vi "HandleObservationAsync_old.vi"(8 "error in (no error)":errorcluster, 10 "Acquisition.lvclass In":refnum<class "Acquisition.lvclass">, 11 "S4ACS_GUI in":refnum<class "S4GUI.lvclass">) -> (0 "error out":errorcluster, 2 "Acquisition.lvclass Out":refnum<class "Acquisition.lvclass">, 3 "S4ACS_GUI out":refnum<class "S4GUI.lvclass">)   [LabVIEW 2018, in "S4GUI.lvclass"]
uses:
  S4GUI.lvclass
  Acquisition/Acquisition.lvclass
  C:/Users/devstaff/sparc4/s4gui/Versao ZeroMQ REQ-REP/SPARC4_GUI -20241016_20241016/Server/Server.lvclass
  S4GUI.lvclass/S4GUI.ctl
  Instrument/Instrument.lvclass/Instrument.ctl
  Device/Optics/Optics.lvclass/Optics.ctl
  Interface/Interface.lvclass/Interface.ctl
  Server/Server.lvclass/Server.ctl
  Device/Optics/Opt_Selector/Opt_Selector.lvclass
  C:/Users/devstaff/sparc4/s4gui/Versao ZeroMQ REQ-REP/SPARC4_GUI -20241016_20241016/Device/Optics/Optics.lvclass
  Instrument/Instrument.lvclass
  StateMachine/State Machine.lvclass
  SyncBox/Sync Box.lvclass
  Trigger/Trigger.lvclass
  Channel/Channel.lvclass
  Interface/Interface.lvclass
  TelFocus/TelFocus.lvclass
  SecMirror/SecMirror.lvclass
  Device/Optics/Optics.lvclass
  Server/Server.lvclass
panel:
  out "time308":u32
  out "time307":u32
  out "time9":u32
  out "delay 89":u32
  out "time 10":u32
  out "time elapsed 2":u32
  out "time 8":u32
  out "delay 78":u32
  out "time7":u32
  out "time6":u32
  out "time5":u32
  out "delay 3-4":u32
  out "time4":u32
  out "time3":u32
  out "time 2":u32
  out "time1":u32
  # "ACS DELAY"
  # "WAVEPLATE DURATION"
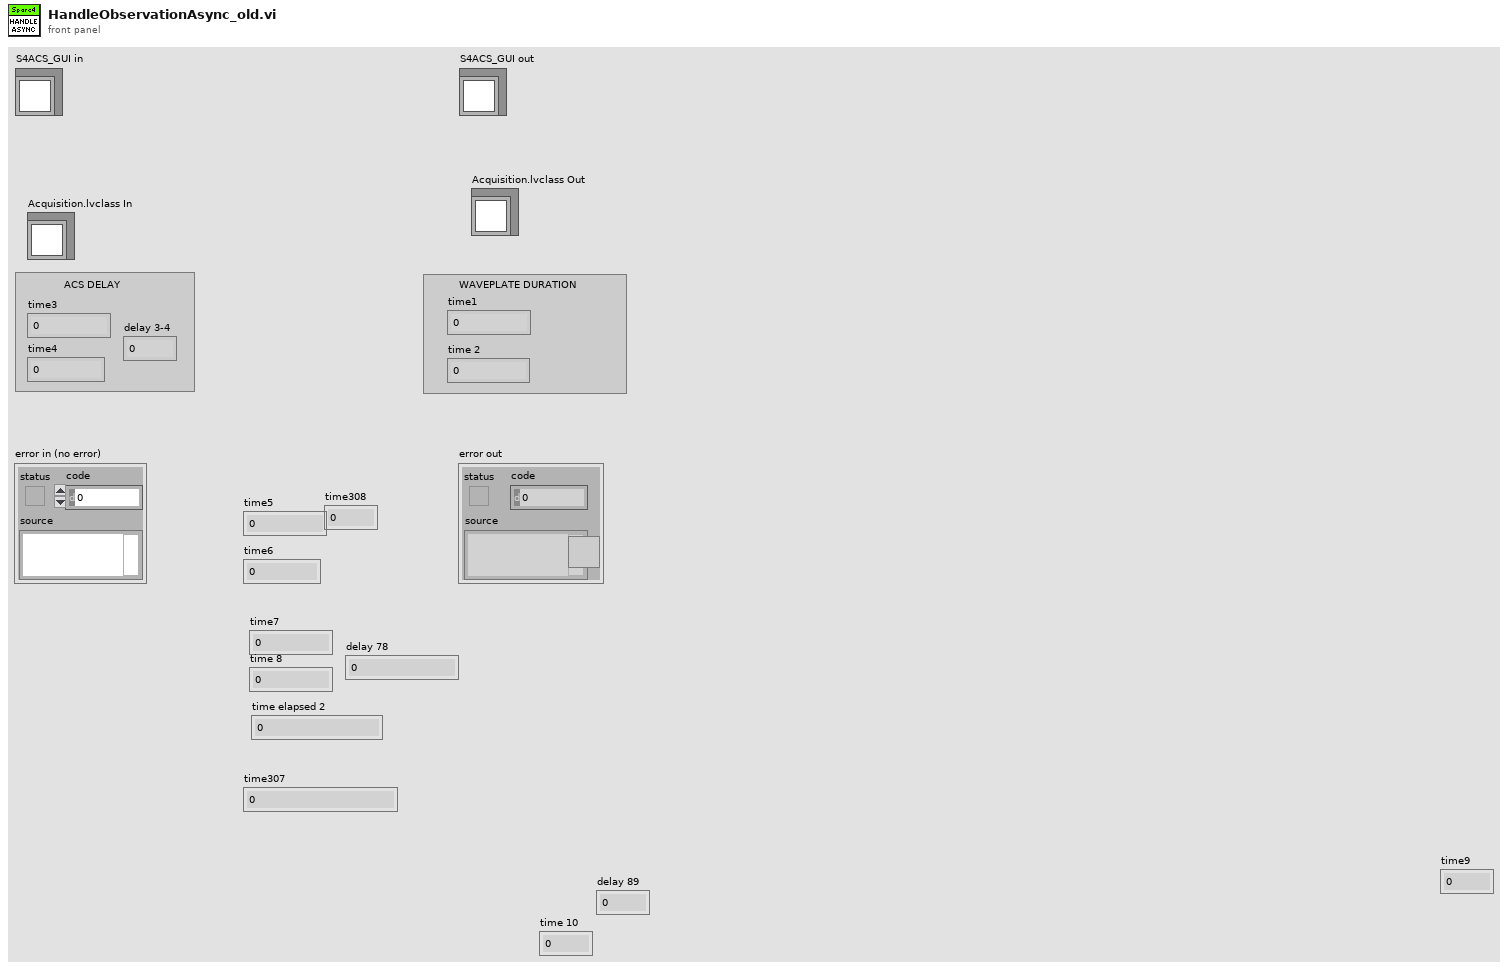
[diagram p1: front panel]
types:
  T1 = cluster{"ACQUISITION_MODE":u8, "TRIGGER_MODE":u8, "READ_MODE":u8, "PREAMP":u8, "READOUT_RATE":u8, "VERTICAL_SHIFT_SPEED":u8, "EM_MODE":u8, "EM_GAIN":u16, "SHUTTER_MODE":u8, "SHUTTER_TTL":u8, "SHUTTER_OPENING_TIME":u16, "SHUTTER_CLOSING_TIME":u16, "VBIN":u16, "HBIN":u16, "INITIAL_LINE":u16, "INITIAL_COLUMN":u16, "FINAL_LINE":u16, "FINAL_COLUMN":u16, "FRAME_TRANSFER":bool, "VERTICAL_CLOCK_VOLTAGE":u8, "AD_CHANNEL":u32}
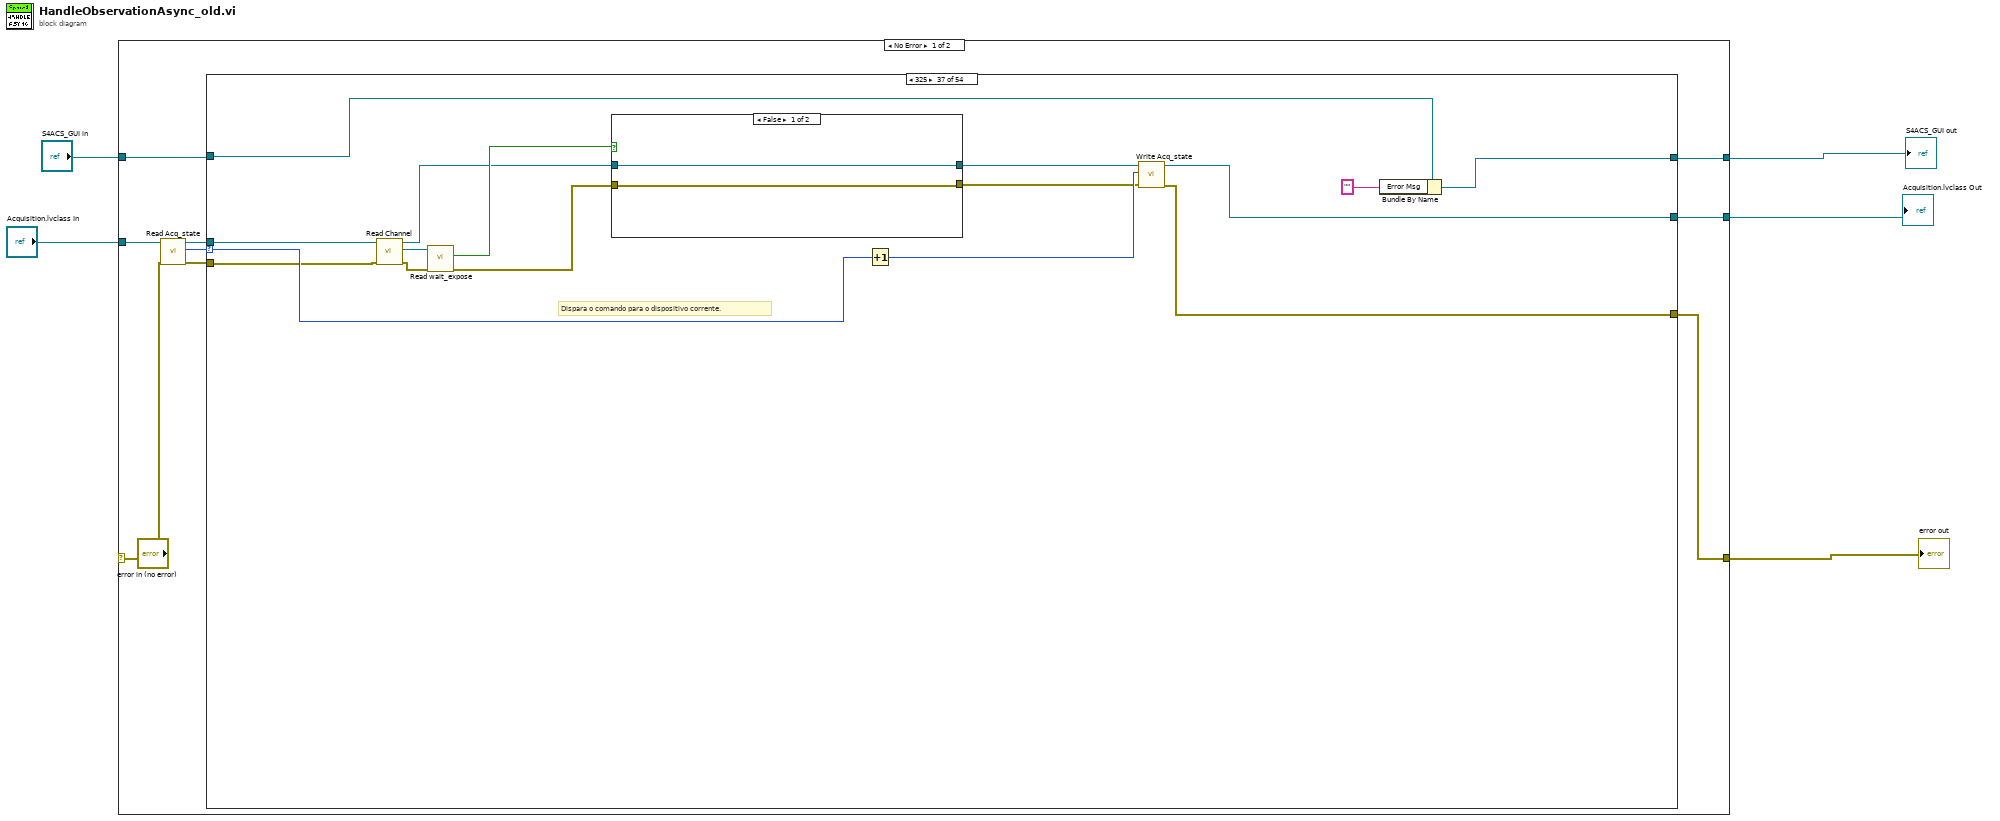
[diagram p0: block diagram]
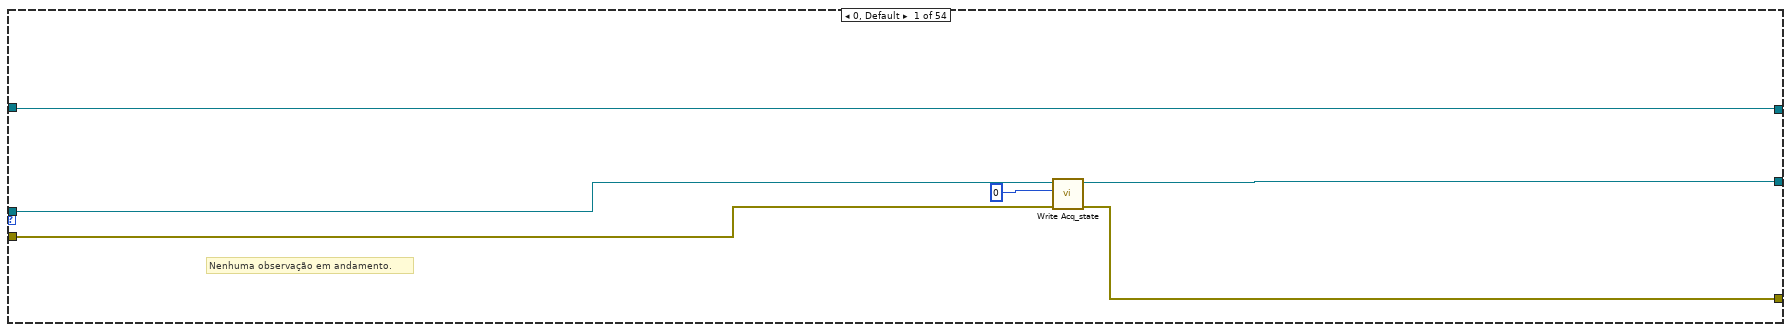
[diagram p2: hidden frame]
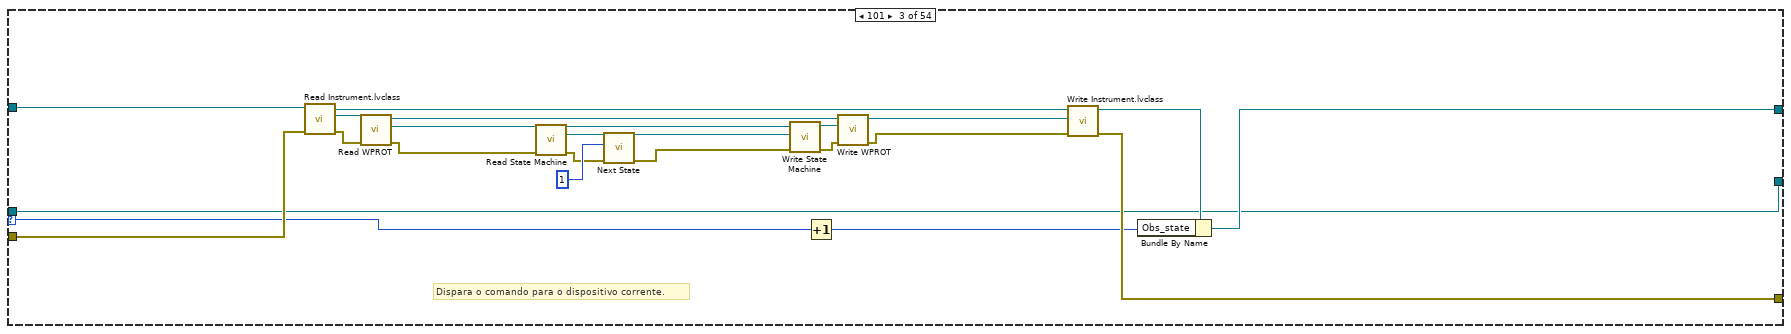
[diagram p4: hidden frame]
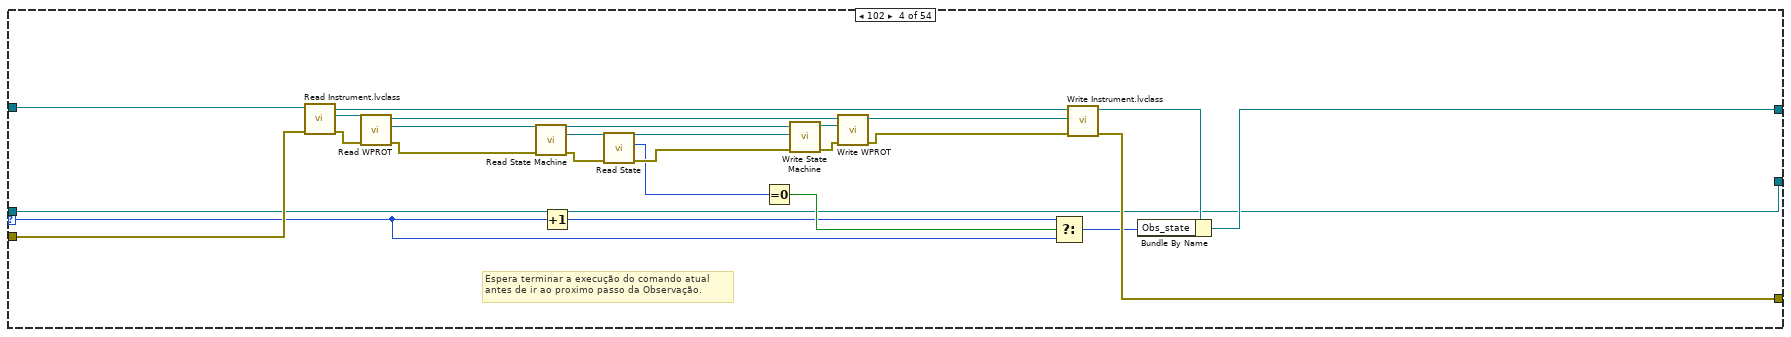
[diagram p5: hidden frame]
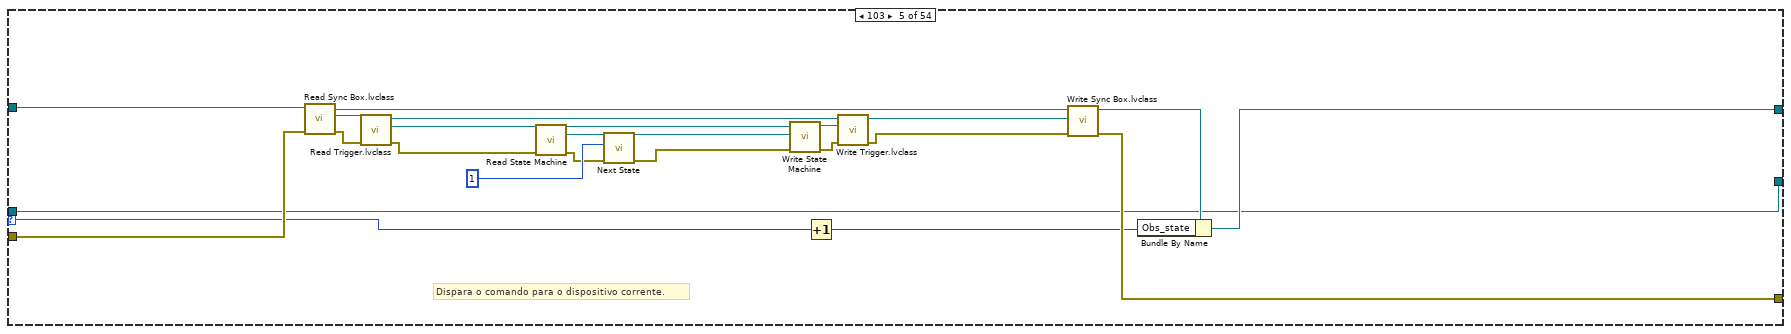
[diagram p6: hidden frame]
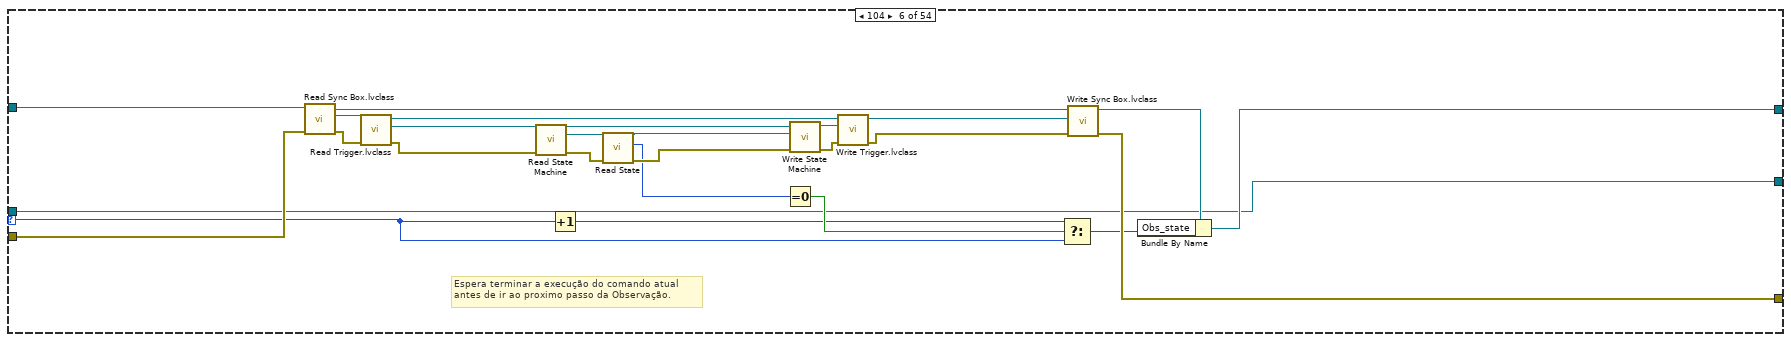
[diagram p7: hidden frame]
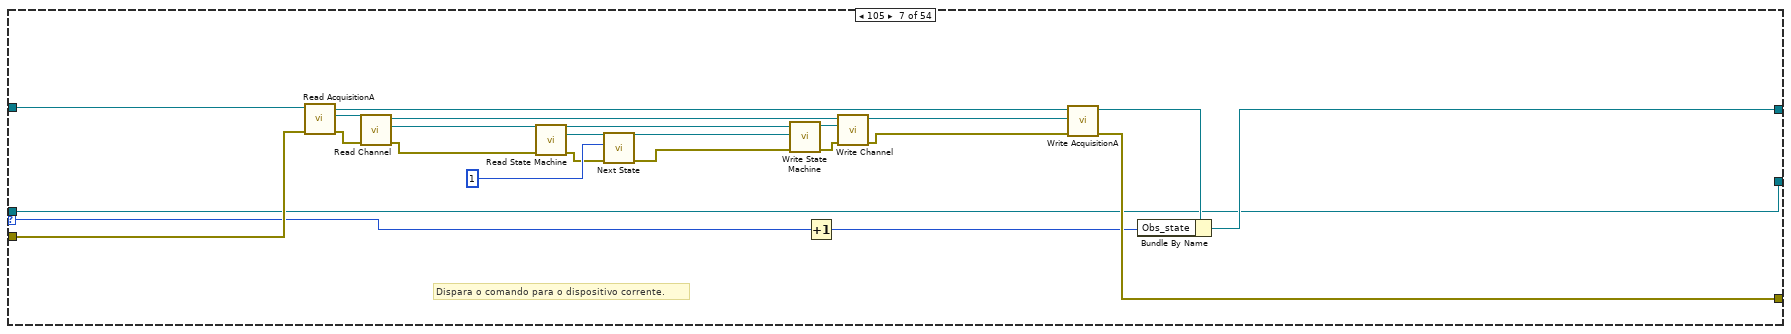
[diagram p8: hidden frame]
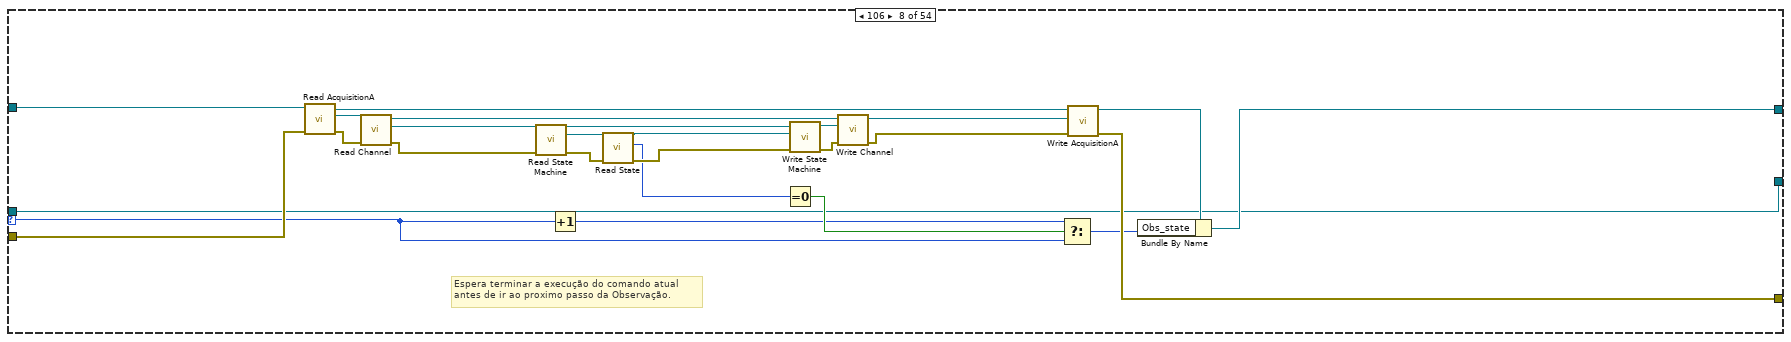
[diagram p9: hidden frame]
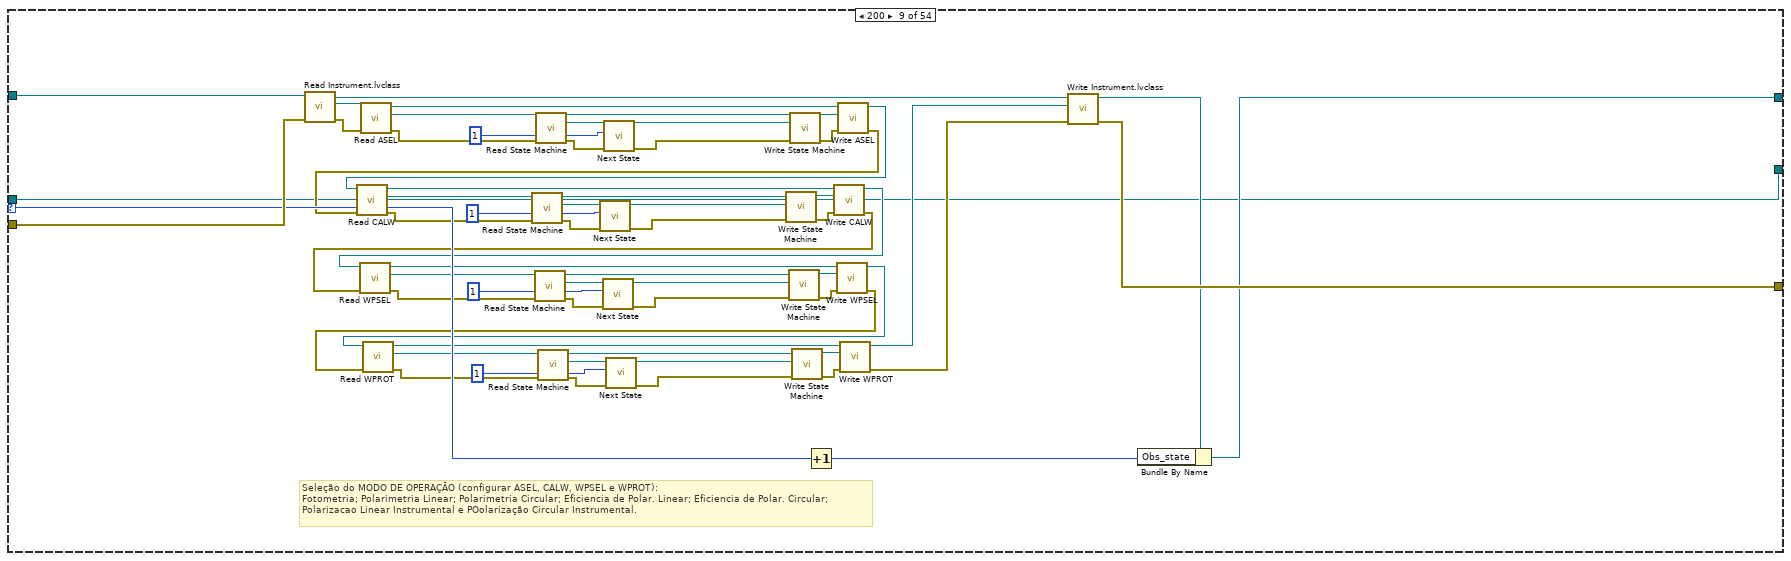
[diagram p10: hidden frame]
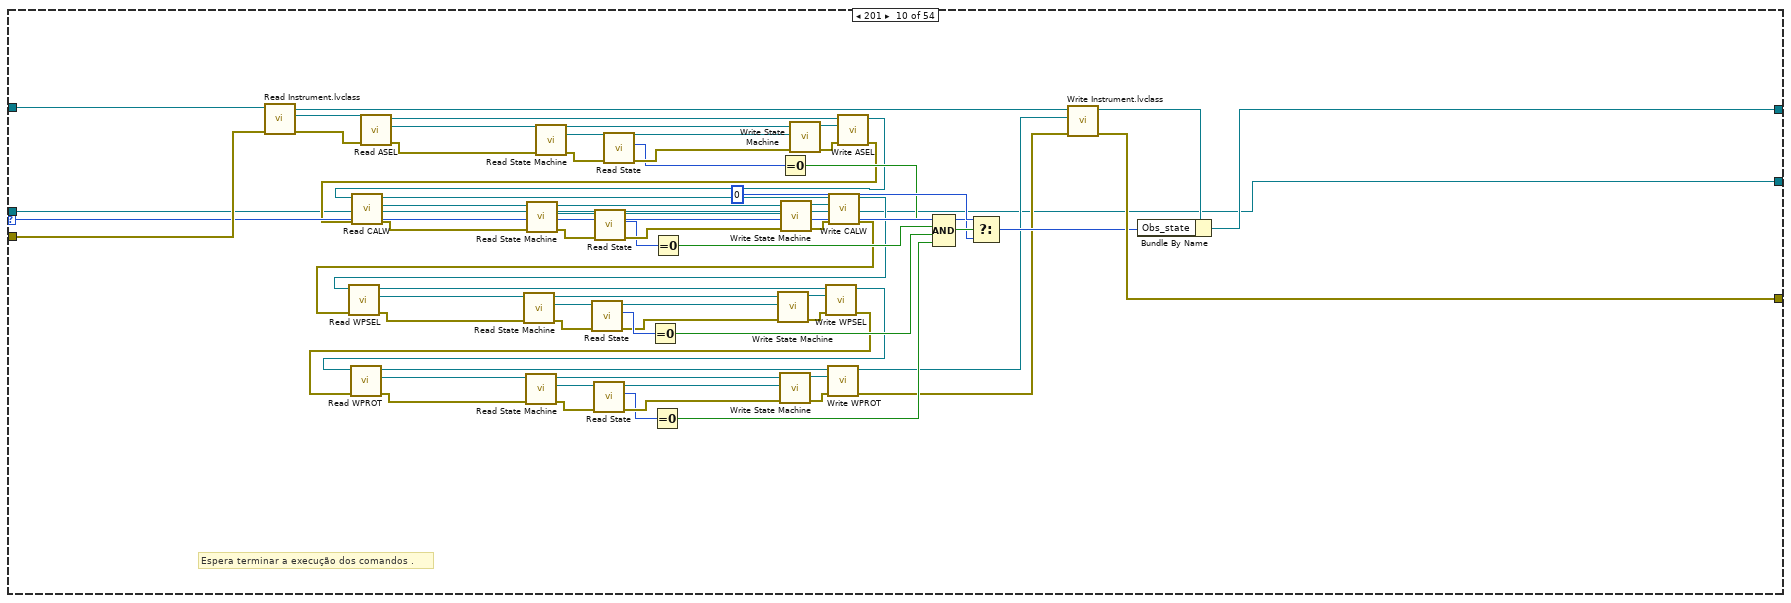
[diagram p11: hidden frame]
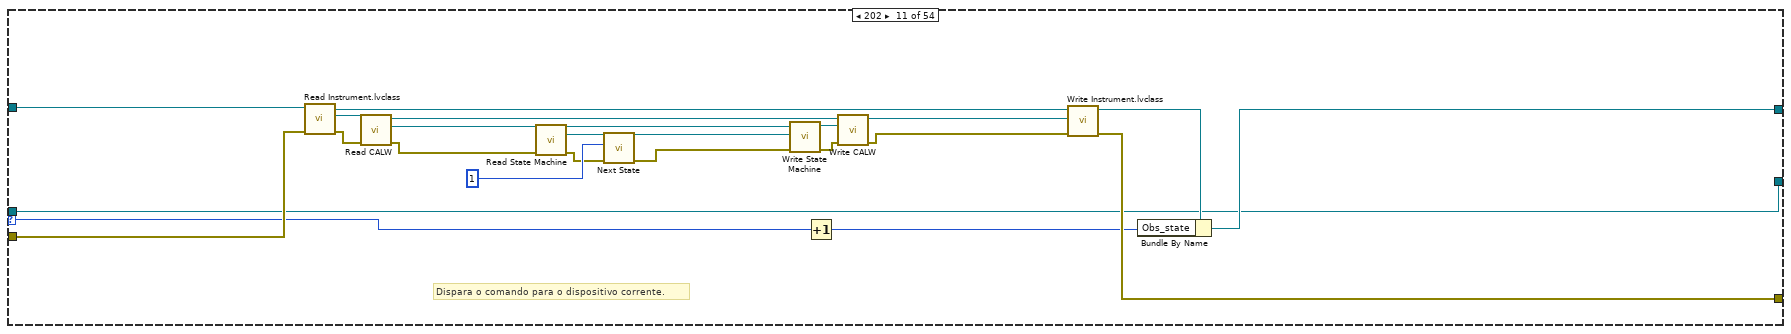
[diagram p12: hidden frame]
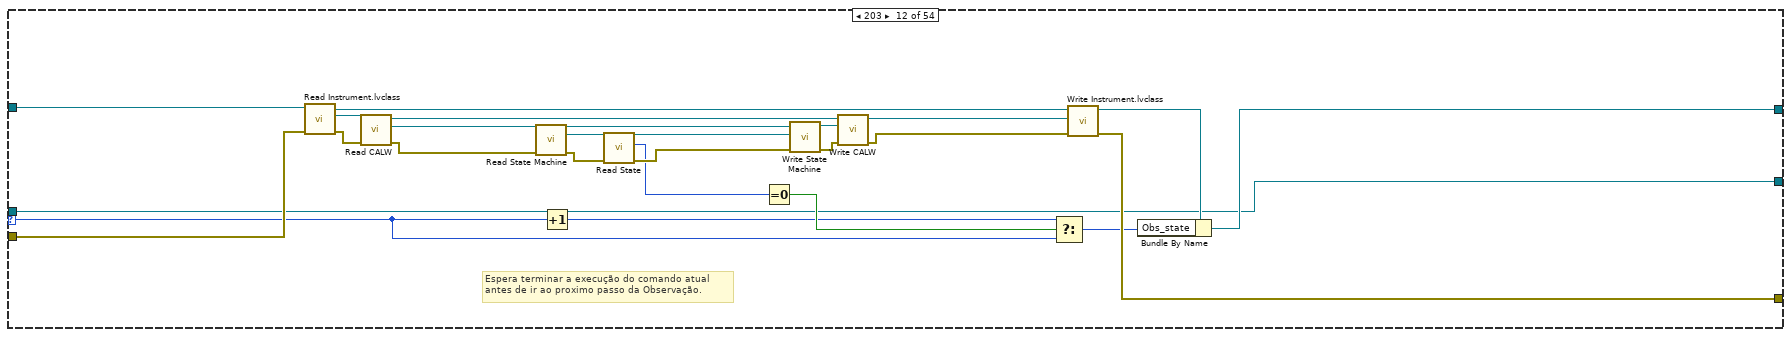
[diagram p13: hidden frame]
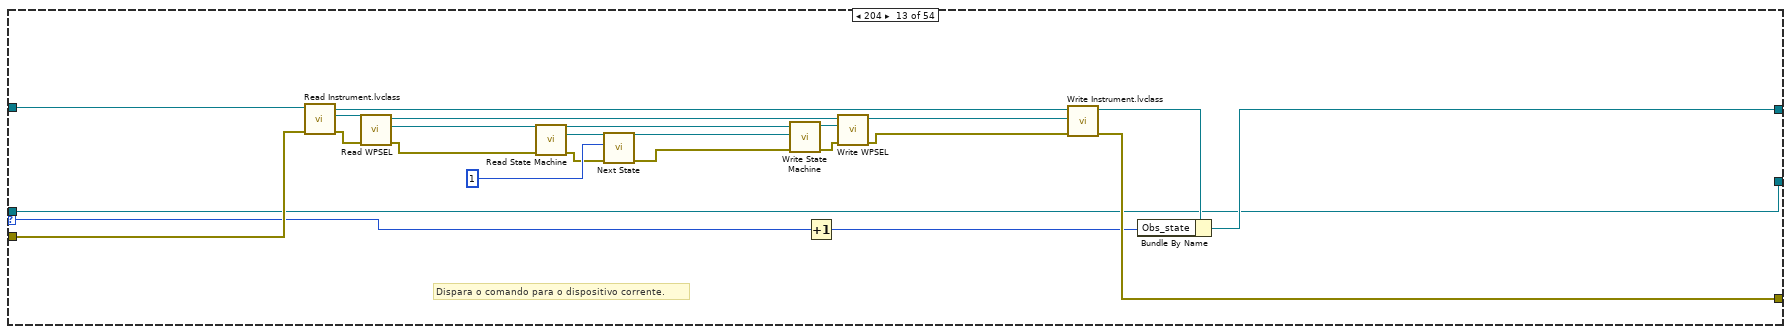
[diagram p14: hidden frame]
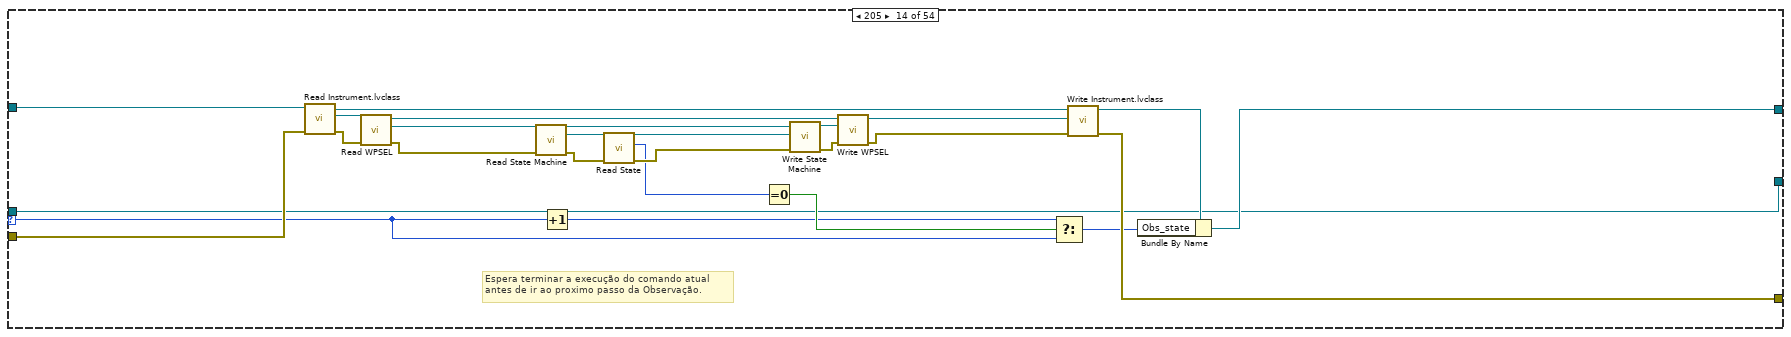
[diagram p15: hidden frame]
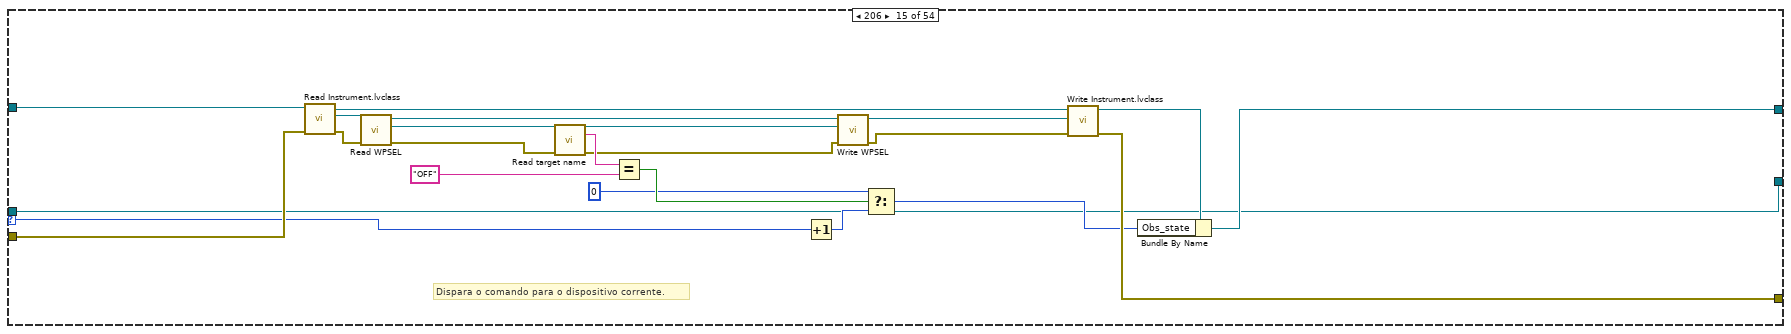
[diagram p16: hidden frame]
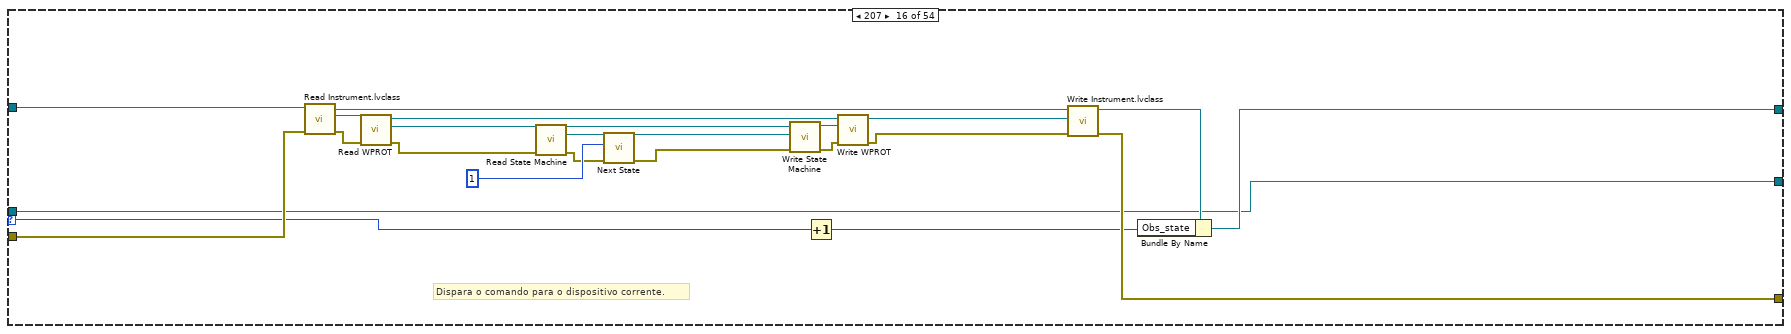
[diagram p17: hidden frame]
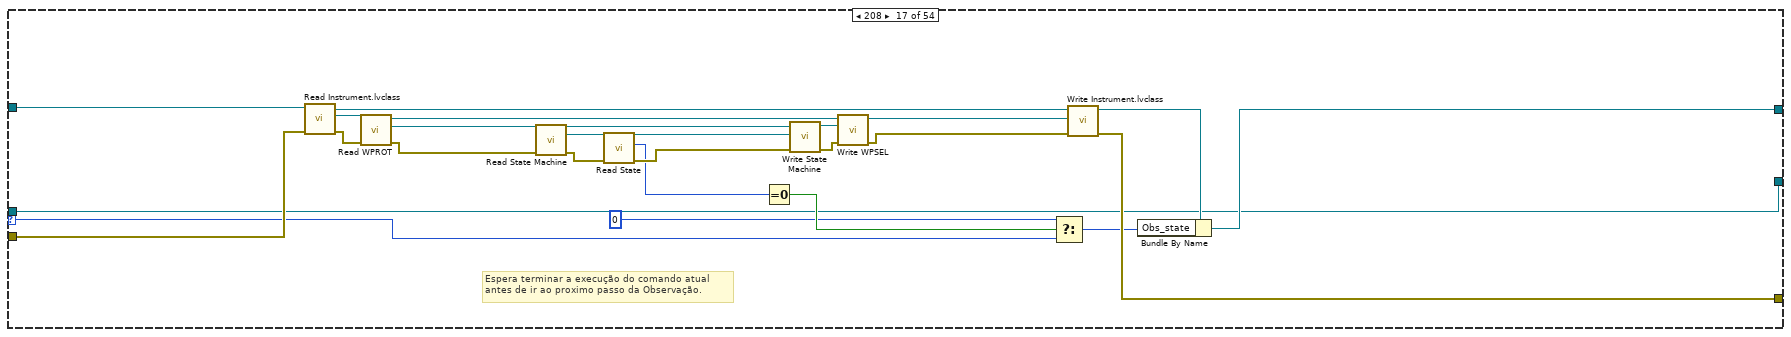
[diagram p18: hidden frame]
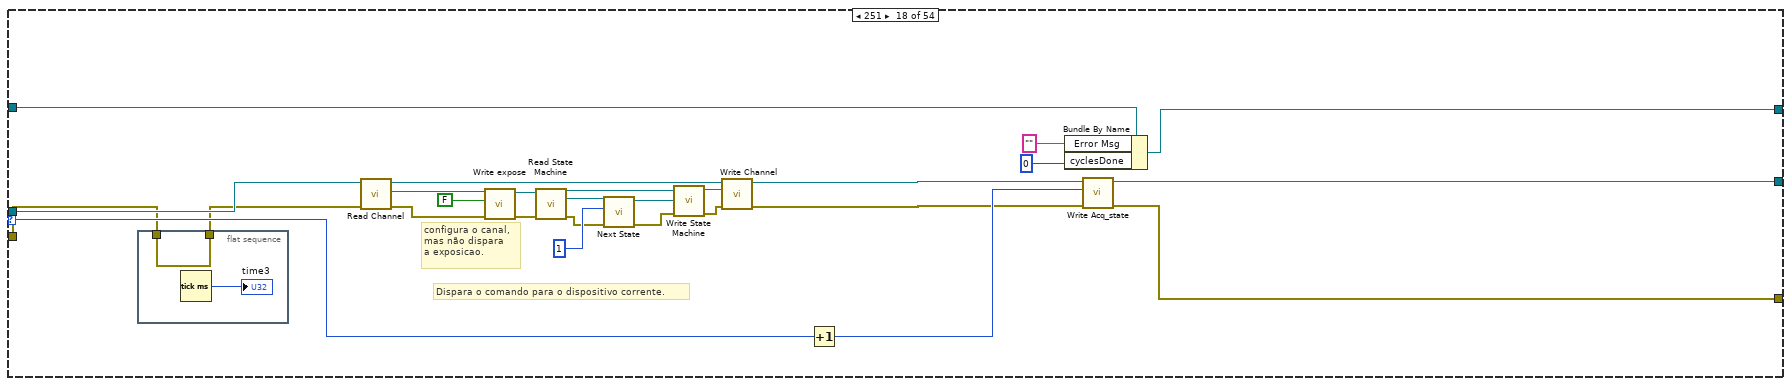
[diagram p19: hidden frame]
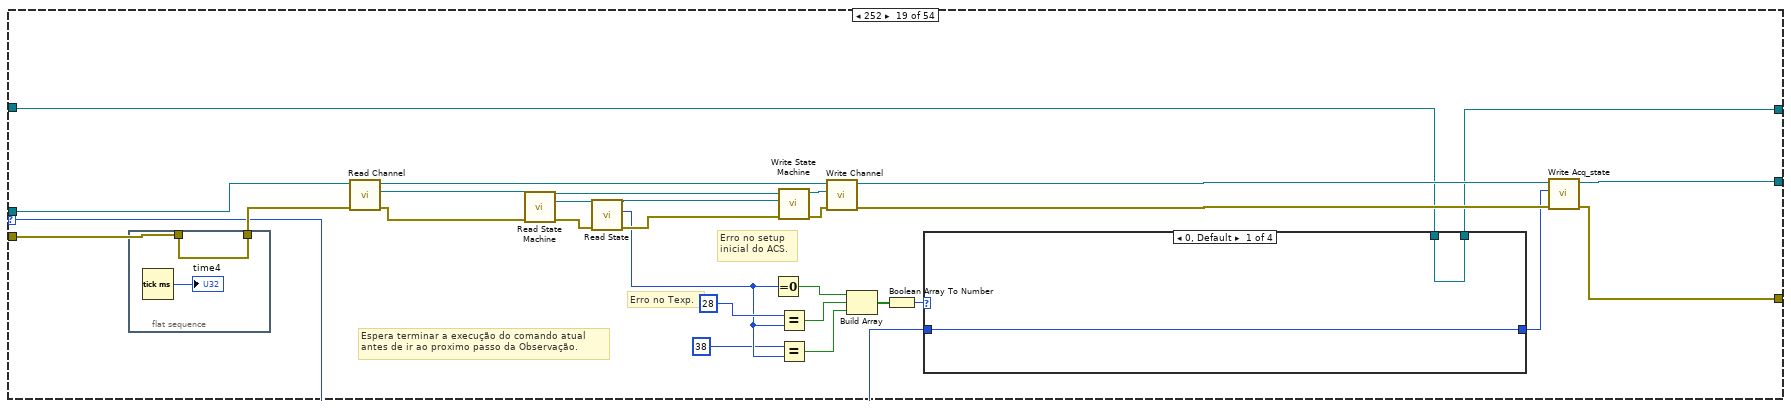
[diagram p20: hidden frame]
diagram:
  n1 = case shown="No Error" "error in (no error)" {
    selector: "error in (no error)" -> [w9 w1768]
    tunnel: [w15 w1768] -> w5
    tunnel: [w14 w1767] -> w3
    tunnel: "S4ACS_GUI in" -> [w13 w1767]
    tunnel: "Acquisition.lvclass In" -> [w12 w1766]
    tunnel: [w7 w1766] -> w1
    frame No Error {
      n2 = call-dynamic "Read Acq_state.vi"("error in (no error)"=w9, "Acquisition in"=w12) -> ("error out"=w8:errorcluster, "Acq_state"=w10:u32, "Acquisition out"=w11:refnum<class "Acquisition.lvclass">)  [unwired: 7 in]
      n3 = case shown="325" w10 {
        selector: w10 -> [_ _ w28 w51 w78 w101 w128 w151 w220 w284 w310 w333 w360 w383 w419 w433 w456 w499 w512 w585 w592 w635 w648 _ w740 w750 w806 w871 w922 w954 w992 _ w1091 w1101 w1129 w1161 w1187 w1207 w1257 w1338 _ w1418 _ w1505 w1554 w1603 w1626 w1642 w1667 w1686 w1711 _ _ _]
        tunnel: w13 -> [w20 w24 w42 w68 w92 w118 w142 w168 w234 w302 w324 w350 w374 w400 w423 w447 w473 w483 w510 w555 w599 w616 w646 w715 w725 w749 w807 w890 w912 w939 w995 w1028 w1081 w1100 w1120 w1144 w1179 w1208 w1252 w1333 w1404 w1417 w1491 w1507 w1556 w1599 w1617 w1648 w1663 w1677 w1704 w1737 w1745 w1748]
        tunnel: [w20 w24 w26 w55 w76 w109 w126 w159 w218 w289 w308 w337 w358 w387 w418 w431 w460 w481 w509 w555 w599 w619 w645 w701 w730 w749 w773 w860 w910 w946 w994 w1027 w1079 w1100 w1119 w1145 w1181 w1211 w1253 w1334 w1404 w1417 w1491 w1504 w1540 w1599 w1621 w1648 w1663 w1681 w1704 w1732 w1745 w1750] -> w14
        tunnel: w8 -> [w19 w23 w41 w67 w91 w117 w141 w167 w233 w301 w323 w349 w373 w399 w422 w446 w472 w485 w522 w556 w593 w622 w658 w706 w724 w763 w770 w877 w920 w934 w1001 w1032 w1089 w1114 w1117 w1155 w1172 w1215 w1237 w1318 w1410 w1421 w1485 w1506 w1555 w1601 w1631 w1645 w1665 w1694 w1724 w1736 w1744 w1747]
        tunnel: [w16 w23 w40 w66 w90 w116 w140 w166 w232 w300 w322 w348 w372 w398 w421 w445 w471 w486 w523 w589 w594 w623 w659 w708 w734 w761 w772 w881 w915 w957 w999 w1029 w1084 w1112 w1123 w1158 w1182 w1218 w1240 w1321 w1415 w1419 w1492 w1498 w1536 w1592 w1627 w1646 w1659 w1690 w1720 w1730 w1744 w1749] -> w15
        tunnel: w11 -> [w18 w22 w25 w49 w75 w99 w125 w149 w175 w238 w307 w331 w357 w381 w407 w430 w454 w491 w527 w588 w600 w627 w663 w700 w739 w764 w775 w859 w921 w961 w1002 w1031 w1090 w1115 w1128 w1154 w1177 w1214 w1238 w1319 w1411 w1422 w1486 w1502 w1539 w1602 w1632 w1643 w1666 w1695 w1725 w1735 w1743 w1746]
        tunnel: [w17 w22 w25 w49 w75 w99 w125 w149 w175 w238 w307 w331 w357 w381 w407 w430 w454 w488 w524 w590 w595 w624 w660 w707 w735 w762 w771 w880 w916 w958 w1000 w1030 w1085 w1113 w1127 w1160 w1186 w1220 w1256 w1337 w1416 w1420 w1493 w1501 w1537 w1596 w1628 w1647 w1660 w1691 w1721 w1731 w1743 w1746] -> w7
        frame 0, Default {
          # "Nenhuma observação em andamento."
          n4 = call-dynamic "Write Acq_state.vi"("error in (no error)"=w19, "Acq_state"=u32 0 ("Obs_state"), "Acquisition in"=w18) -> ("error out"=w16:errorcluster, "Acquisition out"=w17:refnum<class "Acquisition.lvclass">)  [unwired: 7 in]
        }
        frame 1 {
          # "Estado de erro!\nFica aqui até acionar STOP ou ABORT."
          # "Nenhuma observação em andamento."
        }
        frame 101 {
          # "Dispara o comando para o dispositivo corrente."
          n5 = call "Read Instrument.lvclass.vi"("error in (no error)"=w41, "S4ACS_GUI in"=w42) -> ("error out"=w47:errorcluster, "Instrument.lvclass"=w48:refnum<class "Instrument.lvclass">, "S4ACS_GUI out"=w44:refnum<class "S4GUI.lvclass">)  [unwired: 7 in]
          n6 = call "Read WPROT.vi"("error in (no error)"=w47, "Instrument in"=w48) -> ("error out"=w34:errorcluster, "Opt_Selector.lvclass"=w33:refnum<class "Opt_Selector.lvclass">, "Instrument out"=w46:refnum<class "Instrument.lvclass">)  [unwired: 7 in]
          n7 = call-dynamic "Read State Machine.vi"("error in (no error)"=w34, "Device in"=w33) -> ("error out"=w37:errorcluster, "State Machine.lvclass"=w39:refnum<class "State Machine.lvclass">, "Device out"=w31:refnum<class "Opt_Selector.lvclass">)  [unwired: 7 in]
          n8 = call "Next State.vi"("error in (no error)"=w37, "New_State"=1, "State Machine in"=w39) -> ("error out"=w36:errorcluster, "State Machine out"=w35:refnum<class "State Machine.lvclass">)  [unwired: 7 in]
          n9 = call-dynamic "Write State Machine.vi"("error in (no error)"=w36, "State Machine.lvclass"=w35, "Device in"=w31) -> ("error out"=w30:errorcluster, "Device out"=w32:refnum<class "Opt_Selector.lvclass">)  [unwired: 7 in]
          n10 = Increment(x=w28) -> (x+1=w27:u32)
          n11 = call "Write WPROT.vi"("error in (no error)"=w30, "Opt_Selector.lvclass"=w32, "Instrument in"=w46) -> ("error out"=w43:errorcluster, "Instrument out"=w45:refnum<class "Instrument.lvclass">)  [unwired: 7 in]
          n12 = call "Write Instrument.lvclass.vi"("error in (no error)"=w43, "Instrument.lvclass"=w45, "S4ACS_GUI in"=w44) -> ("error out"=w40:errorcluster, "S4ACS_GUI out"=w29:refnum<class "S4GUI.lvclass">)  [unwired: 7 in]
          n13 = Bundle By Name(cluster=w29, "Obs_state"=w27) -> (w26:refnum<class "S4GUI.lvclass">)
        }
        frame 102 {
          # "Espera terminar a execução do comando atual \nantes de ir ao proximo passo da Observação."
          n14 = call "Read Instrument.lvclass.vi"("error in (no error)"=w67, "S4ACS_GUI in"=w68) -> ("error out"=w73:errorcluster, "Instrument.lvclass"=w74:refnum<class "Instrument.lvclass">, "S4ACS_GUI out"=w70:refnum<class "S4GUI.lvclass">)  [unwired: 7 in]
          n15 = call "Read WPROT.vi"("error in (no error)"=w73, "Instrument in"=w74) -> ("error out"=w61:errorcluster, "Opt_Selector.lvclass"=w60:refnum<class "Opt_Selector.lvclass">, "Instrument out"=w72:refnum<class "Instrument.lvclass">)  [unwired: 7 in]
          n16 = call-dynamic "Read State Machine.vi"("error in (no error)"=w61, "Device in"=w60) -> ("error out"=w64:errorcluster, "State Machine.lvclass"=w65:refnum<class "State Machine.lvclass">, "Device out"=w58:refnum<class "Opt_Selector.lvclass">)  [unwired: 7 in]
          n17 = Increment(x=w51) -> (x+1=w50:u32)
          n18 = call-dynamic "Read State.vi"("error in (no error)"=w64, "State Machine in"=w65) -> ("error out"=w63:errorcluster, "State"=w53:i32, "State Machine out"=w62:refnum<class "State Machine.lvclass">)  [unwired: 7 in]
          n19 = Equal To 0?(x=w53) -> (x = 0?=w54:bool)
          n20 = call-dynamic "Write State Machine.vi"("error in (no error)"=w63, "State Machine.lvclass"=w62, "Device in"=w58) -> ("error out"=w57:errorcluster, "Device out"=w59:refnum<class "Opt_Selector.lvclass">)  [unwired: 7 in]
          n21 = call "Write WPROT.vi"("error in (no error)"=w57, "Opt_Selector.lvclass"=w59, "Instrument in"=w72) -> ("error out"=w69:errorcluster, "Instrument out"=w71:refnum<class "Instrument.lvclass">)  [unwired: 7 in]
          n22 = Select(t=w50, s=w54, f=w51) -> (s? t:f=w52:u32)
          n23 = call "Write Instrument.lvclass.vi"("error in (no error)"=w69, "Instrument.lvclass"=w71, "S4ACS_GUI in"=w70) -> ("error out"=w66:errorcluster, "S4ACS_GUI out"=w56:refnum<class "S4GUI.lvclass">)  [unwired: 7 in]
          n24 = Bundle By Name(cluster=w56, "Obs_state"=w52) -> (w55:refnum<class "S4GUI.lvclass">)
        }
        frame 103 {
          # "Dispara o comando para o dispositivo corrente."
          n25 = call-dynamic "Read Sync Box.lvclass.vi"("error in (no error)"=w91, "SPARC4_AC in"=w92) -> ("error out"=w97:errorcluster, "Sync Box.lvclass"=w98:refnum<class "Sync Box.lvclass">, "SPARC4_AC out"=w94:refnum<class "S4GUI.lvclass">)  [unwired: 7 in]
          n26 = call-dynamic "Read Trigger.lvclass.vi"("error in (no error)"=w97, "Sync Box in"=w98) -> ("error out"=w84:errorcluster, "Trigger.lvclass"=w83:refnum<class "Trigger.lvclass">, "Sync Box out"=w96:refnum<class "Sync Box.lvclass">)  [unwired: 7 in]
          n27 = call-dynamic "Read State Machine.vi"("error in (no error)"=w84, "Device in"=w83) -> ("error out"=w87:errorcluster, "State Machine.lvclass"=w89:refnum<class "State Machine.lvclass">, "Device out"=w81:refnum<class "Trigger.lvclass">)  [unwired: 7 in]
          n28 = call "Next State.vi"("error in (no error)"=w87, "New_State"=1, "State Machine in"=w89) -> ("error out"=w86:errorcluster, "State Machine out"=w85:refnum<class "State Machine.lvclass">)  [unwired: 7 in]
          n29 = call-dynamic "Write State Machine.vi"("error in (no error)"=w86, "State Machine.lvclass"=w85, "Device in"=w81) -> ("error out"=w80:errorcluster, "Device out"=w82:refnum<class "Trigger.lvclass">)  [unwired: 7 in]
          n30 = Increment(x=w78) -> (x+1=w77:u32)
          n31 = call-dynamic "Write Trigger.lvclass.vi"("error in (no error)"=w80, "Trigger.lvclass"=w82, "Sync Box in"=w96) -> ("error out"=w93:errorcluster, "Sync Box out"=w95:refnum<class "Sync Box.lvclass">)  [unwired: 7 in]
          n32 = call-dynamic "Write Sync Box.lvclass.vi"("error in (no error)"=w93, "Sync Box.lvclass"=w95, "SPARC4_AC in"=w94) -> ("error out"=w90:errorcluster, "SPARC4_AC out"=w79:refnum<class "S4GUI.lvclass">)  [unwired: 7 in]
          n33 = Bundle By Name(cluster=w79, "Obs_state"=w77) -> (w76:refnum<class "S4GUI.lvclass">)
        }
        frame 104 {
          # "Espera terminar a execução do comando atual \nantes de ir ao proximo passo da Observação."
          n34 = call-dynamic "Read Sync Box.lvclass.vi"("error in (no error)"=w117, "SPARC4_AC in"=w118) -> ("error out"=w123:errorcluster, "Sync Box.lvclass"=w124:refnum<class "Sync Box.lvclass">, "SPARC4_AC out"=w120:refnum<class "S4GUI.lvclass">)  [unwired: 7 in]
          n35 = call-dynamic "Read Trigger.lvclass.vi"("error in (no error)"=w123, "Sync Box in"=w124) -> ("error out"=w115:errorcluster, "Trigger.lvclass"=w114:refnum<class "Trigger.lvclass">, "Sync Box out"=w122:refnum<class "Sync Box.lvclass">)  [unwired: 7 in]
          n36 = call-dynamic "Read State Machine.vi"("error in (no error)"=w115, "Device in"=w114) -> ("error out"=w106:errorcluster, "State Machine.lvclass"=w108:refnum<class "State Machine.lvclass">, "Device out"=w112:refnum<class "Trigger.lvclass">)  [unwired: 7 in]
          n37 = Increment(x=w101) -> (x+1=w103:u32)
          n38 = call-dynamic "Read State.vi"("error in (no error)"=w106, "State Machine in"=w108) -> ("error out"=w105:errorcluster, "State"=w100:i32, "State Machine out"=w107:refnum<class "State Machine.lvclass">)  [unwired: 7 in]
          n39 = Equal To 0?(x=w100) -> (x = 0?=w104:bool)
          n40 = call-dynamic "Write State Machine.vi"("error in (no error)"=w105, "State Machine.lvclass"=w107, "Device in"=w112) -> ("error out"=w111:errorcluster, "Device out"=w113:refnum<class "Trigger.lvclass">)  [unwired: 7 in]
          n41 = call-dynamic "Write Trigger.lvclass.vi"("error in (no error)"=w111, "Trigger.lvclass"=w113, "Sync Box in"=w122) -> ("error out"=w119:errorcluster, "Sync Box out"=w121:refnum<class "Sync Box.lvclass">)  [unwired: 7 in]
          n42 = Select(t=w103, s=w104, f=w101) -> (s? t:f=w102:u32)
          n43 = call-dynamic "Write Sync Box.lvclass.vi"("error in (no error)"=w119, "Sync Box.lvclass"=w121, "SPARC4_AC in"=w120) -> ("error out"=w116:errorcluster, "SPARC4_AC out"=w110:refnum<class "S4GUI.lvclass">)  [unwired: 7 in]
          n44 = Bundle By Name(cluster=w110, "Obs_state"=w102) -> (w109:refnum<class "S4GUI.lvclass">)
        }
        frame 105 {
          # "Dispara o comando para o dispositivo corrente."
          n45 = call-dynamic "Read AcquisitionA.vi"("error in (no error)"=w141, "S4ACS_GUI in"=w142) -> ("error out"=w147:errorcluster, "Acquisition.lvclass"=w148:refnum<class "Acquisition.lvclass">, "S4ACS_GUI out"=w144:refnum<class "S4GUI.lvclass">)  [unwired: 7 in]
          n46 = call-dynamic "Read Channel.vi"("error in (no error)"=w147, "Acquisition in"=w148) -> ("error out"=w134:errorcluster, "Channel.lvclass"=w133:refnum<class "Channel.lvclass">, "Acquisition out"=w146:refnum<class "Acquisition.lvclass">)  [unwired: 7 in]
          n47 = call-dynamic "Read State Machine.vi"("error in (no error)"=w134, "Device in"=w133) -> ("error out"=w137:errorcluster, "State Machine.lvclass"=w139:refnum<class "State Machine.lvclass">, "Device out"=w131:refnum<class "Channel.lvclass">)  [unwired: 7 in]
          n48 = call "Next State.vi"("error in (no error)"=w137, "New_State"=1, "State Machine in"=w139) -> ("error out"=w136:errorcluster, "State Machine out"=w135:refnum<class "State Machine.lvclass">)  [unwired: 7 in]
          n49 = call-dynamic "Write State Machine.vi"("error in (no error)"=w136, "State Machine.lvclass"=w135, "Device in"=w131) -> ("error out"=w130:errorcluster, "Device out"=w132:refnum<class "Channel.lvclass">)  [unwired: 7 in]
          n50 = Increment(x=w128) -> (x+1=w127:u32)
          n51 = call-dynamic "Write Channel.vi"("error in (no error)"=w130, "Channel.lvclass"=w132, "Acquisition in"=w146) -> ("error out"=w143:errorcluster, "Acquisition out"=w145:refnum<class "Acquisition.lvclass">)  [unwired: 7 in]
          n52 = call-dynamic "Write AcquisitionA.vi"("error in (no error)"=w143, "Acquisition.lvclass"=w145, "S4ACS_GUI in"=w144) -> ("error out"=w140:errorcluster, "S4ACS_GUI out"=w129:refnum<class "S4GUI.lvclass">)  [unwired: 7 in]
          n53 = Bundle By Name(cluster=w129, "Obs_state"=w127) -> (w126:refnum<class "S4GUI.lvclass">)
        }
        frame 106 {
          # "Espera terminar a execução do comando atual \nantes de ir ao proximo passo da Observação."
          n54 = call-dynamic "Read AcquisitionA.vi"("error in (no error)"=w167, "S4ACS_GUI in"=w168) -> ("error out"=w173:errorcluster, "Acquisition.lvclass"=w174:refnum<class "Acquisition.lvclass">, "S4ACS_GUI out"=w170:refnum<class "S4GUI.lvclass">)  [unwired: 7 in]
          n55 = call-dynamic "Read Channel.vi"("error in (no error)"=w173, "Acquisition in"=w174) -> ("error out"=w165:errorcluster, "Channel.lvclass"=w164:refnum<class "Channel.lvclass">, "Acquisition out"=w172:refnum<class "Acquisition.lvclass">)  [unwired: 7 in]
          n56 = call-dynamic "Read State Machine.vi"("error in (no error)"=w165, "Device in"=w164) -> ("error out"=w156:errorcluster, "State Machine.lvclass"=w158:refnum<class "State Machine.lvclass">, "Device out"=w162:refnum<class "Channel.lvclass">)  [unwired: 7 in]
          n57 = Increment(x=w151) -> (x+1=w153:u32)
          n58 = call-dynamic "Read State.vi"("error in (no error)"=w156, "State Machine in"=w158) -> ("error out"=w155:errorcluster, "State"=w150:i32, "State Machine out"=w157:refnum<class "State Machine.lvclass">)  [unwired: 7 in]
          n59 = Equal To 0?(x=w150) -> (x = 0?=w154:bool)
          n60 = call-dynamic "Write State Machine.vi"("error in (no error)"=w155, "State Machine.lvclass"=w157, "Device in"=w162) -> ("error out"=w161:errorcluster, "Device out"=w163:refnum<class "Channel.lvclass">)  [unwired: 7 in]
          n61 = call-dynamic "Write Channel.vi"("error in (no error)"=w161, "Channel.lvclass"=w163, "Acquisition in"=w172) -> ("error out"=w169:errorcluster, "Acquisition out"=w171:refnum<class "Acquisition.lvclass">)  [unwired: 7 in]
          n62 = Select(t=w153, s=w154, f=w151) -> (s? t:f=w152:u32)
          n63 = call-dynamic "Write AcquisitionA.vi"("error in (no error)"=w169, "Acquisition.lvclass"=w171, "S4ACS_GUI in"=w170) -> ("error out"=w166:errorcluster, "S4ACS_GUI out"=w160:refnum<class "S4GUI.lvclass">)  [unwired: 7 in]
          n64 = Bundle By Name(cluster=w160, "Obs_state"=w152) -> (w159:refnum<class "S4GUI.lvclass">)
        }
        frame 200 {
          # "Seleção do MODO DE OPERAÇÃO (configurar ASEL, CALW, WPSEL e WPROT): \nFotometria; Polarimetria Linear; Polarimetria Circular; Eficiencia de Polar. Linear; Eficiencia de Polar. Circular;\nPolarizacao Linear Instrumental e POolarização Circular Instrumental."
          n65 = call "Read Instrument.lvclass.vi"("error in (no error)"=w233, "S4ACS_GUI in"=w234) -> ("error out"=w237:errorcluster, "Instrument.lvclass"=w197:refnum<class "Instrument.lvclass">, "S4ACS_GUI out"=w235:refnum<class "S4GUI.lvclass">)  [unwired: 7 in]
          n66 = call "Read ASEL.vi"("error in (no error)"=w237, "Instrument in"=w197) -> ("error out"=w226:errorcluster, "Opt_Selector.lvclass"=w225:refnum<class "Opt_Selector.lvclass">, "Instrument out"=w236:refnum<class "Instrument.lvclass">)  [unwired: 7 in]
          n67 = call-dynamic "Read State Machine.vi"("error in (no error)"=w226, "Device in"=w225) -> ("error out"=w229:errorcluster, "State Machine.lvclass"=w231:refnum<class "State Machine.lvclass">, "Device out"=w223:refnum<class "Opt_Selector.lvclass">)  [unwired: 7 in]
          n68 = call "Next State.vi"("error in (no error)"=w229, "New_State"=1, "State Machine in"=w231) -> ("error out"=w228:errorcluster, "State Machine out"=w227:refnum<class "State Machine.lvclass">)  [unwired: 7 in]
          n69 = call-dynamic "Write State Machine.vi"("error in (no error)"=w228, "State Machine.lvclass"=w227, "Device in"=w223) -> ("error out"=w222:errorcluster, "Device out"=w224:refnum<class "Opt_Selector.lvclass">)  [unwired: 7 in]
          n70 = Increment(x=w220) -> (x+1=w219:u32)
          n71 = call "Write ASEL.vi"("error in (no error)"=w222, "Opt_Selector.lvclass"=w224, "Instrument in"=w236) -> ("error out"=w178:errorcluster, "Instrument out"=w196:refnum<class "Instrument.lvclass">)  [unwired: 7 in]
          n72 = call "Read CALW.vi"("error in (no error)"=w178, "Instrument in"=w196) -> ("error out"=w213:errorcluster, "Opt_Selector.lvclass"=w214:refnum<class "Opt_Selector.lvclass">, "Instrument out"=w195:refnum<class "Instrument.lvclass">)  [unwired: 7 in]
          n73 = call-dynamic "Read State Machine.vi"("error in (no error)"=w213, "Device in"=w214) -> ("error out"=w210:errorcluster, "State Machine.lvclass"=w208:refnum<class "State Machine.lvclass">, "Device out"=w216:refnum<class "Opt_Selector.lvclass">)  [unwired: 7 in]
          n74 = call "Next State.vi"("error in (no error)"=w210, "New_State"=1, "State Machine in"=w208) -> ("error out"=w211:errorcluster, "State Machine out"=w212:refnum<class "State Machine.lvclass">)  [unwired: 7 in]
          n75 = call-dynamic "Write State Machine.vi"("error in (no error)"=w211, "State Machine.lvclass"=w212, "Device in"=w216) -> ("error out"=w217:errorcluster, "Device out"=w215:refnum<class "Opt_Selector.lvclass">)  [unwired: 7 in]
          n76 = call "Write CALW.vi"("error in (no error)"=w217, "Opt_Selector.lvclass"=w215, "Instrument in"=w195) -> ("error out"=w177:errorcluster, "Instrument out"=w194:refnum<class "Instrument.lvclass">)  [unwired: 7 in]
          n77 = call "Read WPSEL.vi"("error in (no error)"=w177, "Instrument in"=w194) -> ("error out"=w202:errorcluster, "Opt_Selector.lvclass"=w201:refnum<class "Opt_Selector.lvclass">, "Instrument out"=w193:refnum<class "Instrument.lvclass">)  [unwired: 7 in]
          n78 = call-dynamic "Read State Machine.vi"("error in (no error)"=w202, "Device in"=w201) -> ("error out"=w205:errorcluster, "State Machine.lvclass"=w207:refnum<class "State Machine.lvclass">, "Device out"=w199:refnum<class "Opt_Selector.lvclass">)  [unwired: 7 in]
          n79 = call "Next State.vi"("error in (no error)"=w205, "New_State"=1, "State Machine in"=w207) -> ("error out"=w204:errorcluster, "State Machine out"=w203:refnum<class "State Machine.lvclass">)  [unwired: 7 in]
          n80 = call-dynamic "Write State Machine.vi"("error in (no error)"=w204, "State Machine.lvclass"=w203, "Device in"=w199) -> ("error out"=w198:errorcluster, "Device out"=w200:refnum<class "Opt_Selector.lvclass">)  [unwired: 7 in]
          n81 = call "Write WPSEL.vi"("error in (no error)"=w198, "Opt_Selector.lvclass"=w200, "Instrument in"=w193) -> ("error out"=w176:errorcluster, "Instrument out"=w182:refnum<class "Instrument.lvclass">)  [unwired: 7 in]
          n82 = call "Read WPROT.vi"("error in (no error)"=w176, "Instrument in"=w182) -> ("error out"=w188:errorcluster, "Opt_Selector.lvclass"=w189:refnum<class "Opt_Selector.lvclass">, "Instrument out"=w181:refnum<class "Instrument.lvclass">)  [unwired: 7 in]
          n83 = call-dynamic "Read State Machine.vi"("error in (no error)"=w188, "Device in"=w189) -> ("error out"=w185:errorcluster, "State Machine.lvclass"=w183:refnum<class "State Machine.lvclass">, "Device out"=w191:refnum<class "Opt_Selector.lvclass">)  [unwired: 7 in]
          n84 = call "Next State.vi"("error in (no error)"=w185, "New_State"=1, "State Machine in"=w183) -> ("error out"=w186:errorcluster, "State Machine out"=w187:refnum<class "State Machine.lvclass">)  [unwired: 7 in]
          n85 = call-dynamic "Write State Machine.vi"("error in (no error)"=w186, "State Machine.lvclass"=w187, "Device in"=w191) -> ("error out"=w192:errorcluster, "Device out"=w190:refnum<class "Opt_Selector.lvclass">)  [unwired: 7 in]
          n86 = call "Write WPROT.vi"("error in (no error)"=w192, "Opt_Selector.lvclass"=w190, "Instrument in"=w181) -> ("error out"=w179:errorcluster, "Instrument out"=w180:refnum<class "Instrument.lvclass">)  [unwired: 7 in]
          n87 = call "Write Instrument.lvclass.vi"("error in (no error)"=w179, "Instrument.lvclass"=w180, "S4ACS_GUI in"=w235) -> ("error out"=w232:errorcluster, "S4ACS_GUI out"=w221:refnum<class "S4GUI.lvclass">)  [unwired: 7 in]
          n88 = Bundle By Name(cluster=w221, "Obs_state"=w219) -> (w218:refnum<class "S4GUI.lvclass">)
        }
        frame 201 {
          # "Espera terminar a execução dos comandos ."
          n89 = call "Read Instrument.lvclass.vi"("error in (no error)"=w301, "S4ACS_GUI in"=w302) -> ("error out"=w305:errorcluster, "Instrument.lvclass"=w306:refnum<class "Instrument.lvclass">, "S4ACS_GUI out"=w303:refnum<class "S4GUI.lvclass">)  [unwired: 7 in]
          n90 = call "Read ASEL.vi"("error in (no error)"=w305, "Instrument in"=w306) -> ("error out"=w295:errorcluster, "Opt_Selector.lvclass"=w294:refnum<class "Opt_Selector.lvclass">, "Instrument out"=w304:refnum<class "Instrument.lvclass">)  [unwired: 7 in]
          n91 = call-dynamic "Read State Machine.vi"("error in (no error)"=w295, "Device in"=w294) -> ("error out"=w298:errorcluster, "State Machine.lvclass"=w299:refnum<class "State Machine.lvclass">, "Device out"=w292:refnum<class "Opt_Selector.lvclass">)  [unwired: 7 in]
          n92 = call-dynamic "Read State.vi"("error in (no error)"=w298, "State Machine in"=w299) -> ("error out"=w297:errorcluster, "State"=w288:i32, "State Machine out"=w296:refnum<class "State Machine.lvclass">)  [unwired: 7 in]
          n93 = Equal To 0?(x=w288) -> (x = 0?=w283:bool)
          n94 = call-dynamic "Write State Machine.vi"("error in (no error)"=w297, "State Machine.lvclass"=w296, "Device in"=w292) -> ("error out"=w291:errorcluster, "Device out"=w293:refnum<class "Opt_Selector.lvclass">)  [unwired: 7 in]
          n95 = call "Write ASEL.vi"("error in (no error)"=w291, "Opt_Selector.lvclass"=w293, "Instrument in"=w304) -> ("error out"=w245:errorcluster, "Instrument out"=w246:refnum<class "Instrument.lvclass">)  [unwired: 7 in]
          n96 = call "Read CALW.vi"("error in (no error)"=w245, "Instrument in"=w246) -> ("error out"=w278:errorcluster, "Opt_Selector.lvclass"=w279:refnum<class "Opt_Selector.lvclass">, "Instrument out"=w249:refnum<class "Instrument.lvclass">)  [unwired: 7 in]
          n97 = call-dynamic "Read State Machine.vi"("error in (no error)"=w278, "Device in"=w279) -> ("error out"=w275:errorcluster, "State Machine.lvclass"=w274:refnum<class "State Machine.lvclass">, "Device out"=w281:refnum<class "Opt_Selector.lvclass">)  [unwired: 7 in]
          n98 = call-dynamic "Read State.vi"("error in (no error)"=w275, "State Machine in"=w274) -> ("error out"=w276:errorcluster, "State"=w273:i32, "State Machine out"=w277:refnum<class "State Machine.lvclass">)  [unwired: 7 in]
          n99 = Equal To 0?(x=w273) -> (x = 0?=w272:bool)
          n100 = call-dynamic "Write State Machine.vi"("error in (no error)"=w276, "State Machine.lvclass"=w277, "Device in"=w281) -> ("error out"=w282:errorcluster, "Device out"=w280:refnum<class "Opt_Selector.lvclass">)  [unwired: 7 in]
          n101 = call "Write CALW.vi"("error in (no error)"=w282, "Opt_Selector.lvclass"=w280, "Instrument in"=w249) -> ("error out"=w243:errorcluster, "Instrument out"=w244:refnum<class "Instrument.lvclass">)  [unwired: 7 in]
          n102 = call "Read WPSEL.vi"("error in (no error)"=w243, "Instrument in"=w244) -> ("error out"=w266:errorcluster, "Opt_Selector.lvclass"=w265:refnum<class "Opt_Selector.lvclass">, "Instrument out"=w248:refnum<class "Instrument.lvclass">)  [unwired: 7 in]
          n103 = call-dynamic "Read State Machine.vi"("error in (no error)"=w266, "Device in"=w265) -> ("error out"=w269:errorcluster, "State Machine.lvclass"=w270:refnum<class "State Machine.lvclass">, "Device out"=w263:refnum<class "Opt_Selector.lvclass">)  [unwired: 7 in]
          n104 = call-dynamic "Read State.vi"("error in (no error)"=w269, "State Machine in"=w270) -> ("error out"=w268:errorcluster, "State"=w271:i32, "State Machine out"=w267:refnum<class "State Machine.lvclass">)  [unwired: 7 in]
          n105 = Equal To 0?(x=w271) -> (x = 0?=w251:bool)
          n106 = call-dynamic "Write State Machine.vi"("error in (no error)"=w268, "State Machine.lvclass"=w267, "Device in"=w263) -> ("error out"=w262:errorcluster, "Device out"=w264:refnum<class "Opt_Selector.lvclass">)  [unwired: 7 in]
          n107 = call "Write WPSEL.vi"("error in (no error)"=w262, "Opt_Selector.lvclass"=w264, "Instrument in"=w248) -> ("error out"=w241:errorcluster, "Instrument out"=w242:refnum<class "Instrument.lvclass">)  [unwired: 7 in]
          n108 = call "Read WPROT.vi"("error in (no error)"=w241, "Instrument in"=w242) -> ("error out"=w257:errorcluster, "Opt_Selector.lvclass"=w258:refnum<class "Opt_Selector.lvclass">, "Instrument out"=w247:refnum<class "Instrument.lvclass">)  [unwired: 7 in]
          n109 = call-dynamic "Read State Machine.vi"("error in (no error)"=w257, "Device in"=w258) -> ("error out"=w254:errorcluster, "State Machine.lvclass"=w253:refnum<class "State Machine.lvclass">, "Device out"=w260:refnum<class "Opt_Selector.lvclass">)  [unwired: 7 in]
          n110 = call-dynamic "Read State.vi"("error in (no error)"=w254, "State Machine in"=w253) -> ("error out"=w255:errorcluster, "State"=w252:i32, "State Machine out"=w256:refnum<class "State Machine.lvclass">)  [unwired: 7 in]
          n111 = Equal To 0?(x=w252) -> (x = 0?=w250:bool)
          n112 = call-dynamic "Write State Machine.vi"("error in (no error)"=w255, "State Machine.lvclass"=w256, "Device in"=w260) -> ("error out"=w261:errorcluster, "Device out"=w259:refnum<class "Opt_Selector.lvclass">)  [unwired: 7 in]
          n113 = call "Write WPROT.vi"("error in (no error)"=w261, "Opt_Selector.lvclass"=w259, "Instrument in"=w247) -> ("error out"=w239:errorcluster, "Instrument out"=w240:refnum<class "Instrument.lvclass">)  [unwired: 7 in]
          n114 = Compound Arithmetic op=AND(w283, w272, w251, w250) -> (w285:bool)
          n115 = Select(t=u32 0, s=w285, f=w284) -> (s? t:f=w287:u32)
          n116 = call "Write Instrument.lvclass.vi"("error in (no error)"=w239, "Instrument.lvclass"=w240, "S4ACS_GUI in"=w303) -> ("error out"=w300:errorcluster, "S4ACS_GUI out"=w290:refnum<class "S4GUI.lvclass">)  [unwired: 7 in]
          n117 = Bundle By Name(cluster=w290, "Obs_state"=w287) -> (w289:refnum<class "S4GUI.lvclass">)
        }
        frame 202 {
          # "Dispara o comando para o dispositivo corrente."
          n118 = call "Read Instrument.lvclass.vi"("error in (no error)"=w323, "S4ACS_GUI in"=w324) -> ("error out"=w329:errorcluster, "Instrument.lvclass"=w330:refnum<class "Instrument.lvclass">, "S4ACS_GUI out"=w326:refnum<class "S4GUI.lvclass">)  [unwired: 7 in]
          n119 = call "Read CALW.vi"("error in (no error)"=w329, "Instrument in"=w330) -> ("error out"=w316:errorcluster, "Opt_Selector.lvclass"=w315:refnum<class "Opt_Selector.lvclass">, "Instrument out"=w328:refnum<class "Instrument.lvclass">)  [unwired: 7 in]
          n120 = call-dynamic "Read State Machine.vi"("error in (no error)"=w316, "Device in"=w315) -> ("error out"=w319:errorcluster, "State Machine.lvclass"=w321:refnum<class "State Machine.lvclass">, "Device out"=w313:refnum<class "Opt_Selector.lvclass">)  [unwired: 7 in]
          n121 = call "Next State.vi"("error in (no error)"=w319, "New_State"=1, "State Machine in"=w321) -> ("error out"=w318:errorcluster, "State Machine out"=w317:refnum<class "State Machine.lvclass">)  [unwired: 7 in]
          n122 = call-dynamic "Write State Machine.vi"("error in (no error)"=w318, "State Machine.lvclass"=w317, "Device in"=w313) -> ("error out"=w312:errorcluster, "Device out"=w314:refnum<class "Opt_Selector.lvclass">)  [unwired: 7 in]
          n123 = Increment(x=w310) -> (x+1=w309:u32)
          n124 = call "Write CALW.vi"("error in (no error)"=w312, "Opt_Selector.lvclass"=w314, "Instrument in"=w328) -> ("error out"=w325:errorcluster, "Instrument out"=w327:refnum<class "Instrument.lvclass">)  [unwired: 7 in]
          n125 = call "Write Instrument.lvclass.vi"("error in (no error)"=w325, "Instrument.lvclass"=w327, "S4ACS_GUI in"=w326) -> ("error out"=w322:errorcluster, "S4ACS_GUI out"=w311:refnum<class "S4GUI.lvclass">)  [unwired: 7 in]
          n126 = Bundle By Name(cluster=w311, "Obs_state"=w309) -> (w308:refnum<class "S4GUI.lvclass">)
        }
        frame 203 {
          # "Espera terminar a execução do comando atual \nantes de ir ao proximo passo da Observação."
          n127 = call "Read Instrument.lvclass.vi"("error in (no error)"=w349, "S4ACS_GUI in"=w350) -> ("error out"=w355:errorcluster, "Instrument.lvclass"=w356:refnum<class "Instrument.lvclass">, "S4ACS_GUI out"=w352:refnum<class "S4GUI.lvclass">)  [unwired: 7 in]
          n128 = call "Read CALW.vi"("error in (no error)"=w355, "Instrument in"=w356) -> ("error out"=w343:errorcluster, "Opt_Selector.lvclass"=w342:refnum<class "Opt_Selector.lvclass">, "Instrument out"=w354:refnum<class "Instrument.lvclass">)  [unwired: 7 in]
          n129 = call-dynamic "Read State Machine.vi"("error in (no error)"=w343, "Device in"=w342) -> ("error out"=w346:errorcluster, "State Machine.lvclass"=w347:refnum<class "State Machine.lvclass">, "Device out"=w340:refnum<class "Opt_Selector.lvclass">)  [unwired: 7 in]
          n130 = Increment(x=w333) -> (x+1=w332:u32)
          n131 = call-dynamic "Read State.vi"("error in (no error)"=w346, "State Machine in"=w347) -> ("error out"=w345:errorcluster, "State"=w335:i32, "State Machine out"=w344:refnum<class "State Machine.lvclass">)  [unwired: 7 in]
          n132 = Equal To 0?(x=w335) -> (x = 0?=w336:bool)
          n133 = call-dynamic "Write State Machine.vi"("error in (no error)"=w345, "State Machine.lvclass"=w344, "Device in"=w340) -> ("error out"=w339:errorcluster, "Device out"=w341:refnum<class "Opt_Selector.lvclass">)  [unwired: 7 in]
          n134 = call "Write CALW.vi"("error in (no error)"=w339, "Opt_Selector.lvclass"=w341, "Instrument in"=w354) -> ("error out"=w351:errorcluster, "Instrument out"=w353:refnum<class "Instrument.lvclass">)  [unwired: 7 in]
          n135 = Select(t=w332, s=w336, f=w333) -> (s? t:f=w334:u32)
          n136 = call "Write Instrument.lvclass.vi"("error in (no error)"=w351, "Instrument.lvclass"=w353, "S4ACS_GUI in"=w352) -> ("error out"=w348:errorcluster, "S4ACS_GUI out"=w338:refnum<class "S4GUI.lvclass">)  [unwired: 7 in]
          n137 = Bundle By Name(cluster=w338, "Obs_state"=w334) -> (w337:refnum<class "S4GUI.lvclass">)
        }
        frame 204 {
          # "Dispara o comando para o dispositivo corrente."
          n138 = call "Read Instrument.lvclass.vi"("error in (no error)"=w373, "S4ACS_GUI in"=w374) -> ("error out"=w379:errorcluster, "Instrument.lvclass"=w380:refnum<class "Instrument.lvclass">, "S4ACS_GUI out"=w376:refnum<class "S4GUI.lvclass">)  [unwired: 7 in]
          n139 = call "Read WPSEL.vi"("error in (no error)"=w379, "Instrument in"=w380) -> ("error out"=w366:errorcluster, "Opt_Selector.lvclass"=w365:refnum<class "Opt_Selector.lvclass">, "Instrument out"=w378:refnum<class "Instrument.lvclass">)  [unwired: 7 in]
          n140 = call-dynamic "Read State Machine.vi"("error in (no error)"=w366, "Device in"=w365) -> ("error out"=w369:errorcluster, "State Machine.lvclass"=w371:refnum<class "State Machine.lvclass">, "Device out"=w363:refnum<class "Opt_Selector.lvclass">)  [unwired: 7 in]
          n141 = call "Next State.vi"("error in (no error)"=w369, "New_State"=1, "State Machine in"=w371) -> ("error out"=w368:errorcluster, "State Machine out"=w367:refnum<class "State Machine.lvclass">)  [unwired: 7 in]
          n142 = call-dynamic "Write State Machine.vi"("error in (no error)"=w368, "State Machine.lvclass"=w367, "Device in"=w363) -> ("error out"=w362:errorcluster, "Device out"=w364:refnum<class "Opt_Selector.lvclass">)  [unwired: 7 in]
          n143 = Increment(x=w360) -> (x+1=w359:u32)
          n144 = call "Write WPSEL.vi"("error in (no error)"=w362, "Opt_Selector.lvclass"=w364, "Instrument in"=w378) -> ("error out"=w375:errorcluster, "Instrument out"=w377:refnum<class "Instrument.lvclass">)  [unwired: 7 in]
          n145 = call "Write Instrument.lvclass.vi"("error in (no error)"=w375, "Instrument.lvclass"=w377, "S4ACS_GUI in"=w376) -> ("error out"=w372:errorcluster, "S4ACS_GUI out"=w361:refnum<class "S4GUI.lvclass">)  [unwired: 7 in]
          n146 = Bundle By Name(cluster=w361, "Obs_state"=w359) -> (w358:refnum<class "S4GUI.lvclass">)
        }
        frame 205 {
          # "Espera terminar a execução do comando atual \nantes de ir ao proximo passo da Observação."
          n147 = call "Read Instrument.lvclass.vi"("error in (no error)"=w399, "S4ACS_GUI in"=w400) -> ("error out"=w405:errorcluster, "Instrument.lvclass"=w406:refnum<class "Instrument.lvclass">, "S4ACS_GUI out"=w402:refnum<class "S4GUI.lvclass">)  [unwired: 7 in]
          n148 = call "Read WPSEL.vi"("error in (no error)"=w405, "Instrument in"=w406) -> ("error out"=w393:errorcluster, "Opt_Selector.lvclass"=w392:refnum<class "Opt_Selector.lvclass">, "Instrument out"=w404:refnum<class "Instrument.lvclass">)  [unwired: 7 in]
          n149 = call-dynamic "Read State Machine.vi"("error in (no error)"=w393, "Device in"=w392) -> ("error out"=w396:errorcluster, "State Machine.lvclass"=w397:refnum<class "State Machine.lvclass">, "Device out"=w390:refnum<class "Opt_Selector.lvclass">)  [unwired: 7 in]
          n150 = Increment(x=w383) -> (x+1=w382:u32)
          n151 = call-dynamic "Read State.vi"("error in (no error)"=w396, "State Machine in"=w397) -> ("error out"=w395:errorcluster, "State"=w385:i32, "State Machine out"=w394:refnum<class "State Machine.lvclass">)  [unwired: 7 in]
          n152 = Equal To 0?(x=w385) -> (x = 0?=w386:bool)
          n153 = call-dynamic "Write State Machine.vi"("error in (no error)"=w395, "State Machine.lvclass"=w394, "Device in"=w390) -> ("error out"=w389:errorcluster, "Device out"=w391:refnum<class "Opt_Selector.lvclass">)  [unwired: 7 in]
          n154 = call "Write WPSEL.vi"("error in (no error)"=w389, "Opt_Selector.lvclass"=w391, "Instrument in"=w404) -> ("error out"=w401:errorcluster, "Instrument out"=w403:refnum<class "Instrument.lvclass">)  [unwired: 7 in]
          n155 = Select(t=w382, s=w386, f=w383) -> (s? t:f=w384:u32)
          n156 = call "Write Instrument.lvclass.vi"("error in (no error)"=w401, "Instrument.lvclass"=w403, "S4ACS_GUI in"=w402) -> ("error out"=w398:errorcluster, "S4ACS_GUI out"=w388:refnum<class "S4GUI.lvclass">)  [unwired: 7 in]
          n157 = Bundle By Name(cluster=w388, "Obs_state"=w384) -> (w387:refnum<class "S4GUI.lvclass">)
        }
        frame 206 {
          # "Dispara o comando para o dispositivo corrente."
          n158 = call "Read Instrument.lvclass.vi"("error in (no error)"=w422, "S4ACS_GUI in"=w423) -> ("error out"=w428:errorcluster, "Instrument.lvclass"=w429:refnum<class "Instrument.lvclass">, "S4ACS_GUI out"=w425:refnum<class "S4GUI.lvclass">)  [unwired: 7 in]
          n159 = call "Read WPSEL.vi"("error in (no error)"=w428, "Instrument in"=w429) -> ("error out"=w416:errorcluster, "Opt_Selector.lvclass"=w417:refnum<class "Opt_Selector.lvclass">, "Instrument out"=w427:refnum<class "Instrument.lvclass">)  [unwired: 7 in]
          n160 = call "Read target name.vi"("error in (no error)"=w416, "Optics in"=w417) -> ("error out"=w410:errorcluster, "target name"=w415:string, "Optics out"=w409:refnum<class "Opt_Selector.lvclass">)  [unwired: 7 in]
          n161 = Equal?(x=w415, y="OFF") -> (x = y?=w413:bool)
          n162 = Increment(x=w419) -> (x+1=w411:u32)
          n163 = call "Write WPSEL.vi"("error in (no error)"=w410, "Opt_Selector.lvclass"=w409, "Instrument in"=w427) -> ("error out"=w424:errorcluster, "Instrument out"=w426:refnum<class "Instrument.lvclass">)  [unwired: 7 in]
          n164 = Select(t=u32 0, s=w413, f=w411) -> (s? t:f=w408:u32)
          n165 = call "Write Instrument.lvclass.vi"("error in (no error)"=w424, "Instrument.lvclass"=w426, "S4ACS_GUI in"=w425) -> ("error out"=w421:errorcluster, "S4ACS_GUI out"=w420:refnum<class "S4GUI.lvclass">)  [unwired: 7 in]
          n166 = Bundle By Name(cluster=w420, "Obs_state"=w408) -> (w418:refnum<class "S4GUI.lvclass">)
        }
        frame 207 {
          # "Dispara o comando para o dispositivo corrente."
          n167 = call "Read Instrument.lvclass.vi"("error in (no error)"=w446, "S4ACS_GUI in"=w447) -> ("error out"=w452:errorcluster, "Instrument.lvclass"=w453:refnum<class "Instrument.lvclass">, "S4ACS_GUI out"=w449:refnum<class "S4GUI.lvclass">)  [unwired: 7 in]
          n168 = call "Read WPROT.vi"("error in (no error)"=w452, "Instrument in"=w453) -> ("error out"=w439:errorcluster, "Opt_Selector.lvclass"=w438:refnum<class "Opt_Selector.lvclass">, "Instrument out"=w451:refnum<class "Instrument.lvclass">)  [unwired: 7 in]
          n169 = call-dynamic "Read State Machine.vi"("error in (no error)"=w439, "Device in"=w438) -> ("error out"=w442:errorcluster, "State Machine.lvclass"=w444:refnum<class "State Machine.lvclass">, "Device out"=w436:refnum<class "Opt_Selector.lvclass">)  [unwired: 7 in]
          n170 = call "Next State.vi"("error in (no error)"=w442, "New_State"=1, "State Machine in"=w444) -> ("error out"=w441:errorcluster, "State Machine out"=w440:refnum<class "State Machine.lvclass">)  [unwired: 7 in]
          n171 = call-dynamic "Write State Machine.vi"("error in (no error)"=w441, "State Machine.lvclass"=w440, "Device in"=w436) -> ("error out"=w435:errorcluster, "Device out"=w437:refnum<class "Opt_Selector.lvclass">)  [unwired: 7 in]
          n172 = Increment(x=w433) -> (x+1=w432:u32)
          n173 = call "Write WPROT.vi"("error in (no error)"=w435, "Opt_Selector.lvclass"=w437, "Instrument in"=w451) -> ("error out"=w448:errorcluster, "Instrument out"=w450:refnum<class "Instrument.lvclass">)  [unwired: 7 in]
          n174 = call "Write Instrument.lvclass.vi"("error in (no error)"=w448, "Instrument.lvclass"=w450, "S4ACS_GUI in"=w449) -> ("error out"=w445:errorcluster, "S4ACS_GUI out"=w434:refnum<class "S4GUI.lvclass">)  [unwired: 7 in]
          n175 = Bundle By Name(cluster=w434, "Obs_state"=w432) -> (w431:refnum<class "S4GUI.lvclass">)
        }
        frame 208 {
          # "Espera terminar a execução do comando atual \nantes de ir ao proximo passo da Observação."
          n176 = call "Read Instrument.lvclass.vi"("error in (no error)"=w472, "S4ACS_GUI in"=w473) -> ("error out"=w478:errorcluster, "Instrument.lvclass"=w479:refnum<class "Instrument.lvclass">, "S4ACS_GUI out"=w475:refnum<class "S4GUI.lvclass">)  [unwired: 7 in]
          n177 = call "Read WPROT.vi"("error in (no error)"=w478, "Instrument in"=w479) -> ("error out"=w466:errorcluster, "Opt_Selector.lvclass"=w465:refnum<class "Opt_Selector.lvclass">, "Instrument out"=w477:refnum<class "Instrument.lvclass">)  [unwired: 7 in]
          n178 = call-dynamic "Read State Machine.vi"("error in (no error)"=w466, "Device in"=w465) -> ("error out"=w469:errorcluster, "State Machine.lvclass"=w470:refnum<class "State Machine.lvclass">, "Device out"=w463:refnum<class "Opt_Selector.lvclass">)  [unwired: 7 in]
          n179 = call-dynamic "Read State.vi"("error in (no error)"=w469, "State Machine in"=w470) -> ("error out"=w468:errorcluster, "State"=w458:i32, "State Machine out"=w467:refnum<class "State Machine.lvclass">)  [unwired: 7 in]
          n180 = Equal To 0?(x=w458) -> (x = 0?=w459:bool)
          n181 = call-dynamic "Write State Machine.vi"("error in (no error)"=w468, "State Machine.lvclass"=w467, "Device in"=w463) -> ("error out"=w462:errorcluster, "Device out"=w464:refnum<class "Opt_Selector.lvclass">)  [unwired: 7 in]
          n182 = call "Write WPSEL.vi"("error in (no error)"=w462, "Opt_Selector.lvclass"=w464, "Instrument in"=w477) -> ("error out"=w474:errorcluster, "Instrument out"=w476:refnum<class "Instrument.lvclass">)  [unwired: 7 in]
          n183 = Select(t=u32 0, s=w459, f=w456) -> (s? t:f=w457:u32)
          n184 = call "Write Instrument.lvclass.vi"("error in (no error)"=w474, "Instrument.lvclass"=w476, "S4ACS_GUI in"=w475) -> ("error out"=w471:errorcluster, "S4ACS_GUI out"=w461:refnum<class "S4GUI.lvclass">)  [unwired: 7 in]
          n185 = Bundle By Name(cluster=w461, "Obs_state"=w457) -> (w460:refnum<class "S4GUI.lvclass">)
        }
        frame 251 {
          # "configura o canal,\nmas não dispara\na exposicao."
          # "Dispara o comando para o dispositivo corrente."
          n186 = flat-sequence {
            tunnel: [w508] -> w484
            tunnel: w485 -> [w508]
            frame #0 {
              n187 = Tick Count (ms)() -> (millisecond timer value=→"time3":u32)
            }
          }
          n188 = call-dynamic "Read Channel.vi"("error in (no error)"=w484, "Acquisition in"=w491) -> ("error out"=w496:errorcluster, "Channel.lvclass"=w498:refnum<class "Channel.lvclass">, "Acquisition out"=w506:refnum<class "Acquisition.lvclass">)  [unwired: 7 in]
          n189 = call-dynamic "Write expose.vi"("error in (no error)"=w496, "expose"=FALSE, "Channel in"=w498) -> ("error out"=w495:errorcluster, "Channel out"=w497:refnum<class "Channel.lvclass">)  [unwired: 7 in]
          n190 = call-dynamic "Read State Machine.vi"("error in (no error)"=w495, "Device in"=w497) -> ("error out"=w503:errorcluster, "State Machine.lvclass"=w505:refnum<class "State Machine.lvclass">, "Device out"=w501:refnum<class "Channel.lvclass">)  [unwired: 7 in]
          n191 = call "Next State.vi"("error in (no error)"=w503, "New_State"=1, "State Machine in"=w505) -> ("error out"=w492:errorcluster, "State Machine out"=w493:refnum<class "State Machine.lvclass">)  [unwired: 7 in]
          n192 = call-dynamic "Write State Machine.vi"("error in (no error)"=w492, "State Machine.lvclass"=w493, "Device in"=w501) -> ("error out"=w500:errorcluster, "Device out"=w502:refnum<class "Channel.lvclass">)  [unwired: 7 in]
          n193 = call-dynamic "Write Channel.vi"("error in (no error)"=w500, "Channel.lvclass"=w502, "Acquisition in"=w506) -> ("error out"=w487:errorcluster, "Acquisition out"=w489:refnum<class "Acquisition.lvclass">)  [unwired: 7 in]
          n194 = Increment(x=w499) -> (x+1=w490:u32)
          n195 = Bundle By Name(cluster=w483, "Error Msg"="", "cyclesDone"=u32 0) -> (w481:refnum<class "S4GUI.lvclass">)
          n196 = call-dynamic "Write Acq_state.vi"("error in (no error)"=w487, "Acq_state"=w490, "Acquisition in"=w489) -> ("error out"=w486:errorcluster, "Acquisition out"=w488:refnum<class "Acquisition.lvclass">)  [unwired: 7 in]
        }
        frame 252 {
          # "Erro no Texp."
          # "Erro no setup\ninicial do ACS."
          # "Espera terminar a execução do comando atual \nantes de ir ao proximo passo da Observação."
          n197 = flat-sequence {
            tunnel: [w553] -> w521
            tunnel: w522 -> [w553]
            frame #0 {
              n198 = Tick Count (ms)() -> (millisecond timer value=→"time4":u32)
            }
          }
          n199 = call-dynamic "Read Channel.vi"("error in (no error)"=w521, "Acquisition in"=w527) -> ("error out"=w536:errorcluster, "Channel.lvclass"=w535:refnum<class "Channel.lvclass">, "Acquisition out"=w537:refnum<class "Acquisition.lvclass">)  [unwired: 7 in]
          n200 = call-dynamic "Read State Machine.vi"("error in (no error)"=w536, "Device in"=w535) -> ("error out"=w529:errorcluster, "State Machine.lvclass"=w531:refnum<class "State Machine.lvclass">, "Device out"=w533:refnum<class "Channel.lvclass">)  [unwired: 7 in]
          n201 = call-dynamic "Read State.vi"("error in (no error)"=w529, "State Machine in"=w531) -> ("error out"=w528:errorcluster, "State"=w519:i32, "State Machine out"=w530:refnum<class "State Machine.lvclass">)  [unwired: 7 in]
          n202 = Equal To 0?(x=w519) -> (x = 0?=w517:bool)
          n203 = call-dynamic "Write State Machine.vi"("error in (no error)"=w528, "State Machine.lvclass"=w530, "Device in"=w533) -> ("error out"=w532:errorcluster, "Device out"=w534:refnum<class "Channel.lvclass">)  [unwired: 7 in]
          n204 = Equal?(x=28, y=w519) -> (x = y?=w516:bool)
          n205 = Equal?(x=38, y=w519) -> (x = y?=w515:bool)
          n206 = call-dynamic "Write Channel.vi"("error in (no error)"=w532, "Channel.lvclass"=w534, "Acquisition in"=w537) -> ("error out"=w526:errorcluster, "Acquisition out"=w525:refnum<class "Acquisition.lvclass">)  [unwired: 7 in]
          n207 = Build Array(w517, w516, w515) -> (w514:bool[])
          n208 = Boolean Array To Number(Boolean array=w514) -> (number=w513:u32)
          n209 = case shown="0, Default" w513 {
            tunnel: w512 -> [w539 _ _ _]
            tunnel: [w539 u32 300 ("t") u32 1 ("t") u32 1 ("t")] -> w511
            tunnel: w510 -> [w538 w542 w547 w551]
            tunnel: [w538 w541 w546 w550] -> w509
            frame 0, Default {
            }
            frame 1 {
              n210 = Tick Count (ms)() -> (millisecond timer value=→"time307":u32)
              n211 = Bundle By Name(cluster=w542, "Error Msg"="") -> (w541:refnum<class "S4GUI.lvclass">)
            }
            frame 2 {
              n212 = Bundle By Name(cluster=w547, "Error Msg"="ERROR: Some channel initialization failed. S4GUI:HandleObservationAsync.vi state 252.") -> (w546:refnum<class "S4GUI.lvclass">)
            }
            frame 4 {
              n213 = Bundle By Name(cluster=w551, "Error Msg"="ERROR: Some channel with invalid Exposition Time. S4GUI:HandleObservationAsync.vi state 252.") -> (w550:refnum<class "S4GUI.lvclass">)
            }
          }
          n214 = call-dynamic "Write Acq_state.vi"("error in (no error)"=w526, "Acq_state"=w511, "Acquisition in"=w525) -> ("error out"=w523:errorcluster, "Acquisition out"=w524:refnum<class "Acquisition.lvclass">)  [unwired: 7 in]
        }
        frame 253 {
          # "Sem syncbox, \ntrigger mode = 0 (internal)"
          n215 = call-dynamic "Read Channel.vi"("error in (no error)"=w556, "Acquisition in"=w588) -> ("error out"=w561:errorcluster, "Channel.lvclass"=w560:refnum<class "Channel.lvclass">, "Acquisition out"=w583:refnum<class "Acquisition.lvclass">)  [unwired: 7 in]
          n216 = call-dynamic "Read Interface.vi"("error in (no error)"=w561, "Channel in"=w560) -> ("error out"=w559:errorcluster, "Interface.lvclass"=w565:refnum<class "Interface.lvclass">, "Channel out"=w564:refnum<class "Channel.lvclass">)  [unwired: 7 in]
          n217 = call-dynamic "Get CCD_Config.vi"("error in (no error)"=w559, "Interface in"=w565) -> ("error out"=w572:errorcluster, "output cluster"=w574:T1, "Interface out"=w571:refnum<class "Interface.lvclass">)  [unwired: 7 in]
          n218 = Bundle By Name(cluster=w574, "TRIGGER_MODE"=u8 0) -> (w570:T1)
          n219 = call-dynamic "Set CCD_Config.vi"("error in (no error)"=w572, "input cluster"=w570, "Interface in"=w571) -> ("error out"=w568:errorcluster, "Interface out"=w566:refnum<class "Interface.lvclass">)  [unwired: 7 in]
          n220 = Flatten To String(anything=w570, error in (no error)=w568) -> (data string=w569:string, error out=w567:errorcluster)  [unwired: 2 in, 1 out]
          n221 = call "Write flatted cluster.vi"("error in (no error)"=w567, "flatted cluster"=w569, "Interface in"=w566) -> ("error out"=w562:errorcluster, "Interface out"=w563:refnum<class "Interface.lvclass">)  [unwired: 7 in]
          n222 = call-dynamic "Write Interface.vi"("error in (no error)"=w562, "Interface.lvclass"=w563, "Channel in"=w564) -> ("error out"=w558:errorcluster, "Channel out"=w557:refnum<class "Channel.lvclass">)  [unwired: 7 in]
          n223 = call-dynamic "Read State Machine.vi"("error in (no error)"=w558, "Device in"=w557) -> ("error out"=w580:errorcluster, "State Machine.lvclass"=w582:refnum<class "State Machine.lvclass">, "Device out"=w578:refnum<class "Channel.lvclass">)  [unwired: 7 in]
          n224 = Increment(x=w585) -> (x+1=w586:u32)
          n225 = call "Next State.vi"("error in (no error)"=w580, "New_State"=60, "State Machine in"=w582) -> ("error out"=w575:errorcluster, "State Machine out"=w576:refnum<class "State Machine.lvclass">)  [unwired: 7 in]
          n226 = call-dynamic "Write State Machine.vi"("error in (no error)"=w575, "State Machine.lvclass"=w576, "Device in"=w578) -> ("error out"=w577:errorcluster, "Device out"=w579:refnum<class "Channel.lvclass">)  [unwired: 7 in]
          n227 = call-dynamic "Write Channel.vi"("error in (no error)"=w577, "Channel.lvclass"=w579, "Acquisition in"=w583) -> ("error out"=w584:errorcluster, "Acquisition out"=w587:refnum<class "Acquisition.lvclass">)  [unwired: 7 in]
          n228 = call-dynamic "Write Acq_state.vi"("error in (no error)"=w584, "Acq_state"=w586, "Acquisition in"=w587) -> ("error out"=w589:errorcluster, "Acquisition out"=w590:refnum<class "Acquisition.lvclass">)  [unwired: 7 in]
        }
        frame 254 {
          # "Espera terminar a execução do comando atual \nantes de ir ao proximo passo da Observação."
          n229 = call-dynamic "Read Channel.vi"("error in (no error)"=w593, "Acquisition in"=w600) -> ("error out"=w611:errorcluster, "Channel.lvclass"=w610:refnum<class "Channel.lvclass">, "Acquisition out"=w612:refnum<class "Acquisition.lvclass">)  [unwired: 7 in]
          n230 = call-dynamic "Read State Machine.vi"("error in (no error)"=w611, "Device in"=w610) -> ("error out"=w604:errorcluster, "State Machine.lvclass"=w606:refnum<class "State Machine.lvclass">, "Device out"=w608:refnum<class "Channel.lvclass">)  [unwired: 7 in]
          n231 = call-dynamic "Read State.vi"("error in (no error)"=w604, "State Machine in"=w606) -> ("error out"=w603:errorcluster, "State"=w601:i32, "State Machine out"=w605:refnum<class "State Machine.lvclass">)  [unwired: 7 in]
          n232 = Equal To 0?(x=w601) -> (x = 0?=w602:bool)
          n233 = call-dynamic "Write State Machine.vi"("error in (no error)"=w603, "State Machine.lvclass"=w605, "Device in"=w608) -> ("error out"=w607:errorcluster, "Device out"=w609:refnum<class "Channel.lvclass">)  [unwired: 7 in]
          n234 = call-dynamic "Write Channel.vi"("error in (no error)"=w607, "Channel.lvclass"=w609, "Acquisition in"=w612) -> ("error out"=w597:errorcluster, "Acquisition out"=w596:refnum<class "Acquisition.lvclass">)  [unwired: 7 in]
          n235 = Select(t=u32 299, s=w602, f=w592) -> (s? t:f=w598:u32)
          n236 = call-dynamic "Write Acq_state.vi"("error in (no error)"=w597, "Acq_state"=w598, "Acquisition in"=w596) -> ("error out"=w594:errorcluster, "Acquisition out"=w595:refnum<class "Acquisition.lvclass">)  [unwired: 7 in]
        }
        frame 271 {
          # "configura o canal,\nmas não dispara\na exposicao."
          # "Dispara o comando para o dispositivo corrente."
          n237 = flat-sequence {
            tunnel: [w644] -> w621
            tunnel: w622 -> [w644]
            frame #0 {
              n238 = Tick Count (ms)() -> (millisecond timer value=→"time5":u32)
            }
          }
          n239 = call-dynamic "Read Channel.vi"("error in (no error)"=w621, "Acquisition in"=w627) -> ("error out"=w632:errorcluster, "Channel.lvclass"=w634:refnum<class "Channel.lvclass">, "Acquisition out"=w642:refnum<class "Acquisition.lvclass">)  [unwired: 7 in]
          n240 = call-dynamic "Write expose.vi"("error in (no error)"=w632, "expose"=FALSE, "Channel in"=w634) -> ("error out"=w631:errorcluster, "Channel out"=w633:refnum<class "Channel.lvclass">)  [unwired: 7 in]
          n241 = call-dynamic "Read State Machine.vi"("error in (no error)"=w631, "Device in"=w633) -> ("error out"=w639:errorcluster, "State Machine.lvclass"=w641:refnum<class "State Machine.lvclass">, "Device out"=w637:refnum<class "Channel.lvclass">)  [unwired: 7 in]
          n242 = call "Next State.vi"("error in (no error)"=w639, "New_State"=1, "State Machine in"=w641) -> ("error out"=w628:errorcluster, "State Machine out"=w629:refnum<class "State Machine.lvclass">)  [unwired: 7 in]
          n243 = call-dynamic "Write State Machine.vi"("error in (no error)"=w628, "State Machine.lvclass"=w629, "Device in"=w637) -> ("error out"=w636:errorcluster, "Device out"=w638:refnum<class "Channel.lvclass">)  [unwired: 7 in]
          n244 = call-dynamic "Write Channel.vi"("error in (no error)"=w636, "Channel.lvclass"=w638, "Acquisition in"=w642) -> ("error out"=w614:errorcluster, "Acquisition out"=w625:refnum<class "Acquisition.lvclass">)  [unwired: 7 in]
          n245 = Increment(x=w635) -> (x+1=w626:u32)
          n246 = Unbundle By Name(w616) -> ("TelFocus.lvclass"=w618:refnum<class "TelFocus.lvclass">)
          n247 = call-dynamic "Write focus #stepsdone.vi"("error in (no error)"=w614, "focus #stepsdone"=u32 0, "TelFocus in"=w618) -> ("error out"=w613:errorcluster, "TelFocus out"=w615:refnum<class "TelFocus.lvclass">)  [unwired: 7 in]
          n248 = Bundle By Name(cluster=w616, "TelFocus.lvclass"=w615, "Error Msg"="") -> (w619:refnum<class "S4GUI.lvclass">)
          n249 = call-dynamic "Write Acq_state.vi"("error in (no error)"=w613, "Acq_state"=w626, "Acquisition in"=w625) -> ("error out"=w623:errorcluster, "Acquisition out"=w624:refnum<class "Acquisition.lvclass">)  [unwired: 7 in]
        }
        frame 272 {
          # "Erro no Texp."
          # "Erro no setup\ninicial do ACS."
          # "Espera terminar a execução do comando atual \nantes de ir ao proximo passo da Observação."
          n250 = flat-sequence {
            tunnel: [w688] -> w657
            tunnel: w658 -> [w688]
            frame #0 {
              n251 = Tick Count (ms)() -> (millisecond timer value=→"time6":u32)
            }
          }
          n252 = call-dynamic "Read Channel.vi"("error in (no error)"=w657, "Acquisition in"=w663) -> ("error out"=w672:errorcluster, "Channel.lvclass"=w671:refnum<class "Channel.lvclass">, "Acquisition out"=w673:refnum<class "Acquisition.lvclass">)  [unwired: 7 in]
          n253 = call-dynamic "Read State Machine.vi"("error in (no error)"=w672, "Device in"=w671) -> ("error out"=w665:errorcluster, "State Machine.lvclass"=w667:refnum<class "State Machine.lvclass">, "Device out"=w669:refnum<class "Channel.lvclass">)  [unwired: 7 in]
          n254 = call-dynamic "Read State.vi"("error in (no error)"=w665, "State Machine in"=w667) -> ("error out"=w664:errorcluster, "State"=w655:i32, "State Machine out"=w666:refnum<class "State Machine.lvclass">)  [unwired: 7 in]
          n255 = Equal To 0?(x=w655) -> (x = 0?=w653:bool)
          n256 = call-dynamic "Write State Machine.vi"("error in (no error)"=w664, "State Machine.lvclass"=w666, "Device in"=w669) -> ("error out"=w668:errorcluster, "Device out"=w670:refnum<class "Channel.lvclass">)  [unwired: 7 in]
          n257 = Equal?(x=28, y=w655) -> (x = y?=w652:bool)
          n258 = Equal?(x=38, y=w655) -> (x = y?=w651:bool)
          n259 = call-dynamic "Write Channel.vi"("error in (no error)"=w668, "Channel.lvclass"=w670, "Acquisition in"=w673) -> ("error out"=w662:errorcluster, "Acquisition out"=w661:refnum<class "Acquisition.lvclass">)  [unwired: 7 in]
          n260 = Build Array(w653, w652, w651) -> (w650:bool[])
          n261 = Boolean Array To Number(Boolean array=w650) -> (number=w649:u32)
          n262 = case shown="1" w649 {
            tunnel: w648 -> [w674 _ _ _]
            tunnel: [w674 u32 360 ("t") u32 0 ("t") u32 0 ("t")] -> w647
            tunnel: w646 -> [w675 w677 w682 w686]
            tunnel: [w675 w676 w681 w685] -> w645
            frame 0, Default {
            }
            frame 1 {
              n263 = Bundle By Name(cluster=w677, "Error Msg"="") -> (w676:refnum<class "S4GUI.lvclass">)
            }
            frame 2 {
              n264 = Bundle By Name(cluster=w682, "Error Msg"="ERROR: Some channel initialization failed. S4GUI:HandleObservationAsync.vi state 272.") -> (w681:refnum<class "S4GUI.lvclass">)
            }
            frame 4 {
              n265 = Bundle By Name(cluster=w686, "Error Msg"="ERROR: Some channel with invalid Exposition Time. S4GUI:HandleObservationAsync.vi state 272.") -> (w685:refnum<class "S4GUI.lvclass">)
            }
          }
          n266 = call-dynamic "Write Acq_state.vi"("error in (no error)"=w662, "Acq_state"=w647, "Acquisition in"=w661) -> ("error out"=w659:errorcluster, "Acquisition out"=w660:refnum<class "Acquisition.lvclass">)  [unwired: 7 in]
        }
        frame 300 {
          # "Verifica se é modo fotometria ou polarimetria:\nTrue = polarimetria (estado 301)\nFalse = fotometria (estado 321)"
          n267 = flat-sequence {
            tunnel: [w716] -> w705
            tunnel: w706 -> [w716]
            frame #0 {
              n268 = local read "time4"() -> (w718:u32)
              n269 = local read "time3"() -> (w717:u32)
              n270 = Subtract(x=w718, y=w717) -> (x-y=→"delay 3-4":u32)
            }
          }
          n271 = call "Read Instrument.lvclass.vi"("error in (no error)"=w705, "S4ACS_GUI in"=w715) -> ("error out"=w712:errorcluster, "Instrument.lvclass"=w713:refnum<class "Instrument.lvclass">, "S4ACS_GUI out"=w702:refnum<class "S4GUI.lvclass">)  [unwired: 7 in]
          n272 = call-dynamic "Read mode.vi"("error in (no error)"=w712, "Instrument in"=w713) -> ("error out"=w692:errorcluster, "mode"=w711:bool)  [unwired: 7 in, 1 out]
          n273 = call-dynamic "Read Channel.vi"("error in (no error)"=w692, "Acquisition in"=w700) -> ("error out"=w694:errorcluster, "Channel.lvclass"=w696:refnum<class "Channel.lvclass">, "Acquisition out"=w699:refnum<class "Acquisition.lvclass">)  [unwired: 7 in]
          n274 = call-dynamic "Write PrevCyclesDone.vi"("error in (no error)"=w694, "PrevCyclesDone"=u32 0, "Channel in"=w696) -> ("error out"=w693:errorcluster, "Channel out"=w695:refnum<class "Channel.lvclass">)  [unwired: 7 in]
          n275 = call-dynamic "Write Channel.vi"("error in (no error)"=w693, "Channel.lvclass"=w695, "Acquisition in"=w699) -> ("error out"=w691:errorcluster, "Acquisition out"=w698:refnum<class "Acquisition.lvclass">)  [unwired: 7 in]
          n276 = Select(t=u32 301, s=w711, f=u32 321 ("t")) -> (s? t:f=w709:u32)
          n277 = call-dynamic "Write Acq_state.vi"("error in (no error)"=w691, "Acq_state"=w709, "Acquisition in"=w698) -> ("error out"=w708:errorcluster, "Acquisition out"=w707:refnum<class "Acquisition.lvclass">)  [unwired: 7 in]
          n278 = Bundle By Name(cluster=w702, "cyclesDone"=u32 0, "sequesDone"=u32 0, "seqAtual"=u32 0) -> (w701:refnum<class "S4GUI.lvclass">)
        }
        frame 301 {
          # "Se for polarimetria com 1 pos,\ndesabilita WAIT EXPOSE no ACS."
          # "Envia WAIT_EXPOSE_COMMAND ...\nON (se forem varias posicoes) ou\nOFF (se for uma única posição da lâmina.)"
          n279 = call-dynamic "VerifWavePlate.vi"("error in (no error)"=w724, "S4GUI in"=w725) -> ("error out"=w723:errorcluster, "One Position"=w721:bool, "S4GUI out"=w722:refnum<class "S4GUI.lvclass">)  [unwired: 7 in]
          n280 = Not(x=w721) -> (.not. x?=w720:bool)
          n281 = call-dynamic "Read Channel.vi"("error in (no error)"=w723, "Acquisition in"=w739) -> ("error out"=w727:errorcluster, "Channel.lvclass"=w729:refnum<class "Channel.lvclass">, "Acquisition out"=w747:refnum<class "Acquisition.lvclass">)  [unwired: 7 in]
          n282 = call-dynamic "Write wait_expose.vi"("error in (no error)"=w727, "wait_expose"=w720, "Channel in"=w729) -> ("error out"=w726:errorcluster, "Channel out"=w728:refnum<class "Channel.lvclass">)  [unwired: 7 in]
          n283 = call-dynamic "Read State Machine.vi"("error in (no error)"=w726, "Device in"=w728) -> ("error out"=w744:errorcluster, "State Machine.lvclass"=w746:refnum<class "State Machine.lvclass">, "Device out"=w742:refnum<class "Channel.lvclass">)  [unwired: 7 in]
          n284 = call "Next State.vi"("error in (no error)"=w744, "New_State"=40, "State Machine in"=w746) -> ("error out"=w732:errorcluster, "State Machine out"=w733:refnum<class "State Machine.lvclass">)  [unwired: 7 in]
          n285 = call-dynamic "Write State Machine.vi"("error in (no error)"=w732, "State Machine.lvclass"=w733, "Device in"=w742) -> ("error out"=w741:errorcluster, "Device out"=w743:refnum<class "Channel.lvclass">)  [unwired: 7 in]
          n286 = Increment(x=w740) -> (x+1=w738:u32)
          n287 = call-dynamic "Write Channel.vi"("error in (no error)"=w741, "Channel.lvclass"=w743, "Acquisition in"=w747) -> ("error out"=w737:errorcluster, "Acquisition out"=w736:refnum<class "Acquisition.lvclass">)  [unwired: 7 in]
          n288 = call-dynamic "Write Acq_state.vi"("error in (no error)"=w737, "Acq_state"=w738, "Acquisition in"=w736) -> ("error out"=w734:errorcluster, "Acquisition out"=w735:refnum<class "Acquisition.lvclass">)  [unwired: 7 in]
          n289 = Bundle By Name(cluster=w722, "Error Msg"="") -> (w730:refnum<class "S4GUI.lvclass">)
        }
        frame 302 {
          # "Espera canal voltar para IDLE"
          n290 = call-dynamic "Read Channel.vi"("error in (no error)"=w763, "Acquisition in"=w764) -> ("error out"=w754:errorcluster, "Channel.lvclass"=w755:refnum<class "Channel.lvclass">, "Acquisition out"=w756:refnum<class "Acquisition.lvclass">)  [unwired: 7 in]
          n291 = call-dynamic "Read State Machine.vi"("error in (no error)"=w754, "Device in"=w755) -> ("error out"=w757:errorcluster, "State Machine.lvclass"=w759:refnum<class "State Machine.lvclass">)  [unwired: 7 in, 1 out]
          n292 = call-dynamic "Read State.vi"("error in (no error)"=w757, "State Machine in"=w759) -> ("error out"=w752:errorcluster, "State"=w758:i32)  [unwired: 7 in, 1 out]
          n293 = Equal?(x=0, y=w758) -> (x = y?=w748:bool)
          n294 = Increment(x=w750) -> (x+1=w751:u32)
          n295 = Select(t=w751, s=w748, f=w750) -> (s? t:f=w753:u32)
          n296 = call-dynamic "Write Acq_state.vi"("error in (no error)"=w752, "Acq_state"=w753, "Acquisition in"=w756) -> ("error out"=w761:errorcluster, "Acquisition out"=w762:refnum<class "Acquisition.lvclass">)  [unwired: 7 in]
        }
        frame 303 {
          # "2024 04 26: ATEN敲O: NO MODO POLARIMETRIA ASYNC, APENAS 1 CANAL POR VEZ PODE FAZER AQUISI敲O!\nO atributo S4GUI:SeqAtual pode se perder se mais de um canal rodar aqui..."
          n297 = flat-sequence {
            tunnel: w770 -> [w811]
            tunnel: [w811] -> w769
            frame #0 {
              n298 = Tick Count (ms)() -> (millisecond timer value=→"time1":u32)
            }
          }
          n299 = call "Read Instrument.lvclass.vi"("error in (no error)"=w769, "S4ACS_GUI in"=w807) -> ("error out"=w809:errorcluster, "Instrument.lvclass"=w810:refnum<class "Instrument.lvclass">, "S4ACS_GUI out"=w767:refnum<class "S4GUI.lvclass">)  [unwired: 7 in]
          n300 = call "Read WPROT.vi"("error in (no error)"=w809, "Instrument in"=w810) -> ("error out"=w804:errorcluster, "Opt_Selector.lvclass"=w805:refnum<class "Opt_Selector.lvclass">, "Instrument out"=w808:refnum<class "Instrument.lvclass">)  [unwired: 7 in]
          n301 = call-dynamic "getTargetPos.vi"("error in (no error)"=w804, "Opt_Selector in"=w805) -> ("error out"=w803:errorcluster, "Target Pos"=w783:u16, "Opt_Selector out"=w802:refnum<class "Opt_Selector.lvclass">)  [unwired: 7 in]
          n302 = Build Array(-1.0 ("element"), 0.0 ("element"), 22.5 ("element"), 45.0 ("element"), 67.5 ("element"), 90.0 ("element"), 112.5 ("element"), 135.0 ("element"), 157.5 ("element"), 180.0 ("element"), 202.5 ("element"), 225.0 ("element"), 247.5 ("element"), 270.0 ("element"), 292.5 ("element"), 315.0 ("element"), 337.5 ("element")) -> (w795:dbl[])
          n303 = Unbundle By Name(w767) -> ("seqAtual"=w768:u32)
          n304 = Index Array(array=w795, index=w783) -> (element=w782:dbl)
          n305 = case shown="1..16" w783 {
            selector: w783 -> [_ w845]
            tunnel: w808 -> [w821 w833]
            tunnel: [w821 w833] -> w778
            tunnel: [w818 w832] -> w777
            tunnel: w806 -> [_ w847]
            tunnel: [u32 314 w846] -> w776
            tunnel: w803 -> [w819 w841]
            tunnel: w802 -> [w820 w840]
            tunnel: w782 -> [_ w835]
            tunnel: [w816 w834] -> w779
            tunnel: [u32 0 ("seqAtual") w823] -> w766
            tunnel: w768 -> [_ w824]
            frame 0, Default {
              # "Verifica os ciclos"
              # "Recupera a sequencia anterior para o caso \nde repetição da sequencia (sem precisar clicar \nnas posicoes desejadas novamente)."
              n306 = call-dynamic "Read sequencia_ant.vi"("error in (no error)"=w819, "Opt_Selector in"=w820) -> ("error out"=w815:errorcluster, "sequencia_ant"=w814:u16, "Opt_Selector out"=w817:refnum<class "Opt_Selector.lvclass">)  [unwired: 7 in]
              n307 = call-dynamic "Write sequencia.vi"("error in (no error)"=w815, "sequencia"=w814, "Opt_Selector in"=w817) -> ("error out"=w818:errorcluster, "Opt_Selector out"=w816:refnum<class "Opt_Selector.lvclass">)  [unwired: 7 in]
            }
            frame 1..16 {
              # "Inicia o Ticks com\nvalor do relogio atual"
              # "Espera até 40 x 0.25s (= 10s) para\nmecanismo entrar em READY"
              n308 = Number To Decimal String(number=w845) -> (decimal integer string=w844:string)  [unwired: 1 in]
              n309 = Concatenate Strings("WP" ("string"), w844) -> (w842:string)
              n310 = call "Write target name.vi"("error in (no error)"=w841, "target name"=w842, "Optics in"=w840) -> ("error out"=w838:errorcluster, "Optics out"=w839:refnum<class "Opt_Selector.lvclass">)  [unwired: 7 in]
              n311 = call "Write target.vi"("error in (no error)"=w838, "target"=w835, "Optics in"=w839) -> ("error out"=w837:errorcluster, "Optics out"=w836:refnum<class "Opt_Selector.lvclass">)  [unwired: 7 in]
              n312 = call-dynamic "Read State Machine.vi"("error in (no error)"=w837, "Device in"=w836) -> ("error out"=w849:errorcluster, "State Machine.lvclass"=w851:refnum<class "State Machine.lvclass">, "Device out"=w848:refnum<class "Opt_Selector.lvclass">)  [unwired: 7 in]
              n313 = Increment(x=w847) -> (x+1=w846:u32)
              n314 = Increment(x=w824) -> (x+1=w823:u32)
              n315 = call "Next State.vi"("error in (no error)"=w849, "New_State"=1, "State Machine in"=w851) -> ("error out"=w830:errorcluster, "State Machine out"=w831:refnum<class "State Machine.lvclass">)  [unwired: 7 in]
              n316 = call-dynamic "Write Timer.vi"("error in (no error)"=w830, "Timer"=u32 40, "State Machine in"=w831) -> ("error out"=w827:errorcluster, "State Machine out"=w828:refnum<class "State Machine.lvclass">)  [unwired: 7 in]
              n317 = call-dynamic "Init Ticks.vi"("error in (no error)"=w827, "State Machine in"=w828) -> ("error out"=w825:errorcluster, "State Machine out"=w826:refnum<class "State Machine.lvclass">)  [unwired: 8 in]
              n318 = call-dynamic "Write State Machine.vi"("error in (no error)"=w825, "State Machine.lvclass"=w826, "Device in"=w848) -> ("error out"=w832:errorcluster, "Device out"=w834:refnum<class "Opt_Selector.lvclass">)  [unwired: 7 in]
            }
          }
          n319 = call "Write WPROT.vi"("error in (no error)"=w777, "Opt_Selector.lvclass"=w779, "Instrument in"=w778) -> ("error out"=w781:errorcluster, "Instrument out"=w780:refnum<class "Instrument.lvclass">)  [unwired: 7 in]
          n320 = Bundle By Name(cluster=w767, "seqAtual"=w766) -> (w765:refnum<class "S4GUI.lvclass">)
          n321 = call "Write Instrument.lvclass.vi"("error in (no error)"=w781, "Instrument.lvclass"=w780, "S4ACS_GUI in"=w765) -> ("error out"=w774:errorcluster, "S4ACS_GUI out"=w773:refnum<class "S4GUI.lvclass">)  [unwired: 7 in]
          n322 = call-dynamic "Write Acq_state.vi"("error in (no error)"=w774, "Acq_state"=w776, "Acquisition in"=w775) -> ("error out"=w772:errorcluster, "Acquisition out"=w771:refnum<class "Acquisition.lvclass">)  [unwired: 7 in]
        }
        frame 304 {
          # "Espera terminar o movimento para a posição \"target\" do waveplate\nantes de ir para o estado que dispara a aquisição de imagens.\n\n20230424: Não precisa mais atualizar o valor de WPPOS com o\ncomando WRITE_HEADER porque o ACS já recebeu a sequência de\nposições da lâmina"
          n323 = flat-sequence {
            tunnel: [w908] -> w876
            tunnel: w877 -> [w908]
            frame #0 {
              n324 = Tick Count (ms)() -> (millisecond timer value=→"time 2":u32)
            }
          }
          n325 = call "Read Instrument.lvclass.vi"("error in (no error)"=w876, "S4ACS_GUI in"=w890) -> ("error out"=w895:errorcluster, "Instrument.lvclass"=w896:refnum<class "Instrument.lvclass">, "S4ACS_GUI out"=w892:refnum<class "S4GUI.lvclass">)  [unwired: 7 in]
          n326 = call "Read WPROT.vi"("error in (no error)"=w895, "Instrument in"=w896) -> ("error out"=w857:errorcluster, "Opt_Selector.lvclass"=w889:refnum<class "Opt_Selector.lvclass">, "Instrument out"=w894:refnum<class "Instrument.lvclass">)  [unwired: 7 in]
          n327 = call-dynamic "Read Channel.vi"("error in (no error)"=w857, "Acquisition in"=w859) -> ("error out"=w853:errorcluster, "Channel.lvclass"=w854:refnum<class "Channel.lvclass">, "Acquisition out"=w858:refnum<class "Acquisition.lvclass">)  [unwired: 7 in]
          n328 = call-dynamic "Read wait_expose.vi"("error in (no error)"=w853, "Channel in"=w854) -> ("error out"=w856:errorcluster, "wait_expose"=w855:bool)  [unwired: 7 in, 1 out]
          n329 = call-dynamic "Read State Machine.vi"("error in (no error)"=w856, "Device in"=w889) -> ("error out"=w863:errorcluster, "State Machine.lvclass"=w866:refnum<class "State Machine.lvclass">, "Device out"=w887:refnum<class "Opt_Selector.lvclass">)  [unwired: 7 in]
          n330 = call-dynamic "Verif Clock.vi"("error in (no error)"=w863, "period (ms)"=u32 20000 ("period"), "State Machine in"=w866) -> ("error out"=w867:errorcluster, "State Machine out"=w865:refnum<class "State Machine.lvclass">)  [unwired: 6 in, 1 out]
          n331 = call-dynamic "Read Timeout.vi"("error in (no error)"=w867, "State Machine in"=w865) -> ("error out"=w862:errorcluster, "Timeout"=w861:bool, "State Machine out"=w864:refnum<class "State Machine.lvclass">)  [unwired: 7 in]
          n332 = call-dynamic "Read State.vi"("error in (no error)"=w862, "State Machine in"=w864) -> ("error out"=w878:errorcluster, "State"=w884:i32, "State Machine out"=w879:refnum<class "State Machine.lvclass">)  [unwired: 7 in]
          n333 = call-dynamic "Write State Machine.vi"("error in (no error)"=w878, "State Machine.lvclass"=w879, "Device in"=w887) -> ("error out"=w886:errorcluster, "Device out"=w888:refnum<class "Opt_Selector.lvclass">)  [unwired: 7 in]
          n334 = Equal To 0?(x=w884) -> (x = 0?=w885:bool)
          n335 = call "Write WPROT.vi"("error in (no error)"=w886, "Opt_Selector.lvclass"=w888, "Instrument in"=w894) -> ("error out"=w891:errorcluster, "Instrument out"=w893:refnum<class "Instrument.lvclass">)  [unwired: 7 in]
          n336 = call "Write Instrument.lvclass.vi"("error in (no error)"=w891, "Instrument.lvclass"=w893, "S4ACS_GUI in"=w892) -> ("error out"=w882:errorcluster, "S4ACS_GUI out"=w869:refnum<class "S4GUI.lvclass">)  [unwired: 7 in]
          n337 = case shown="True" w861 {
            tunnel: w871 -> [w898 _]
            tunnel: [w898 u32 1 ("Obs_state")] -> w870
            tunnel: w869 -> [w897 w902]
            tunnel: [w897 w901] -> w860
            frame False {
            }
            frame True {
              n338 = Bundle By Name(cluster=w902, "Error Msg"="ERROR: moving waveplate (S4GUI:HandleObservationAsync.vi - state 304)") -> (w901:refnum<class "S4GUI.lvclass">)
            }
          }
          n339 = Unbundle By Name(w869) -> ("cyclesDone"=w874:u32, "sequesDone"=w873:u32)
          n340 = Add(x=w874, y=w873) -> (x+y=w875:u32)
          n341 = Equal To 0?(x=w875) -> ()  [unwired: 1 out]
          n342 = case shown="True" TRUE {
            tunnel: [w903 u32 308 ("t")] -> w872
            tunnel: w855 -> [w905 _]
            frame False {
              # "2a seq. em diante: depende\nde Channel.wait_expose"
              n343 = Select(t=u32 308, s=w905, f=u32 326 ("t")) -> (s? t:f=w903:u32)
            }
            frame True {
              # "1a. seq.: Envia EXPOSE"
            }
          }
          n344 = Select(t=w872, s=w885, f=w870) -> (s? t:f=w883:u32)
          n345 = call-dynamic "Write Acq_state.vi"("error in (no error)"=w882, "Acq_state"=w883, "Acquisition in"=w858) -> ("error out"=w881:errorcluster, "Acquisition out"=w880:refnum<class "Acquisition.lvclass">)  [unwired: 7 in]
        }
        frame 308 {
          # "Dispara o comando para o dispositivo corrente."
          n346 = call-dynamic "Read Channel.vi"("error in (no error)"=w920, "Acquisition in"=w921) -> ("error out"=w927:errorcluster, "Channel.lvclass"=w926:refnum<class "Channel.lvclass">, "Acquisition out"=w931:refnum<class "Acquisition.lvclass">)  [unwired: 7 in]
          n347 = call-dynamic "Read State Machine.vi"("error in (no error)"=w927, "Device in"=w926) -> ("error out"=w928:errorcluster, "State Machine.lvclass"=w930:refnum<class "State Machine.lvclass">, "Device out"=w924:refnum<class "Channel.lvclass">)  [unwired: 7 in]
          n348 = call "Next State.vi"("error in (no error)"=w928, "New_State"=50, "State Machine in"=w930) -> ("error out"=w913:errorcluster, "State Machine out"=w914:refnum<class "State Machine.lvclass">)  [unwired: 7 in]
          n349 = call-dynamic "Write State Machine.vi"("error in (no error)"=w913, "State Machine.lvclass"=w914, "Device in"=w924) -> ("error out"=w923:errorcluster, "Device out"=w925:refnum<class "Channel.lvclass">)  [unwired: 7 in]
          n350 = Increment(x=w922) -> (x+1=w919:u32)
          n351 = call-dynamic "Write Channel.vi"("error in (no error)"=w923, "Channel.lvclass"=w925, "Acquisition in"=w931) -> ("error out"=w918:errorcluster, "Acquisition out"=w917:refnum<class "Acquisition.lvclass">)  [unwired: 7 in]
          n352 = call-dynamic "Write Acq_state.vi"("error in (no error)"=w918, "Acq_state"=w919, "Acquisition in"=w917) -> ("error out"=w915:errorcluster, "Acquisition out"=w916:refnum<class "Acquisition.lvclass">)  [unwired: 7 in]
          n353 = Bundle By Name(cluster=w912, "Error Msg"="") -> (w910:refnum<class "S4GUI.lvclass">)
        }
        frame 309 {
          # "Se wait_expose=T, não envia\no EXPOSE do estado 308\n(1o EXPOSE já foi enviado).\n\nNeste caso, vai para:\n* 312 se houver mais \n   de 1 posição da lamina ou para \n* 326 se houver apenas 1 posição\n   da lâmina"
          # "OV 20240821 -Espera ACTIVE ou SeqsDone incrementar."
          n354 = Unbundle By Name(w939) -> ("seqAtual"=w938:u32)
          n355 = flat-sequence {
            tunnel: [w974] -> w933
            tunnel: w934 -> [w974]
            frame #0 {
              n356 = Tick Count (ms)() -> (millisecond timer value=→"time308":u32)
            }
          }
          n357 = call-dynamic "Read Channel.vi"("error in (no error)"=w933, "Acquisition in"=w961) -> ("error out"=w941:errorcluster, "Channel.lvclass"=w944:refnum<class "Channel.lvclass">, "Acquisition out"=w969:refnum<class "Acquisition.lvclass">)  [unwired: 7 in]
          n358 = call-dynamic "Read SequesDone.vi"("error in (no error)"=w941, "Channel in"=w944) -> ("error out"=w940:errorcluster, "SequesDoneRaw"=w942:u32, "Channel out"=w943:refnum<class "Channel.lvclass">)  [unwired: 6 in, 1 out]
          n359 = Equal?(x=w942, y=w938) -> (x = y?=w935:bool)
          n360 = call-dynamic "Read wait_expose.vi"("error in (no error)"=w940, "Channel in"=w943) -> ("error out"=w952:errorcluster, "Channel out"=w953:refnum<class "Channel.lvclass">)  [unwired: 7 in, 1 out]
          n361 = call-dynamic "Read State Machine.vi"("error in (no error)"=w952, "Device in"=w953) -> ("error out"=w963:errorcluster, "State Machine.lvclass"=w965:refnum<class "State Machine.lvclass">, "Device out"=w967:refnum<class "Channel.lvclass">)  [unwired: 7 in]
          n362 = call-dynamic "Read State.vi"("error in (no error)"=w963, "State Machine in"=w965) -> ("error out"=w962:errorcluster, "State"=w955:i32, "State Machine out"=w964:refnum<class "State Machine.lvclass">)  [unwired: 7 in]
          n363 = call-dynamic "Write State Machine.vi"("error in (no error)"=w962, "State Machine.lvclass"=w964, "Device in"=w967) -> ("error out"=w966:errorcluster, "Device out"=w968:refnum<class "Channel.lvclass">)  [unwired: 7 in]
          n364 = Greater?(x=w955, y=53) -> (0:w937:bool)
          n365 = disable-structure shown="Enabled" {
            disable-tunnel: w937 -> [w972 w973]
            disable-tunnel: [w971 w973] -> w936
            disable-tunnel: w935 -> [w970 _]
            frame Disabled {
              n366 = Or(x=w972, y=w970) -> (x .or. y?=w971:bool)
            }
            frame Enabled {
            }
          }
          n367 = call-dynamic "Write Channel.vi"("error in (no error)"=w966, "Channel.lvclass"=w968, "Acquisition in"=w969) -> ("error out"=w951:errorcluster, "Acquisition out"=w960:refnum<class "Acquisition.lvclass">)  [unwired: 7 in]
          n368 = call-dynamic "VerifWavePlate.vi"("error in (no error)"=w951, "S4GUI in"=w939) -> ("error out"=w950:errorcluster, "One Position"=w949:bool, "S4GUI out"=w945:refnum<class "S4GUI.lvclass">)  [unwired: 7 in]
          n369 = Select(t=u32 326, s=w949, f=u32 312 ("t")) -> (s? t:f=w932:u32)
          n370 = Select(t=w932, s=w936, f=w954) -> (s? t:f=w959:u32)
          n371 = call-dynamic "Write Acq_state.vi"("error in (no error)"=w950, "Acq_state"=w959, "Acquisition in"=w960) -> ("error out"=w957:errorcluster, "Acquisition out"=w958:refnum<class "Acquisition.lvclass">)  [unwired: 7 in]
          n372 = flat-sequence {
            tunnel: [w976] -> w946
            tunnel: w945 -> [w976]
            frame #0 {
              n373 = Tick Count (ms)() -> (millisecond timer value=w977:u32)
              n374 = local write "time307"(w977) -> ()
            }
          }
        }
        frame 312 {
          # "Exemplo:\nSET #CYCLES 3\nSET #SEQ 4\ntotal de sequencias: 3 x 4 = 12\n\nseq.        CYCLES_DONE           SEQS_DONE\n1a.                     0                                 0\n2a.                     0                                 1 \n3a.                     0                                 2 \n4a.                     0                                 3 \n\n5a.                     1                                 4->0 \n6a.                     1                                 1 \n7a.                     1                                 2 \n8a.                     1                                 3 \n\n9a.                     2                                 4->0 \n10a.                   2                                 1 \n11a.                   2                                 2 \n12a.                   2                                 3 \n\nfim                    3                                 4"
          # "SEQS_DONE = 0,1,2,...,n,0,1,..."
          n375 = Unbundle By Name(w995) -> ("seqAtual"=w996:u32)
          n376 = call-dynamic "Read Channel.vi"("error in (no error)"=w1001, "Acquisition in"=w1002) -> ("error out"=w988:errorcluster, "Channel.lvclass"=w990:refnum<class "Channel.lvclass">, "Acquisition out"=w1003:refnum<class "Acquisition.lvclass">)  [unwired: 7 in]
          n377 = call-dynamic "Read stopping.vi"("error in (no error)"=w988, "Channel in"=w990) -> ("error out"=w987:errorcluster, "stopping"=w986:bool, "Channel out"=w989:refnum<class "Channel.lvclass">)  [unwired: 7 in]
          n378 = call-dynamic "Read SequesDone.vi"("error in (no error)"=w987, "Channel in"=w989) -> ("error out"=w997:errorcluster, "SequesDoneRaw"=w978:u32, "Channel out"=w998:refnum<class "Channel.lvclass">)  [unwired: 6 in, 1 out]
          n379 = Equal?(x=w978, y=w996) -> (x = y?=w991:bool)
          n380 = call-dynamic "Write Channel.vi"("error in (no error)"=w997, "Channel.lvclass"=w998, "Acquisition in"=w1003) -> ("error out"=w984:errorcluster, "Acquisition out"=w985:refnum<class "Acquisition.lvclass">)  [unwired: 7 in]
          n381 = call-dynamic "GetCubeDuration.vi"("error in (no error)"=w984, "Acquisition in"=w985) -> ("error out"=w983:errorcluster, "Acquisition out"=w982:refnum<class "Acquisition.lvclass">, "CubeDuration"=w981:dbl)  [unwired: 7 in]
          n382 = Multiply(x=w981, y=1000.0) -> (x*y=w980:dbl)
          n383 = case shown="False" w991 {
            tunnel: w995 -> [w1005 w1022]
            tunnel: [w1004 w1022] -> w994
            tunnel: [w1006 w1024] -> w993
            tunnel: w992 -> [w1007 _]
            tunnel: w986 -> [_ w1023]
            tunnel: w980 -> [w1013 _]
            frame False {
              n384 = Add(x=1000.0, y=w1013) -> (x+y=w1011:dbl)
              n385 = local read "time307"() -> (w1014:u32)
              n386 = Tick Count (ms)() -> (millisecond timer value=w1015:u32)
              n387 = Subtract(x=w1015, y=w1014) -> (x-y=w1010:u32)
              n388 = To Double Precision Float(number=w1010) -> (double precision float=w1009:dbl)
              n389 = Less?(x=w1011, y=w1009) -> (x < y?=w1008:bool)
              n390 = case shown="True" w1008 {
                tunnel: w1007 -> [w1017 _]
                tunnel: [w1017 u32 1 ("Acq_state")] -> w1006
                tunnel: [w1016 w1019] -> w1004
                tunnel: w1005 -> [w1016 w1020]
                frame False {
                }
                frame True {
                  n391 = Bundle By Name(cluster=w1020, "Error Msg"="ERROR: Acquisition Timeout - HandleObservationAsync.vi - state 312.") -> (w1019:refnum<class "S4GUI.lvclass">)
                }
              }
            }
            frame True {
              n392 = case shown="False" w1023 {
                tunnel: [u32 303 ("Obs_state") u32 0 ("Obs_state")] -> w1024
                frame False {
                }
                frame True {
                }
              }
            }
          }
          n393 = call-dynamic "Write Acq_state.vi"("error in (no error)"=w983, "Acq_state"=w993, "Acquisition in"=w982) -> ("error out"=w999:errorcluster, "Acquisition out"=w1000:refnum<class "Acquisition.lvclass">)  [unwired: 7 in]
        }
        frame 314 {
          n394 = disable-structure shown="Enabled" {
            disable-tunnel: w1032 -> [w1049 w1065]
            disable-tunnel: w1031 -> [w1048 w1066]
            disable-tunnel: [w1037 w1064] -> w1030
            disable-tunnel: [w1036 w1063] -> w1029
            disable-tunnel: w1028 -> [w1033 w1060]
            disable-tunnel: [w1033 w1059] -> w1027
            frame Disabled {
              n395 = call-dynamic "Read Channel.vi"("error in (no error)"=w1049, "Acquisition in"=w1048) -> ("error out"=w1047:errorcluster, "Channel.lvclass"=w1046:refnum<class "Channel.lvclass">, "Acquisition out"=w1034:refnum<class "Acquisition.lvclass">)  [unwired: 7 in]
              n396 = call-dynamic "Read ciclos.vi"("error in (no error)"=w1047, "Channel in"=w1046) -> ("error out"=w1043:errorcluster, "ciclos"=w1045:u32, "Channel out"=w1035:refnum<class "Channel.lvclass">)  [unwired: 7 in]
              n397 = Decrement(x=w1045) -> (x-1=w1050:u32)
              n398 = Greater Than 0?(x=w1050) -> (x > 0?=w1054:bool)
              n399 = case shown="True" w1054 {
                selector: w1054 -> [w1056 w1058]
                tunnel: w1050 -> [_ w1057]
                tunnel: [w1056 w1058] -> w1053
                tunnel: [u32 0 w1057] -> w1040
                frame False {
                }
                frame True {
                }
              }
              n400 = call-dynamic "Write ciclos.vi"("error in (no error)"=w1043, "ciclos"=w1040, "Channel in"=w1035) -> ("error out"=w1042:errorcluster, "Channel out"=w1041:refnum<class "Channel.lvclass">)  [unwired: 7 in]
              n401 = Select(t=u32 301, s=w1053, f=u32 0) -> (s? t:f=w1044:u32)
              n402 = call-dynamic "Write Channel.vi"("error in (no error)"=w1042, "Channel.lvclass"=w1041, "Acquisition in"=w1034) -> ("error out"=w1038:errorcluster, "Acquisition out"=w1039:refnum<class "Acquisition.lvclass">)  [unwired: 7 in]
              n403 = call-dynamic "Write Acq_state.vi"("error in (no error)"=w1038, "Acq_state"=w1044, "Acquisition in"=w1039) -> ("error out"=w1036:errorcluster, "Acquisition out"=w1037:refnum<class "Acquisition.lvclass">)  [unwired: 7 in]
            }
            frame Enabled {
              n404 = Unbundle By Name(w1060) -> ("cyclesDone"=w1062:u32)
              n405 = Increment(x=w1062) -> (x+1=w1061:u32)
              n406 = Bundle By Name(cluster=w1060, "cyclesDone"=w1061) -> (w1059:refnum<class "S4GUI.lvclass">)
              n407 = Unbundle By Name(w1059) -> ("TotalCiclos"=w1073:u32, "cyclesDone"=w1072:u32)
              n408 = Subtract(x=w1073, y=w1072) -> (x-y=w1071:u32)
              n409 = Greater Than 0?(x=w1071) -> (x > 0?=w1070:bool)
              n410 = Select(t=u32 303, s=w1070, f=u32 0) -> (s? t:f=w1067:u32)
              n411 = call-dynamic "Write Acq_state.vi"("error in (no error)"=w1065, "Acq_state"=w1067, "Acquisition in"=w1066) -> ("error out"=w1063:errorcluster, "Acquisition out"=w1064:refnum<class "Acquisition.lvclass">)  [unwired: 7 in]
            }
          }
        }
        frame 321 {
          # "Envia: WAIT_EXPOSE_COMMAND  OFF"
          # "Para Fotometria Async -> DESABILITA comando EXPOSE para os ACS."
          n412 = call-dynamic "Read Channel.vi"("error in (no error)"=w1089, "Acquisition in"=w1090) -> ("error out"=w1076:errorcluster, "Channel.lvclass"=w1078:refnum<class "Channel.lvclass">, "Acquisition out"=w1098:refnum<class "Acquisition.lvclass">)  [unwired: 7 in]
          n413 = call-dynamic "Write wait_expose.vi"("error in (no error)"=w1076, "wait_expose"=FALSE, "Channel in"=w1078) -> ("error out"=w1075:errorcluster, "Channel out"=w1077:refnum<class "Channel.lvclass">)  [unwired: 7 in]
          n414 = call-dynamic "Read State Machine.vi"("error in (no error)"=w1075, "Device in"=w1077) -> ("error out"=w1095:errorcluster, "State Machine.lvclass"=w1097:refnum<class "State Machine.lvclass">, "Device out"=w1093:refnum<class "Channel.lvclass">)  [unwired: 7 in]
          n415 = call "Next State.vi"("error in (no error)"=w1095, "New_State"=40, "State Machine in"=w1097) -> ("error out"=w1082:errorcluster, "State Machine out"=w1083:refnum<class "State Machine.lvclass">)  [unwired: 7 in]
          n416 = call-dynamic "Write State Machine.vi"("error in (no error)"=w1082, "State Machine.lvclass"=w1083, "Device in"=w1093) -> ("error out"=w1092:errorcluster, "Device out"=w1094:refnum<class "Channel.lvclass">)  [unwired: 7 in]
          n417 = Increment(x=w1091) -> (x+1=w1088:u32)
          n418 = call-dynamic "Write Channel.vi"("error in (no error)"=w1092, "Channel.lvclass"=w1094, "Acquisition in"=w1098) -> ("error out"=w1087:errorcluster, "Acquisition out"=w1086:refnum<class "Acquisition.lvclass">)  [unwired: 7 in]
          n419 = call-dynamic "Write Acq_state.vi"("error in (no error)"=w1087, "Acq_state"=w1088, "Acquisition in"=w1086) -> ("error out"=w1084:errorcluster, "Acquisition out"=w1085:refnum<class "Acquisition.lvclass">)  [unwired: 7 in]
          n420 = Bundle By Name(cluster=w1081, "Error Msg"="") -> (w1079:refnum<class "S4GUI.lvclass">)
        }
        frame 322 {
          # "Espera canal voltar para IDLE"
          n421 = call-dynamic "Read Channel.vi"("error in (no error)"=w1114, "Acquisition in"=w1115) -> ("error out"=w1105:errorcluster, "Channel.lvclass"=w1106:refnum<class "Channel.lvclass">, "Acquisition out"=w1107:refnum<class "Acquisition.lvclass">)  [unwired: 7 in]
          n422 = call-dynamic "Read State Machine.vi"("error in (no error)"=w1105, "Device in"=w1106) -> ("error out"=w1108:errorcluster, "State Machine.lvclass"=w1110:refnum<class "State Machine.lvclass">)  [unwired: 7 in, 1 out]
          n423 = call-dynamic "Read State.vi"("error in (no error)"=w1108, "State Machine in"=w1110) -> ("error out"=w1103:errorcluster, "State"=w1109:i32)  [unwired: 7 in, 1 out]
          n424 = Equal?(x=0, y=w1109) -> (x = y?=w1099:bool)
          n425 = Increment(x=w1101) -> (x+1=w1102:u32)
          n426 = Select(t=w1102, s=w1099, f=w1101) -> (s? t:f=w1104:u32)
          n427 = call-dynamic "Write Acq_state.vi"("error in (no error)"=w1103, "Acq_state"=w1104, "Acquisition in"=w1107) -> ("error out"=w1112:errorcluster, "Acquisition out"=w1113:refnum<class "Acquisition.lvclass">)  [unwired: 7 in]
        }
        frame 323 {
          # "Envia: EXPOSE para o ACS"
          # "Dispara o comando para o dispositivo corrente."
          n428 = flat-sequence {
            tunnel: w1117 -> [w1139]
            tunnel: [w1139] -> w1116
            frame #0 {
              n429 = Tick Count (ms)() -> (millisecond timer value=w1140:u32)
              n430 = local write "time 2"(w1140) -> ()
            }
          }
          n431 = call-dynamic "Read Channel.vi"("error in (no error)"=w1116, "Acquisition in"=w1128) -> ("error out"=w1134:errorcluster, "Channel.lvclass"=w1133:refnum<class "Channel.lvclass">, "Acquisition out"=w1138:refnum<class "Acquisition.lvclass">)  [unwired: 7 in]
          n432 = call-dynamic "Read State Machine.vi"("error in (no error)"=w1134, "Device in"=w1133) -> ("error out"=w1135:errorcluster, "State Machine.lvclass"=w1137:refnum<class "State Machine.lvclass">, "Device out"=w1131:refnum<class "Channel.lvclass">)  [unwired: 7 in]
          n433 = call "Next State.vi"("error in (no error)"=w1135, "New_State"=50, "State Machine in"=w1137) -> ("error out"=w1121:errorcluster, "State Machine out"=w1122:refnum<class "State Machine.lvclass">)  [unwired: 7 in]
          n434 = call-dynamic "Write State Machine.vi"("error in (no error)"=w1121, "State Machine.lvclass"=w1122, "Device in"=w1131) -> ("error out"=w1130:errorcluster, "Device out"=w1132:refnum<class "Channel.lvclass">)  [unwired: 7 in]
          n435 = Increment(x=w1129) -> (x+1=w1125:u32)
          n436 = call-dynamic "Write Channel.vi"("error in (no error)"=w1130, "Channel.lvclass"=w1132, "Acquisition in"=w1138) -> ("error out"=w1124:errorcluster, "Acquisition out"=w1126:refnum<class "Acquisition.lvclass">)  [unwired: 7 in]
          n437 = call-dynamic "Write Acq_state.vi"("error in (no error)"=w1124, "Acq_state"=w1125, "Acquisition in"=w1126) -> ("error out"=w1123:errorcluster, "Acquisition out"=w1127:refnum<class "Acquisition.lvclass">)  [unwired: 7 in]
          n438 = Bundle By Name(cluster=w1120, "Error Msg"="") -> (w1119:refnum<class "S4GUI.lvclass">)
        }
        frame 324 {
          # "Espera Status Detector entrar em ACTIVE"
          n439 = call-dynamic "Read Channel.vi"("error in (no error)"=w1155, "Acquisition in"=w1154) -> ("error out"=w1141:errorcluster, "Channel.lvclass"=w1142:refnum<class "Channel.lvclass">, "Acquisition out"=w1169:refnum<class "Acquisition.lvclass">)  [unwired: 7 in]
          n440 = call-dynamic "Read wait_expose.vi"("error in (no error)"=w1141, "Channel in"=w1142) -> ("error out"=w1150:errorcluster, "wait_expose"=w1148:bool, "Channel out"=w1151:refnum<class "Channel.lvclass">)  [unwired: 7 in]
          n441 = call-dynamic "Read State Machine.vi"("error in (no error)"=w1150, "Device in"=w1151) -> ("error out"=w1163:errorcluster, "State Machine.lvclass"=w1165:refnum<class "State Machine.lvclass">, "Device out"=w1167:refnum<class "Channel.lvclass">)  [unwired: 7 in]
          n442 = call-dynamic "Read State.vi"("error in (no error)"=w1163, "State Machine in"=w1165) -> ("error out"=w1162:errorcluster, "State"=w1153:i32, "State Machine out"=w1164:refnum<class "State Machine.lvclass">)  [unwired: 7 in]
          n443 = Greater?(x=w1153, y=53) -> (0:w1143:bool)
          n444 = call-dynamic "Write State Machine.vi"("error in (no error)"=w1162, "State Machine.lvclass"=w1164, "Device in"=w1167) -> ("error out"=w1166:errorcluster, "Device out"=w1168:refnum<class "Channel.lvclass">)  [unwired: 7 in]
          n445 = call-dynamic "Write Channel.vi"("error in (no error)"=w1166, "Channel.lvclass"=w1168, "Acquisition in"=w1169) -> ("error out"=w1156:errorcluster, "Acquisition out"=w1157:refnum<class "Acquisition.lvclass">)  [unwired: 7 in]
          n446 = Increment(x=w1161) -> (x+1=w1147:u32)
          n447 = Select(t=327 ("y"), s=w1148, f=w1147) -> (s? t:f=w1146:u32)
          n448 = Select(t=w1146, s=w1143, f=w1161) -> (s? t:f=w1159:u32)
          n449 = call-dynamic "Write Acq_state.vi"("error in (no error)"=w1156, "Acq_state"=w1159, "Acquisition in"=w1157) -> ("error out"=w1158:errorcluster, "Acquisition out"=w1160:refnum<class "Acquisition.lvclass">)  [unwired: 7 in]
          n450 = flat-sequence {
            tunnel: [w1170] -> w1145
            tunnel: w1144 -> [w1170]
            frame #0 {
              n451 = Tick Count (ms)() -> (millisecond timer value=w1171:u32)
              n452 = local write "time307"(w1171) -> ()
            }
          }
        }
        frame 325 {
          # "Dispara o comando para o dispositivo corrente."
          n453 = call-dynamic "Read Channel.vi"("error in (no error)"=w1172, "Acquisition in"=w1177) -> ("error out"=w1178:errorcluster, "Channel.lvclass"=w1173:refnum<class "Channel.lvclass">, "Acquisition out"=w1175:refnum<class "Acquisition.lvclass">)  [unwired: 7 in]
          n454 = call-dynamic "Read wait_expose.vi"("error in (no error)"=w1178, "Channel in"=w1173) -> ("error out"=w1174:errorcluster, "wait_expose"=w1176:bool)  [unwired: 7 in, 1 out]
          n455 = case shown="False" w1176 {
            tunnel: w1175 -> [w1189 w1195]
            tunnel: w1174 -> [w1188 w1194]
            tunnel: [w1189 w1193] -> w1185
            tunnel: [w1188 w1192] -> w1183
            frame False {
            }
            frame True {
              n456 = call-dynamic "Read Channel.vi"("error in (no error)"=w1194, "Acquisition in"=w1195) -> ("error out"=w1200:errorcluster, "Channel.lvclass"=w1199:refnum<class "Channel.lvclass">, "Acquisition out"=w1204:refnum<class "Acquisition.lvclass">)  [unwired: 7 in]
              n457 = call-dynamic "Read State Machine.vi"("error in (no error)"=w1200, "Device in"=w1199) -> ("error out"=w1201:errorcluster, "State Machine.lvclass"=w1203:refnum<class "State Machine.lvclass">, "Device out"=w1197:refnum<class "Channel.lvclass">)  [unwired: 7 in]
              n458 = call "Next State.vi"("error in (no error)"=w1201, "New_State"=50, "State Machine in"=w1203) -> ("error out"=w1190:errorcluster, "State Machine out"=w1191:refnum<class "State Machine.lvclass">)  [unwired: 7 in]
              n459 = call-dynamic "Write State Machine.vi"("error in (no error)"=w1190, "State Machine.lvclass"=w1191, "Device in"=w1197) -> ("error out"=w1196:errorcluster, "Device out"=w1198:refnum<class "Channel.lvclass">)  [unwired: 7 in]
              n460 = call-dynamic "Write Channel.vi"("error in (no error)"=w1196, "Channel.lvclass"=w1198, "Acquisition in"=w1204) -> ("error out"=w1192:errorcluster, "Acquisition out"=w1193:refnum<class "Acquisition.lvclass">)  [unwired: 7 in]
            }
          }
          n461 = Increment(x=w1187) -> (x+1=w1184:u32)
          n462 = call-dynamic "Write Acq_state.vi"("error in (no error)"=w1183, "Acq_state"=w1184, "Acquisition in"=w1185) -> ("error out"=w1182:errorcluster, "Acquisition out"=w1186:refnum<class "Acquisition.lvclass">)  [unwired: 7 in]
          n463 = Bundle By Name(cluster=w1179, "Error Msg"="") -> (w1181:refnum<class "S4GUI.lvclass">)
        }
        frame 326 {
          # "Espera Status Detector entrar em ACTIVE"
          n464 = call-dynamic "Read Channel.vi"("error in (no error)"=w1215, "Acquisition in"=w1214) -> ("error out"=w1209:errorcluster, "Channel.lvclass"=w1210:refnum<class "Channel.lvclass">, "Acquisition out"=w1229:refnum<class "Acquisition.lvclass">)  [unwired: 7 in]
          n465 = call-dynamic "Read State Machine.vi"("error in (no error)"=w1209, "Device in"=w1210) -> ("error out"=w1223:errorcluster, "State Machine.lvclass"=w1225:refnum<class "State Machine.lvclass">, "Device out"=w1227:refnum<class "Channel.lvclass">)  [unwired: 7 in]
          n466 = call-dynamic "Read State.vi"("error in (no error)"=w1223, "State Machine in"=w1225) -> ("error out"=w1222:errorcluster, "State"=w1213:i32, "State Machine out"=w1224:refnum<class "State Machine.lvclass">)  [unwired: 7 in]
          n467 = Greater?(x=w1213, y=53) -> (0:w1221:bool)
          n468 = call-dynamic "Write State Machine.vi"("error in (no error)"=w1222, "State Machine.lvclass"=w1224, "Device in"=w1227) -> ("error out"=w1226:errorcluster, "Device out"=w1228:refnum<class "Channel.lvclass">)  [unwired: 7 in]
          n469 = call-dynamic "Write Channel.vi"("error in (no error)"=w1226, "Channel.lvclass"=w1228, "Acquisition in"=w1229) -> ("error out"=w1216:errorcluster, "Acquisition out"=w1217:refnum<class "Acquisition.lvclass">)  [unwired: 7 in]
          n470 = Increment(x=w1207) -> (x+1=w1206:u32)
          n471 = Select(t=u32 328, s=w1221, f=w1206) -> (s? t:f=w1219:u32)
          n472 = call-dynamic "Write Acq_state.vi"("error in (no error)"=w1216, "Acq_state"=w1219, "Acquisition in"=w1217) -> ("error out"=w1218:errorcluster, "Acquisition out"=w1220:refnum<class "Acquisition.lvclass">)  [unwired: 7 in]
          n473 = flat-sequence {
            tunnel: [w1231] -> w1211
            tunnel: w1208 -> [w1231]
            frame #0 {
              n474 = Tick Count (ms)() -> (millisecond timer value=w1230:u32)
              n475 = local write "time307"(w1230) -> ()
            }
          }
        }
        frame 327 {
          # "Dispara o comando para o dispositivo corrente."
          n476 = call "Read id.vi"("error in (no error)"=w1237, "Server in"=w1238) -> ("error out"=w1235:errorcluster, "id"=w1234:u32, "Server out"=w1236:refnum<class "Acquisition.lvclass">)  [unwired: 7 in]
          n477 = call-dynamic "Read Channel.vi"("error in (no error)"=w1235, "Acquisition in"=w1236) -> ("error out"=w1247:errorcluster, "Channel.lvclass"=w1248:refnum<class "Channel.lvclass">, "Acquisition out"=w1258:refnum<class "Acquisition.lvclass">)  [unwired: 7 in]
          n478 = Increment(x=w1234) -> (x+1=w1233:u32)
          n479 = call-dynamic "Read PrevCyclesDone.vi"("error in (no error)"=w1247, "Channel in"=w1248) -> ("error out"=w1250:errorcluster, "PrevCyclesDone"=w1249:u32, "Channel out"=w1251:refnum<class "Channel.lvclass">)  [unwired: 7 in]
          n480 = call-dynamic "Read CyclesDone.vi"("error in (no error)"=w1250, "Channel in"=w1251) -> ("error out"=w1244:errorcluster, "CyclesDone"=w1239:u32, "Channel out"=w1246:refnum<class "Channel.lvclass">)  [unwired: 7 in]
          n481 = Increment(x=w1249) -> (x+1=w1232:u32)
          n482 = call-dynamic "Read stopping.vi"("error in (no error)"=w1244, "Channel in"=w1246) -> ("error out"=w1243:errorcluster, "stopping"=w1241:bool, "Channel out"=w1245:refnum<class "Channel.lvclass">)  [unwired: 7 in]
          n483 = Equal?(x=w1239, y=w1232) -> (x = y?=w1242:bool)
          n484 = call-dynamic "Write Channel.vi"("error in (no error)"=w1243, "Channel.lvclass"=w1245, "Acquisition in"=w1258) -> ("error out"=w1254:errorcluster, "Acquisition out"=w1255:refnum<class "Acquisition.lvclass">)  [unwired: 7 in]
          n485 = case shown="False" w1242 {
            tunnel: [w1267 w1308] -> w1256
            tunnel: w1255 -> [w1263 w1296]
            tunnel: w1257 -> [w1261 w1307]
            tunnel: w1254 -> [w1264 w1295]
            tunnel: [w1269 w1305] -> w1253
            tunnel: w1252 -> [w1270 w1303]
            tunnel: w1241 -> [_ w1301]
            tunnel: [w1268 w1306] -> w1240
            tunnel: w1239 -> [_ w1300]
            tunnel: w1233 -> [w1266 _]
            frame False {
              # "Aguardando iniciar exposição por 5s"
              n486 = local read "time 2"() -> (w1260:u32)
              n487 = Tick Count (ms)() -> (millisecond timer value=w1273:u32)
              n488 = Subtract(x=w1273, y=w1260) -> (x-y=w1272:u32)
              n489 = To Double Precision Float(number=w1272) -> (double precision float=w1271:dbl)
              n490 = Number To Decimal String(number=w1266) -> (decimal integer string=w1265:string)  [unwired: 1 in]
              n491 = Less?(x=5000.0, y=w1271) -> ()  [unwired: 1 out]
              n492 = case shown="False" FALSE {
                tunnel: w1270 -> [w1280 w1290]
                tunnel: [w1280 w1289] -> w1269
                tunnel: [w1275 w1286] -> w1268
                tunnel: w1264 -> [w1276 w1285]
                tunnel: w1263 -> [w1279 w1288]
                tunnel: [w1277 w1287] -> w1267
                tunnel: w1265 -> [_ w1282]
                tunnel: w1261 -> [w1278 _]
                frame False {
                  # "Volta para esperar ACTIVE."
                  n493 = Decrement(x=w1278) -> (x-1=w1274:u32)
                  n494 = call-dynamic "Write Acq_state.vi"("error in (no error)"=w1276, "Acq_state"=w1274, "Acquisition in"=w1279) -> ("error out"=w1275:errorcluster, "Acquisition out"=w1277:refnum<class "Acquisition.lvclass">)  [unwired: 7 in]
                }
                frame True {
                  n495 = Concatenate Strings("ERROR: Init Acquisition Timeout. HandleObservationAsync.vi - state 327. Channel: ", w1282) -> (w1281:string)
                  n496 = call-dynamic "Write Acq_state.vi"("error in (no error)"=w1285, "Acq_state"=u32 1, "Acquisition in"=w1288) -> ("error out"=w1286:errorcluster, "Acquisition out"=w1287:refnum<class "Acquisition.lvclass">)  [unwired: 7 in]
                  n497 = Bundle By Name(cluster=w1290, "Error Msg"=w1281) -> (w1289:refnum<class "S4GUI.lvclass">)
                }
              }
            }
            frame True {
              # "STOP?"
              # "Avançou o ciclo."
              n498 = call-dynamic "Read Channel.vi"("error in (no error)"=w1295, "Acquisition in"=w1296) -> ("error out"=w1294:errorcluster, "Channel.lvclass"=w1299:refnum<class "Channel.lvclass">, "Acquisition out"=w1297:refnum<class "Acquisition.lvclass">)  [unwired: 7 in]
              n499 = call-dynamic "Write PrevCyclesDone.vi"("error in (no error)"=w1294, "PrevCyclesDone"=w1300, "Channel in"=w1299) -> ("error out"=w1293:errorcluster, "Channel out"=w1298:refnum<class "Channel.lvclass">)  [unwired: 7 in]
              n500 = call-dynamic "Write Channel.vi"("error in (no error)"=w1293, "Channel.lvclass"=w1298, "Acquisition in"=w1297) -> ("error out"=w1291:errorcluster, "Acquisition out"=w1292:refnum<class "Acquisition.lvclass">)  [unwired: 7 in]
              n501 = case shown="False" w1301 {
                tunnel: w1307 -> [w1311 _]
                tunnel: [w1309 u32 0] -> w1302
                frame False {
                  n502 = Increment(x=w1311) -> (x+1=w1310:u32)
                  n503 = Increment(x=w1310) -> (x+1=w1309:u32)
                }
                frame True {
                }
              }
              n504 = call-dynamic "Write Acq_state.vi"("error in (no error)"=w1291, "Acq_state"=w1302, "Acquisition in"=w1292) -> ("error out"=w1306:errorcluster, "Acquisition out"=w1308:refnum<class "Acquisition.lvclass">)  [unwired: 7 in]
              n505 = Bundle By Name(cluster=w1303, "Error Msg"="") -> (w1305:refnum<class "S4GUI.lvclass">)
            }
          }
        }
        frame 328 {
          # "Dispara o comando para o dispositivo corrente."
          n506 = call "Read id.vi"("error in (no error)"=w1318, "Server in"=w1319) -> ("error out"=w1316:errorcluster, "id"=w1315:u32, "Server out"=w1317:refnum<class "Acquisition.lvclass">)  [unwired: 7 in]
          n507 = call-dynamic "Read Channel.vi"("error in (no error)"=w1316, "Acquisition in"=w1317) -> ("error out"=w1328:errorcluster, "Channel.lvclass"=w1329:refnum<class "Channel.lvclass">, "Acquisition out"=w1339:refnum<class "Acquisition.lvclass">)  [unwired: 7 in]
          n508 = Increment(x=w1315) -> (x+1=w1314:u32)
          n509 = call-dynamic "Read PrevCyclesDone.vi"("error in (no error)"=w1328, "Channel in"=w1329) -> ("error out"=w1331:errorcluster, "PrevCyclesDone"=w1330:u32, "Channel out"=w1332:refnum<class "Channel.lvclass">)  [unwired: 7 in]
          n510 = call-dynamic "Read CyclesDone.vi"("error in (no error)"=w1331, "Channel in"=w1332) -> ("error out"=w1325:errorcluster, "CyclesDone"=w1320:u32, "Channel out"=w1327:refnum<class "Channel.lvclass">)  [unwired: 7 in]
          n511 = Increment(x=w1330) -> (x+1=w1313:u32)
          n512 = call-dynamic "Read stopping.vi"("error in (no error)"=w1325, "Channel in"=w1327) -> ("error out"=w1324:errorcluster, "stopping"=w1322:bool, "Channel out"=w1326:refnum<class "Channel.lvclass">)  [unwired: 7 in]
          n513 = Equal?(x=w1320, y=w1313) -> (x = y?=w1323:bool)
          n514 = call-dynamic "Write Channel.vi"("error in (no error)"=w1324, "Channel.lvclass"=w1326, "Acquisition in"=w1339) -> ("error out"=w1335:errorcluster, "Acquisition out"=w1336:refnum<class "Acquisition.lvclass">)  [unwired: 7 in]
          n515 = case shown="False" w1323 {
            tunnel: [w1345 w1390] -> w1337
            tunnel: w1336 -> [w1357 w1378]
            tunnel: w1338 -> [_ w1389]
            tunnel: w1335 -> [w1356 w1377]
            tunnel: [w1349 w1387] -> w1334
            tunnel: w1333 -> [w1350 w1385]
            tunnel: w1322 -> [_ w1383]
            tunnel: [w1347 w1388] -> w1321
            tunnel: w1320 -> [_ w1382]
            tunnel: w1314 -> [w1344 _]
            frame False {
              n516 = Tick Count (ms)() -> (millisecond timer value=w1359:u32)
              n517 = local read "time307"() -> (w1358:u32)
              n518 = call-dynamic "GetCubeDuration.vi"("error in (no error)"=w1356, "Acquisition in"=w1357) -> ("error out"=w1348:errorcluster, "Acquisition out"=w1346:refnum<class "Acquisition.lvclass">, "CubeDuration"=w1342:dbl)  [unwired: 7 in]
              n519 = Subtract(x=w1359, y=w1358) -> (x-y=w1353:u32)
              n520 = Multiply(x=w1342, y=1000.0) -> (x*y=w1340:dbl)
              n521 = To Double Precision Float(number=w1353) -> (double precision float=w1351:dbl)
              n522 = Add(x=1000.0, y=w1340) -> (x+y=w1354:dbl)
              n523 = Number To Decimal String(number=w1344) -> (decimal integer string=w1343:string)  [unwired: 1 in]
              n524 = Less?(x=w1354, y=w1351) -> (x < y?=w1352:bool)
              n525 = case shown="True" w1352 {
                tunnel: w1350 -> [w1362 w1372]
                tunnel: [w1362 w1371] -> w1349
                tunnel: [w1361 w1368] -> w1347
                tunnel: w1348 -> [w1361 w1367]
                tunnel: w1346 -> [w1360 w1370]
                tunnel: [w1360 w1369] -> w1345
                tunnel: w1343 -> [_ w1364]
                frame False {
                }
                frame True {
                  n526 = Concatenate Strings("ERROR: Acquisition Timeout. HandleObservationAsync.vi - state 328. Channel: ", w1364) -> (w1363:string)
                  n527 = call-dynamic "Write Acq_state.vi"("error in (no error)"=w1367, "Acq_state"=u32 1, "Acquisition in"=w1370) -> ("error out"=w1368:errorcluster, "Acquisition out"=w1369:refnum<class "Acquisition.lvclass">)  [unwired: 7 in]
                  n528 = Bundle By Name(cluster=w1372, "Error Msg"=w1363) -> (w1371:refnum<class "S4GUI.lvclass">)
                }
              }
            }
            frame True {
              n529 = call-dynamic "Read Channel.vi"("error in (no error)"=w1377, "Acquisition in"=w1378) -> ("error out"=w1376:errorcluster, "Channel.lvclass"=w1381:refnum<class "Channel.lvclass">, "Acquisition out"=w1379:refnum<class "Acquisition.lvclass">)  [unwired: 7 in]
              n530 = call-dynamic "Write PrevCyclesDone.vi"("error in (no error)"=w1376, "PrevCyclesDone"=w1382, "Channel in"=w1381) -> ("error out"=w1375:errorcluster, "Channel out"=w1380:refnum<class "Channel.lvclass">)  [unwired: 7 in]
              n531 = call-dynamic "Write Channel.vi"("error in (no error)"=w1375, "Channel.lvclass"=w1380, "Acquisition in"=w1379) -> ("error out"=w1373:errorcluster, "Acquisition out"=w1374:refnum<class "Acquisition.lvclass">)  [unwired: 7 in]
              n532 = case shown="False" w1383 {
                tunnel: w1389 -> [w1392 _]
                tunnel: [w1391 u32 0] -> w1384
                frame False {
                  n533 = Increment(x=w1392) -> (x+1=w1391:u32)
                }
                frame True {
                }
              }
              n534 = call-dynamic "Write Acq_state.vi"("error in (no error)"=w1373, "Acq_state"=w1384, "Acquisition in"=w1374) -> ("error out"=w1388:errorcluster, "Acquisition out"=w1390:refnum<class "Acquisition.lvclass">)  [unwired: 7 in]
              n535 = Bundle By Name(cluster=w1385, "Error Msg"="") -> (w1387:refnum<class "S4GUI.lvclass">)
            }
          }
        }
        frame 329 {
          n536 = call-dynamic "Read Channel.vi"("error in (no error)"=w1410, "Acquisition in"=w1411) -> ("error out"=w1399:errorcluster, "Channel.lvclass"=w1409:refnum<class "Channel.lvclass">, "Acquisition out"=w1394:refnum<class "Acquisition.lvclass">)  [unwired: 7 in]
          n537 = call-dynamic "Read CyclesDone.vi"("error in (no error)"=w1399, "Channel in"=w1409) -> ("error out"=w1412:errorcluster, "CyclesDone"=w1407:u32, "Channel out"=w1413:refnum<class "Channel.lvclass">)  [unwired: 7 in]
          n538 = call-dynamic "Read ciclos.vi"("error in (no error)"=w1412, "Channel in"=w1413) -> ("error out"=w1398:errorcluster, "ciclos"=w1408:u32, "Channel out"=w1397:refnum<class "Channel.lvclass">)  [unwired: 7 in]
          n539 = Subtract(x=w1408, y=w1407) -> (x-y=w1414:u32)
          n540 = Greater Than 0?(x=w1414) -> (x > 0?=w1402:bool)
          n541 = call-dynamic "Read wait_expose.vi"("error in (no error)"=w1398, "Channel in"=w1397) -> ("error out"=w1395:errorcluster, "wait_expose"=w1396:bool)  [unwired: 7 in, 1 out]
          n542 = Select(t=u32 323, s=w1396, f=u32 325 ("t")) -> (s? t:f=w1401:u32)
          n543 = Select(t=w1401, s=w1402, f=u32 0) -> (s? t:f=w1403:u32)
          n544 = call-dynamic "Write Acq_state.vi"("error in (no error)"=w1395, "Acq_state"=w1403, "Acquisition in"=w1394) -> ("error out"=w1415:errorcluster, "Acquisition out"=w1416:refnum<class "Acquisition.lvclass">)  [unwired: 7 in]
        }
        frame 1325 {
          n545 = disable-structure shown="Enabled" {
            disable-tunnel: w1422 -> [w1438 w1466]
            disable-tunnel: w1421 -> [w1437 w1465]
            disable-tunnel: [w1430 w1461] -> w1420
            disable-tunnel: [w1424 w1462] -> w1419
            disable-tunnel: w1417 -> [_ _]
            disable-tunnel: w1418 -> [_ w1460]
            frame Disabled {
              n546 = call-dynamic "Read Channel.vi"("error in (no error)"=w1437, "Acquisition in"=w1438) -> ("error out"=w1435:errorcluster, "Channel.lvclass"=w1436:refnum<class "Channel.lvclass">, "Acquisition out"=w1432:refnum<class "Acquisition.lvclass">)  [unwired: 7 in]
              n547 = call-dynamic "Read ciclos.vi"("error in (no error)"=w1435, "Channel in"=w1436) -> ("error out"=w1427:errorcluster, "ciclos"=w1434:u32, "Channel out"=w1428:refnum<class "Channel.lvclass">)  [unwired: 7 in]
              n548 = Decrement(x=w1434) -> (x-1=w1439:u32)
              n549 = Greater Than 0?(x=w1439) -> (x > 0?=w1443:bool)
              n550 = case shown="True" w1443 {
                selector: w1443 -> [w1445 w1447]
                tunnel: w1439 -> [_ w1446]
                tunnel: [w1445 w1447] -> w1442
                tunnel: [u32 0 w1446] -> w1433
                frame False {
                }
                frame True {
                }
              }
              n551 = call-dynamic "Write ciclos.vi"("error in (no error)"=w1427, "ciclos"=w1433, "Channel in"=w1428) -> ("error out"=w1426:errorcluster, "Channel out"=w1429:refnum<class "Channel.lvclass">)  [unwired: 7 in]
              n552 = call-dynamic "Write Channel.vi"("error in (no error)"=w1426, "Channel.lvclass"=w1429, "Acquisition in"=w1432) -> ("error out"=w1425:errorcluster, "Acquisition out"=w1431:refnum<class "Acquisition.lvclass">)  [unwired: 7 in]
              n553 = Select(t=u32 323, s=w1442, f=u32 0) -> (s? t:f=w1423:u32)
              n554 = call-dynamic "Write Acq_state.vi"("error in (no error)"=w1425, "Acq_state"=w1423, "Acquisition in"=w1431) -> ("error out"=w1424:errorcluster, "Acquisition out"=w1430:refnum<class "Acquisition.lvclass">)  [unwired: 7 in]
            }
            frame Enabled {
              n555 = call-dynamic "Read Channel.vi"("error in (no error)"=w1465, "Acquisition in"=w1466) -> ("error out"=w1456:errorcluster, "Channel.lvclass"=w1458:refnum<class "Channel.lvclass">, "Acquisition out"=w1467:refnum<class "Acquisition.lvclass">)  [unwired: 7 in]
              n556 = call-dynamic "Read PrevCyclesDone.vi"("error in (no error)"=w1456, "Channel in"=w1458) -> ("error out"=w1455:errorcluster, "PrevCyclesDone"=w1454:u32, "Channel out"=w1457:refnum<class "Channel.lvclass">)  [unwired: 7 in]
              n557 = call-dynamic "Read CyclesDone.vi"("error in (no error)"=w1455, "Channel in"=w1457) -> ("error out"=w1451:errorcluster, "CyclesDone"=w1463:u32, "Channel out"=w1453:refnum<class "Channel.lvclass">)  [unwired: 7 in]
              n558 = Greater?(x=w1463, y=w1454) -> (0:w1464:bool)
              n559 = case shown="True" w1464 {
                tunnel: w1463 -> [_ w1471]
                tunnel: w1460 -> [w1470 w1477]
                tunnel: [w1470 w1476] -> w1459
                tunnel: [w1469 w1474] -> w1452
                tunnel: w1453 -> [w1469 w1475]
                tunnel: w1451 -> [w1468 w1473]
                tunnel: [w1468 w1472] -> w1450
                frame False {
                }
                frame True {
                  n560 = call-dynamic "Write PrevCyclesDone.vi"("error in (no error)"=w1473, "PrevCyclesDone"=w1471, "Channel in"=w1475) -> ("error out"=w1472:errorcluster, "Channel out"=w1474:refnum<class "Channel.lvclass">)  [unwired: 7 in]
                  n561 = Increment(x=w1477) -> (x+1=w1476:u32)
                }
              }
              n562 = call-dynamic "Write Channel.vi"("error in (no error)"=w1450, "Channel.lvclass"=w1452, "Acquisition in"=w1467) -> ("error out"=w1449:errorcluster, "Acquisition out"=w1448:refnum<class "Acquisition.lvclass">)  [unwired: 7 in]
              n563 = call-dynamic "Write Acq_state.vi"("error in (no error)"=w1449, "Acq_state"=w1459, "Acquisition in"=w1448) -> ("error out"=w1462:errorcluster, "Acquisition out"=w1461:refnum<class "Acquisition.lvclass">)  [unwired: 7 in]
            }
          }
        }
        frame 1326 {
          n564 = call-dynamic "Read Channel.vi"("error in (no error)"=w1485, "Acquisition in"=w1486) -> ("error out"=w1481:errorcluster, "Channel.lvclass"=w1484:refnum<class "Channel.lvclass">, "Acquisition out"=w1482:refnum<class "Acquisition.lvclass">)  [unwired: 7 in]
          n565 = call-dynamic "Read CyclesDone.vi"("Channel in"=w1484) -> ("error out"=w1478:errorcluster, "CyclesDone"=w1479:u32, "Channel out"=w1483:refnum<class "Channel.lvclass">)  [unwired: 8 in]
          n566 = call-dynamic "Read ciclos.vi"("error in (no error)"=w1478, "Channel in"=w1483) -> ("ciclos"=w1480:u32)  [unwired: 7 in, 2 out]
          n567 = Unbundle By Name(w1491) -> ("mode EXPOSE"=w1490:bool)
          n568 = Subtract(x=w1480, y=w1479) -> (x-y=w1497:u32)
          n569 = Select(t=u32 323, s=w1490, f=u32 325 ("t")) -> (s? t:f=w1487:u32)
          n570 = Greater Than 0?(x=w1497) -> (x > 0?=w1496:bool)
          n571 = Select(t=w1487, s=w1496, f=u32 0) -> (s? t:f=w1494:u32)
          n572 = call-dynamic "Write Acq_state.vi"("error in (no error)"=w1481, "Acq_state"=w1494, "Acquisition in"=w1482) -> ("error out"=w1492:errorcluster, "Acquisition out"=w1493:refnum<class "Acquisition.lvclass">)  [unwired: 7 in]
        }
        frame 360 {
          w1503 = u32 0 ("cyclesDone")
          # "Inicia o Ticks com\nvalor do relogio atual"
          # "Espera até 40 x 0.25s (= 10s) para\nmecanismo entrar em READY"
          # "Busca próximo valor de foco..."
          n573 = flat-sequence {
            tunnel: w1506 -> [w1533]
            tunnel: [w1533] -> w1523
            frame #0 {
              n574 = Tick Count (ms)() -> (millisecond timer value=→"time7":u32)
            }
          }
          n575 = call-dynamic "Read TelFocus.lvclass.vi"("error in (no error)"=w1523, "S4GUI in"=w1507) -> ("error out"=w1531:errorcluster, "TelFocus.lvclass"=w1532:refnum<class "TelFocus.lvclass">, "S4GUI out"=w1530:refnum<class "S4GUI.lvclass">)  [unwired: 7 in]
          n576 = call-dynamic "GetNextFocus.vi"("error in (no error)"=w1531, "TelFocus in"=w1532) -> ("error out"=w1521:errorcluster, "TelFocus out"=w1522:refnum<class "TelFocus.lvclass">)  [unwired: 8 in]
          n577 = call-dynamic "Read SecMirror.lvclass.vi"("error in (no error)"=w1521, "TelFocus in"=w1522) -> ("error out"=w1508:errorcluster, "SecMirror.lvclass"=w1509:refnum<class "SecMirror.lvclass">, "TelFocus out"=w1525:refnum<class "TelFocus.lvclass">)  [unwired: 7 in]
          n578 = call-dynamic "Read State Machine.vi"("error in (no error)"=w1508, "Device in"=w1509) -> ("error out"=w1518:errorcluster, "State Machine.lvclass"=w1520:refnum<class "State Machine.lvclass">, "Device out"=w1517:refnum<class "SecMirror.lvclass">)  [unwired: 7 in]
          n579 = call "Next State.vi"("error in (no error)"=w1518, "New_State"=1, "State Machine in"=w1520) -> ("error out"=w1515:errorcluster, "State Machine out"=w1516:refnum<class "State Machine.lvclass">)  [unwired: 7 in]
          n580 = call-dynamic "Write Timer.vi"("error in (no error)"=w1515, "Timer"=u32 40, "State Machine in"=w1516) -> ("error out"=w1512:errorcluster, "State Machine out"=w1513:refnum<class "State Machine.lvclass">)  [unwired: 7 in]
          n581 = call-dynamic "Init Ticks2.vi"("error in (no error)"=w1512, "State Machine in"=w1513) -> ("error out"=w1511:errorcluster, "State Machine out"=w1510:refnum<class "State Machine.lvclass">)  [unwired: 8 in]
          n582 = call-dynamic "Write State Machine.vi"("error in (no error)"=w1511, "State Machine.lvclass"=w1510, "Device in"=w1517) -> ("error out"=w1524:errorcluster, "Device out"=w1526:refnum<class "SecMirror.lvclass">)  [unwired: 7 in]
          n583 = call-dynamic "Write SecMirror.lvclass.vi"("error in (no error)"=w1524, "SecMirror.lvclass"=w1526, "TelFocus in"=w1525) -> ("error out"=w1528:errorcluster, "TelFocus out"=w1527:refnum<class "TelFocus.lvclass">)  [unwired: 7 in]
          n584 = call-dynamic "Write TelFocus.lvclass.vi"("error in (no error)"=w1528, "TelFocus.lvclass"=w1527, "S4GUI in"=w1530) -> ("error out"=w1500:errorcluster, "S4GUI out"=w1529:refnum<class "S4GUI.lvclass">)  [unwired: 7 in]
          n585 = Bundle By Name(cluster=w1529, "cyclesDone"=w1503, "sequesDone"=w1503) -> (w1504:refnum<class "S4GUI.lvclass">)
          n586 = Increment(x=w1505) -> (x+1=w1499:u32)
          n587 = call-dynamic "Write Acq_state.vi"("error in (no error)"=w1500, "Acq_state"=w1499, "Acquisition in"=w1502) -> ("error out"=w1498:errorcluster, "Acquisition out"=w1501:refnum<class "Acquisition.lvclass">)  [unwired: 7 in]
        }
        frame 361 {
          # "Timeout= 25s + distancia do target (cada 1000um=1s)"
          # "Espera terminar o movimento do foco do 2ndario para disparar\n a aquisição do canal."
          n588 = flat-sequence {
            tunnel: w1555 -> [w1591]
            tunnel: [w1591] -> w1571
            frame #0 {
              n589 = Tick Count (ms)() -> (millisecond timer value=w1590:u32)
              "time 8" <- w1590
              n590 = local read "time7"() -> (w1589:u32)
              n591 = Subtract(x=w1590, y=w1589) -> (x-y=→"delay 78":u32)
            }
          }
          n592 = call-dynamic "Read TelFocus.lvclass.vi"("error in (no error)"=w1571, "S4GUI in"=w1556) -> ("error out"=w1580:errorcluster, "TelFocus.lvclass"=w1581:refnum<class "TelFocus.lvclass">, "S4GUI out"=w1577:refnum<class "S4GUI.lvclass">)  [unwired: 7 in]
          n593 = call-dynamic "Read SecMirror.lvclass.vi"("error in (no error)"=w1580, "TelFocus in"=w1581) -> ("error out"=w1544:errorcluster, "SecMirror.lvclass"=w1547:refnum<class "SecMirror.lvclass">, "TelFocus out"=w1579:refnum<class "TelFocus.lvclass">)  [unwired: 7 in]
          n594 = call-dynamic "Read position.vi"("error in (no error)"=w1544, "SecMirror in"=w1547) -> ("error out"=w1553:errorcluster, "position"=w1541:i32, "SecMirror out"=w1546:refnum<class "SecMirror.lvclass">)  [unwired: 7 in]
          n595 = call-dynamic "Read target.vi"("error in (no error)"=w1553, "SecMirror in"=w1546) -> ("error out"=w1543:errorcluster, "target"=w1552:i32, "SecMirror out"=w1545:refnum<class "SecMirror.lvclass">)  [unwired: 7 in]
          n596 = Subtract(x=w1552, y=w1541) -> (x-y=w1551:i32)
          n597 = Absolute Value(x=w1551) -> (abs(x)=w1549:i32)
          n598 = call-dynamic "Read State Machine.vi"("error in (no error)"=w1543, "Device in"=w1545) -> ("error out"=w1563:errorcluster, "State Machine.lvclass"=w1566:refnum<class "State Machine.lvclass">, "Device out"=w1574:refnum<class "SecMirror.lvclass">)  [unwired: 7 in]
          n599 = To Unsigned Long Integer(number=w1549) -> (unsigned 32bit integer=w1550:u32)
          n600 = Add(x=w1550, y=u32 25000 ("period")) -> (x+y=w1542:u32)
          n601 = call-dynamic "Verif Clock 2.vi"("error in (no error)"=w1563, "period (ms)"=w1542, "State Machine in"=w1566) -> ("error out"=w1562:errorcluster, "time elapsed"=→"time elapsed 2":u32, "State Machine out"=w1565:refnum<class "State Machine.lvclass">)  [unwired: 6 in]
          n602 = call-dynamic "Read Timeout 2.vi"("error in (no error)"=w1562, "State Machine in"=w1565) -> ("error out"=w1561:errorcluster, "Timeout 2"=w1567:bool, "State Machine out"=w1564:refnum<class "State Machine.lvclass">)  [unwired: 7 in]
          n603 = call-dynamic "Read State.vi"("error in (no error)"=w1561, "State Machine in"=w1564) -> ("error out"=w1569:errorcluster, "State"=w1572:i32, "State Machine out"=w1570:refnum<class "State Machine.lvclass">)  [unwired: 7 in]
          n604 = call-dynamic "Write State Machine.vi"("error in (no error)"=w1569, "State Machine.lvclass"=w1570, "Device in"=w1574) -> ("error out"=w1573:errorcluster, "Device out"=w1575:refnum<class "SecMirror.lvclass">)  [unwired: 7 in]
          n605 = call-dynamic "Write SecMirror.lvclass.vi"("error in (no error)"=w1573, "SecMirror.lvclass"=w1575, "TelFocus in"=w1579) -> ("error out"=w1576:errorcluster, "TelFocus out"=w1578:refnum<class "TelFocus.lvclass">)  [unwired: 7 in]
          n606 = call-dynamic "Write TelFocus.lvclass.vi"("error in (no error)"=w1576, "TelFocus.lvclass"=w1578, "S4GUI in"=w1577) -> ("error out"=w1538:errorcluster, "S4GUI out"=w1560:refnum<class "S4GUI.lvclass">)  [unwired: 7 in]
          n607 = Equal To 0?(x=w1572) -> (x = 0?=w1568:bool)
          n608 = case shown="True" w1567 {
            tunnel: w1554 -> [w1583 _]
            tunnel: [w1583 u32 0 ("Obs_state")] -> w1558
            tunnel: w1560 -> [w1582 w1587]
            tunnel: [w1582 w1586] -> w1540
            frame False {
            }
            frame True {
              n609 = Bundle By Name(cluster=w1587, "Error Msg"="ERROR: moving telescope focus timeout  (S4GUI:HandleObservationAsync.vi - state 361)") -> (w1586:refnum<class "S4GUI.lvclass">)
            }
          }
          n610 = Increment(x=w1558) -> (x+1=w1557:u32)
          n611 = Select(t=w1557, s=w1568, f=w1558) -> (s? t:f=w1535:u32)
          n612 = call-dynamic "Write Acq_state.vi"("error in (no error)"=w1538, "Acq_state"=w1535, "Acquisition in"=w1539) -> ("error out"=w1536:errorcluster, "Acquisition out"=w1537:refnum<class "Acquisition.lvclass">)  [unwired: 7 in]
        }
        frame 362 {
          # "Dispara o comando para o dispositivo corrente."
          n613 = call-dynamic "Read Channel.vi"("error in (no error)"=w1601, "Acquisition in"=w1602) -> ("error out"=w1608:errorcluster, "Channel.lvclass"=w1607:refnum<class "Channel.lvclass">, "Acquisition out"=w1612:refnum<class "Acquisition.lvclass">)  [unwired: 7 in]
          n614 = call-dynamic "Read State Machine.vi"("error in (no error)"=w1608, "Device in"=w1607) -> ("error out"=w1609:errorcluster, "State Machine.lvclass"=w1611:refnum<class "State Machine.lvclass">, "Device out"=w1605:refnum<class "Channel.lvclass">)  [unwired: 7 in]
          n615 = call "Next State.vi"("error in (no error)"=w1609, "New_State"=58, "State Machine in"=w1611) -> ("error out"=w1594:errorcluster, "State Machine out"=w1595:refnum<class "State Machine.lvclass">)  [unwired: 7 in]
          n616 = call-dynamic "Write State Machine.vi"("error in (no error)"=w1594, "State Machine.lvclass"=w1595, "Device in"=w1605) -> ("error out"=w1604:errorcluster, "Device out"=w1606:refnum<class "Channel.lvclass">)  [unwired: 7 in]
          n617 = Increment(x=w1603) -> (x+1=w1600:u32)
          n618 = call-dynamic "Write Channel.vi"("error in (no error)"=w1604, "Channel.lvclass"=w1606, "Acquisition in"=w1612) -> ("error out"=w1598:errorcluster, "Acquisition out"=w1597:refnum<class "Acquisition.lvclass">)  [unwired: 7 in]
          n619 = call-dynamic "Write Acq_state.vi"("error in (no error)"=w1598, "Acq_state"=w1600, "Acquisition in"=w1597) -> ("error out"=w1593:errorcluster, "Acquisition out"=w1596:refnum<class "Acquisition.lvclass">)  [unwired: 7 in]
          n620 = flat-sequence {
            tunnel: w1593 -> [w1613]
            tunnel: [w1613] -> w1592
            frame #0 {
              n621 = Tick Count (ms)() -> (millisecond timer value=→"time9":u32)
            }
          }
        }
        frame 363 {
          # "Espera terminar a execução do comando atual \nantes de ir ao proximo passo da Observação."
          n622 = call-dynamic "Read Channel.vi"("error in (no error)"=w1631, "Acquisition in"=w1632) -> ("error out"=w1624:errorcluster, "Channel.lvclass"=w1625:refnum<class "Channel.lvclass">, "Acquisition out"=w1640:refnum<class "Acquisition.lvclass">)  [unwired: 7 in]
          n623 = call-dynamic "Read wait_expose.vi"("error in (no error)"=w1624, "Channel in"=w1625) -> ("error out"=w1622:errorcluster, "wait_expose"=w1620:bool, "Channel out"=w1623:refnum<class "Channel.lvclass">)  [unwired: 7 in]
          n624 = call-dynamic "Read State Machine.vi"("error in (no error)"=w1622, "Device in"=w1623) -> ("error out"=w1634:errorcluster, "State Machine.lvclass"=w1636:refnum<class "State Machine.lvclass">, "Device out"=w1638:refnum<class "Channel.lvclass">)  [unwired: 7 in]
          n625 = call-dynamic "Read State.vi"("error in (no error)"=w1634, "State Machine in"=w1636) -> ("error out"=w1633:errorcluster, "State"=w1616:i32, "State Machine out"=w1635:refnum<class "State Machine.lvclass">)  [unwired: 7 in]
          n626 = call-dynamic "Write State Machine.vi"("error in (no error)"=w1633, "State Machine.lvclass"=w1635, "Device in"=w1638) -> ("error out"=w1637:errorcluster, "Device out"=w1639:refnum<class "Channel.lvclass">)  [unwired: 7 in]
          n627 = Equal To 0?(x=w1616) -> (x = 0?=w1615:bool)
          n628 = call-dynamic "Write Channel.vi"("error in (no error)"=w1637, "Channel.lvclass"=w1639, "Acquisition in"=w1640) -> ("error out"=w1618:errorcluster, "Acquisition out"=w1630:refnum<class "Acquisition.lvclass">)  [unwired: 7 in]
          n629 = Increment(x=w1626) -> (x+1=w1619:u32)
          n630 = Select(t=w1619, s=w1615, f=w1626) -> (s? t:f=w1629:u32)
          n631 = call-dynamic "Write Acq_state.vi"("error in (no error)"=w1618, "Acq_state"=w1629, "Acquisition in"=w1630) -> ("error out"=w1627:errorcluster, "Acquisition out"=w1628:refnum<class "Acquisition.lvclass">)  [unwired: 7 in]
          n632 = Bundle By Name(cluster=w1617, "mode EXPOSE"=w1620) -> (w1621:refnum<class "S4GUI.lvclass">)
        }
        frame 364 {
          n633 = flat-sequence {
            tunnel: [w1656] -> w1644
            tunnel: w1645 -> [w1656]
            tunnel: [w1651] -> w1641
            frame #0 {
              n634 = local read "time9"() -> (w1652:u32)
              n635 = Tick Count (ms)() -> (millisecond timer value=w1655:u32)
              "time 10" <- w1655
              n636 = Subtract(x=w1655, y=w1652) -> (x-y=w1654:u32)
              "delay 89" <- w1654
              n637 = Greater?(x=w1654, y=u32 2000) -> (0:w1651:bool)
            }
          }
          n638 = Increment(x=w1642) -> (x+1=w1649:u32)
          n639 = Select(t=w1649, s=w1641, f=w1642) -> (s? t:f=w1650:u32)
          n640 = call-dynamic "Write Acq_state.vi"("error in (no error)"=w1644, "Acq_state"=w1650, "Acquisition in"=w1643) -> ("error out"=w1646:errorcluster, "Acquisition out"=w1647:refnum<class "Acquisition.lvclass">)  [unwired: 7 in]
        }
        frame 365 {
          # "Dispara o comando para o dispositivo corrente."
          n641 = call-dynamic "Read Channel.vi"("error in (no error)"=w1665, "Acquisition in"=w1666) -> ("error out"=w1672:errorcluster, "Channel.lvclass"=w1671:refnum<class "Channel.lvclass">, "Acquisition out"=w1676:refnum<class "Acquisition.lvclass">)  [unwired: 7 in]
          n642 = call-dynamic "Read State Machine.vi"("error in (no error)"=w1672, "Device in"=w1671) -> ("error out"=w1673:errorcluster, "State Machine.lvclass"=w1675:refnum<class "State Machine.lvclass">, "Device out"=w1669:refnum<class "Channel.lvclass">)  [unwired: 7 in]
          n643 = call "Next State.vi"("error in (no error)"=w1673, "New_State"=50, "State Machine in"=w1675) -> ("error out"=w1657:errorcluster, "State Machine out"=w1658:refnum<class "State Machine.lvclass">)  [unwired: 7 in]
          n644 = call-dynamic "Write State Machine.vi"("error in (no error)"=w1657, "State Machine.lvclass"=w1658, "Device in"=w1669) -> ("error out"=w1668:errorcluster, "Device out"=w1670:refnum<class "Channel.lvclass">)  [unwired: 7 in]
          n645 = Increment(x=w1667) -> (x+1=w1664:u32)
          n646 = call-dynamic "Write Channel.vi"("error in (no error)"=w1668, "Channel.lvclass"=w1670, "Acquisition in"=w1676) -> ("error out"=w1662:errorcluster, "Acquisition out"=w1661:refnum<class "Acquisition.lvclass">)  [unwired: 7 in]
          n647 = call-dynamic "Write Acq_state.vi"("error in (no error)"=w1662, "Acq_state"=w1664, "Acquisition in"=w1661) -> ("error out"=w1659:errorcluster, "Acquisition out"=w1660:refnum<class "Acquisition.lvclass">)  [unwired: 7 in]
        }
        frame 366 {
          # "Espera terminar a execução do comando atual \nantes de ir ao proximo passo da Observação."
          n648 = call-dynamic "Read Channel.vi"("error in (no error)"=w1694, "Acquisition in"=w1695) -> ("error out"=w1684:errorcluster, "Channel.lvclass"=w1685:refnum<class "Channel.lvclass">, "Acquisition out"=w1703:refnum<class "Acquisition.lvclass">)  [unwired: 7 in]
          n649 = call-dynamic "Read wait_expose.vi"("error in (no error)"=w1684, "Channel in"=w1685) -> ("error out"=w1682:errorcluster, "wait_expose"=w1680:bool, "Channel out"=w1683:refnum<class "Channel.lvclass">)  [unwired: 7 in]
          n650 = call-dynamic "Read State Machine.vi"("error in (no error)"=w1682, "Device in"=w1683) -> ("error out"=w1697:errorcluster, "State Machine.lvclass"=w1699:refnum<class "State Machine.lvclass">, "Device out"=w1701:refnum<class "Channel.lvclass">)  [unwired: 7 in]
          n651 = call-dynamic "Read State.vi"("error in (no error)"=w1697, "State Machine in"=w1699) -> ("error out"=w1696:errorcluster, "State"=w1688:i32, "State Machine out"=w1698:refnum<class "State Machine.lvclass">)  [unwired: 7 in]
          n652 = call-dynamic "Write State Machine.vi"("error in (no error)"=w1696, "State Machine.lvclass"=w1698, "Device in"=w1701) -> ("error out"=w1700:errorcluster, "Device out"=w1702:refnum<class "Channel.lvclass">)  [unwired: 7 in]
          n653 = Greater?(x=w1688, y=53) -> (0:w1687:bool)
          n654 = call-dynamic "Write Channel.vi"("error in (no error)"=w1700, "Channel.lvclass"=w1702, "Acquisition in"=w1703) -> ("error out"=w1678:errorcluster, "Acquisition out"=w1693:refnum<class "Acquisition.lvclass">)  [unwired: 7 in]
          n655 = Increment(x=w1686) -> (x+1=w1679:u32)
          n656 = Select(t=w1679, s=w1687, f=w1686) -> (s? t:f=w1692:u32)
          n657 = call-dynamic "Write Acq_state.vi"("error in (no error)"=w1678, "Acq_state"=w1692, "Acquisition in"=w1693) -> ("error out"=w1690:errorcluster, "Acquisition out"=w1691:refnum<class "Acquisition.lvclass">)  [unwired: 7 in]
          n658 = Bundle By Name(cluster=w1677, "mode EXPOSE"=w1680) -> (w1681:refnum<class "S4GUI.lvclass">)
        }
        frame 367 {
          # "SEQS_DONE = 0,1,2,...,n,0,1,..."
          n659 = Unbundle By Name(w1704) -> ("sequesDone"=w1713:u32, "cyclesDone"=w1708:u32)
          n660 = call-dynamic "Read Channel.vi"("error in (no error)"=w1724, "Acquisition in"=w1725) -> ("error out"=w1716:errorcluster, "Channel.lvclass"=w1717:refnum<class "Channel.lvclass">, "Acquisition out"=w1726:refnum<class "Acquisition.lvclass">)  [unwired: 7 in]
          n661 = call-dynamic "Read CyclesDone.vi"("error in (no error)"=w1716, "Channel in"=w1717) -> ("error out"=w1718:errorcluster, "CyclesDone"=w1709:u32, "Channel out"=w1719:refnum<class "Channel.lvclass">)  [unwired: 7 in]
          n662 = call-dynamic "Read SequesDone.vi"("error in (no error)"=w1718, "Channel in"=w1719) -> ("error out"=w1714:errorcluster, "SequesDone"=w1710:u32, "Channel out"=w1715:refnum<class "Channel.lvclass">)  [unwired: 6 in, 1 out]
          n663 = Not Equal?(x=w1709, y=w1708) -> (x != y?=w1706:bool)
          n664 = Not Equal?(x=w1710, y=w1713) -> (x != y?=w1707:bool)
          n665 = call-dynamic "Write Channel.vi"("error in (no error)"=w1714, "Channel.lvclass"=w1715, "Acquisition in"=w1726) -> ("error out"=w1722:errorcluster, "Acquisition out"=w1723:refnum<class "Acquisition.lvclass">)  [unwired: 7 in]
          n666 = Or(x=w1707, y=w1706) -> (x .or. y?=w1705:bool)
          n667 = case shown="True" w1705 {
            tunnel: [w1727 w1728] -> w1712
            tunnel: w1711 -> [w1727 w1729]
            tunnel: w1710 -> [_ _]
            tunnel: w1709 -> [_ _]
            frame False {
            }
            frame True {
              n668 = Increment(x=w1729) -> (x+1=w1728:u32)
            }
          }
          n669 = call-dynamic "Write Acq_state.vi"("error in (no error)"=w1722, "Acq_state"=w1712, "Acquisition in"=w1723) -> ("error out"=w1720:errorcluster, "Acquisition out"=w1721:refnum<class "Acquisition.lvclass">)  [unwired: 7 in]
        }
        frame 368 {
          n670 = Unbundle By Name(w1737) -> ("TelFocus.lvclass"=w1739:refnum<class "TelFocus.lvclass">)
          n671 = call-dynamic "VerifSteps.vi"("error in (no error)"=w1736, "TelFocus in"=w1739) -> ("error out"=w1733:errorcluster, "continua?"=w1740:bool, "TelFocus out"=w1738:refnum<class "TelFocus.lvclass">)  [unwired: 7 in]
          n672 = Bundle By Name(cluster=w1737, "TelFocus.lvclass"=w1738) -> (w1732:refnum<class "S4GUI.lvclass">)
          n673 = Select(t=u32 360, s=w1740, f=u32 0) -> (s? t:f=w1734:u32)
          n674 = call-dynamic "Write Acq_state.vi"("error in (no error)"=w1733, "Acq_state"=w1734, "Acquisition in"=w1735) -> ("error out"=w1730:errorcluster, "Acquisition out"=w1731:refnum<class "Acquisition.lvclass">)  [unwired: 7 in]
        }
        frame 400 {
          # "Estado de \"Pause\": fica parado aqui até o botão START seja pressionado."
        }
        frame 500 {
          # "Espera terminar o envio de RESUME para todos os ACS."
          # "Estado de \"Pause\": fica parado aqui até o botão RESUME seja pressionado."
          n675 = call-dynamic "VerifyAcqIdle.vi"("error in (no error)"=w1747, "S4GUI in"=w1748) -> ("error out"=w1751:errorcluster, "idle"=w1753:bool, "S4GUI out"=w1752:refnum<class "S4GUI.lvclass">)  [unwired: 7 in]
          n676 = case shown="True" w1753 {
            tunnel: w1752 -> [w1755 w1765]
            tunnel: [w1755 w1757] -> w1750
            tunnel: w1751 -> [w1754 w1764]
            tunnel: [w1754 w1758] -> w1749
            frame False {
            }
            frame True {
              n677 = call-dynamic "LoadPrevAcqRunState.vi"("error in (no error)"=w1764, "S4GUI in"=w1765) -> ("error out"=w1759:errorcluster, "S4GUI out"=w1760:refnum<class "S4GUI.lvclass">)  [unwired: 8 in]
              n678 = Tick Count (ms)() -> (millisecond timer value=w1756:u32)
              n679 = call-dynamic "Read Obs_prevstate.vi"("error in (no error)"=w1759, "S4ACS_GUI in"=w1760) -> ("error out"=w1763:errorcluster, "Obs_prevstate"=w1761:u32, "S4ACS_GUI out"=w1762:refnum<class "S4GUI.lvclass">)  [unwired: 7 in]
              n680 = local write "time307"(w1756) -> ()
              n681 = local write "time1"(w1756) -> ()
              n682 = call-dynamic "Write Obs_state.vi"("error in (no error)"=w1763, "Obs_state"=w1761, "S4ACS_GUI in"=w1762) -> ("error out"=w1758:errorcluster, "S4ACS_GUI out"=w1757:refnum<class "S4GUI.lvclass">)  [unwired: 7 in]
            }
          }
        }
      }
    }
    frame Error {
    }
  }
  "error out" <- w5
  "S4ACS_GUI out" <- w3
  "Acquisition.lvclass Out" <- w1
